vi "TLB Native Dynamic Events ver 0.21.vi"() -> ()   [LabVIEW 2018]
uses:
  Labview Training Phase 2/Enum Controls/States for Action Engine.ctl
  TLB Type Definitions/State Type Definitions, for 0.26d versions and later.ctl
  TLB Type Definitions/Intruction Type Definitions.ctl
  TLB Type Definitions/Encoder cluster.ctl
  TLB Type Definitions/PING CLUSTER.ctl
  <vilib>/Studica/Studica Toolkit/NavX/NavX.lvlib
  <vilib>/Studica/Studica Toolkit/Background/DIO Channel.ctl
  Underlying VI's/NavX VI/navX type def.ctl
  <vilib>/Studica/Studica Toolkit/Background/I2C Channel.ctl
  TLB Type Definitions/Vision cluster.ctl
  <vilib>/NI_Real-Time Target Support.lvlib
  TLB Type Definitions/Stepper cluster.ctl
  Experimental VI's/Archived VI's/MOTOR CONTROL NO PID Type Def.ctl
  Underlying VI's/I2C Master VI/I2C MASTER Type Def.ctl
  Underlying VI's/I2C Master VI/I2C_MASTER_WRITE_NEW Type Def.ctl
  <vilib>/userdefined/High Color/IMAQdx.ctl
  Underlying VI's/I2C Master VI/Arduino_Interfacing.ctl
  TLB Type Definitions/Yaw Cluster.ctl
  TLB Type Definitions/Time cluster.ctl
  TLB Type Definitions/Y Stepper cluster.ctl
  Underlying VI's/Modified webcam FGV/Webcam AE.ctl
  Underlying VI's/Elasped Timer/Elapsed timer control.ctl
  Underlying VI's/Motor Control VI with PID/MOTOR CONTROL WITH PID AE DATA MODE TYPE DEF.ctl
  Underlying VI's/Motor Control VI with PID/MOTOR CONTROL WITH PID AE DIRECTION TYPE DEF.ctl
  TLB Type Definitions/IR Sensor Type Def.ctl
  <vilib>/myRIO/Common/Instrument Driver Framework/myRIO v1.0/AI/typedefs/AI Channels Enum.ctl
  <vilib>/myRIO/Common/Instrument Driver Framework/myRIO v1.0/AI/typedefs/AI Channels List.ctl
  TLB Type Definitions/Motor Speed Cluster.ctl
  Underlying VI's/IMAQ Create Reference AE/IMAQ Reference AE.ctl
  TLB Type Definitions/Line Sensor Cluster.ctl
  Underlying VI's/Line Sensor AE/Line Sensor AE Type Def.ctl
  <vilib>/Utility/RT CPU Load.ctl
  <vilib>/Studica/Studica Toolkit/NavX/TypeDefs/Flags/Z900_navX_Flags_CalibrationStatusTypeDef.ctl
  <vilib>/Studica/Studica Toolkit/NavX/TypeDefs/Flags/Z900_navX_Flags_OpStatusTypeDef.ctl
panel:
  out "Selected Task":T1=enum."Start Task 9"
  out "Object recognition mode":enum16{"Ball", "Soap", "Gel", "Pipe", "None"}(ring)
  out "Distance reached?":bool
  out "Correcte stepper":u8
  out "Image Processing Error":errorcluster
  out "Object Detection":T2
  out "Status":T5 {"OP Status" items=["INITIALIZING", "SELFTEST_IN_PROGRESS", "ERROR", "IMU_AUTOCAL_IN_PROGRESS", "NORMAL"]; "Calibration Status" items=["IMU_CAL_STATE_MASK"=3, "IMU_CAL_STATE_INPROGRESS"=0, "IMU_CAL_STATE_ACCUMULATE"=1, "IMU_CAL_STATE_COMPLETE"=2]}
  out "General Errors":errorcluster
  in  "Red LED":bool
  out "Arm IR Sensor":dbl
  out "Table obstruct":bool
  out "x-y":dbl
  out "Left IR Sensor":dbl
  out "Obstacle detected":bool
  out "Speed & distance":T6
  out "Time up flag":bool
  out "Task selection":u8
  out "NavX Readings":T7
  out "Arduino Data":T8
  out "CPU loads":T9[](array[typedef]) {"ISR (%)" format="%#.2f"; "Idle (%)" format="%#.2f"; "Background (%)" format="%#.2f"; "Normal (%)" format="%#.2f"; "Above Normal (%)" format="%#.2f"; "High (%)" format="%#.2g"; "Timed Structures (%)" format="%#.2g"; "Time Critical (%)" format="%#.2g"; "Total (%)" format="%#.2g"}
  out "TASK ENABLE":bool
  out "Rising Edge":bool
  in  "Green LED":bool
  out "State Logic":T10=enum."Startup"
  out "elements":T1[](array[typedef])
  in  "STOP TASK":bool
  in  "OK Button":bool
  in  "STOP":bool
  out "Queue Errors":errorcluster
  out "Action Queue Items":i32
  out "State Logic Queue Items":i32
  out "Action Queues items":string[](array[string])=["Hardware reset", "Software reset", ""]
  out "Action State":string
  # "System Health Status Update"
  # "VISION"
  # "TLB FRAMEWORK STATUS"
  # "Test Programme written by Calvin Loke    Dated: 28 Aug 2019\nTest Programme revised by Dr Alex See   Dated 30 Aug 2019\n\nRevision date: 20/03/2020\nProgramme version:   TLB Native Dynamic Events ver 0.19a"
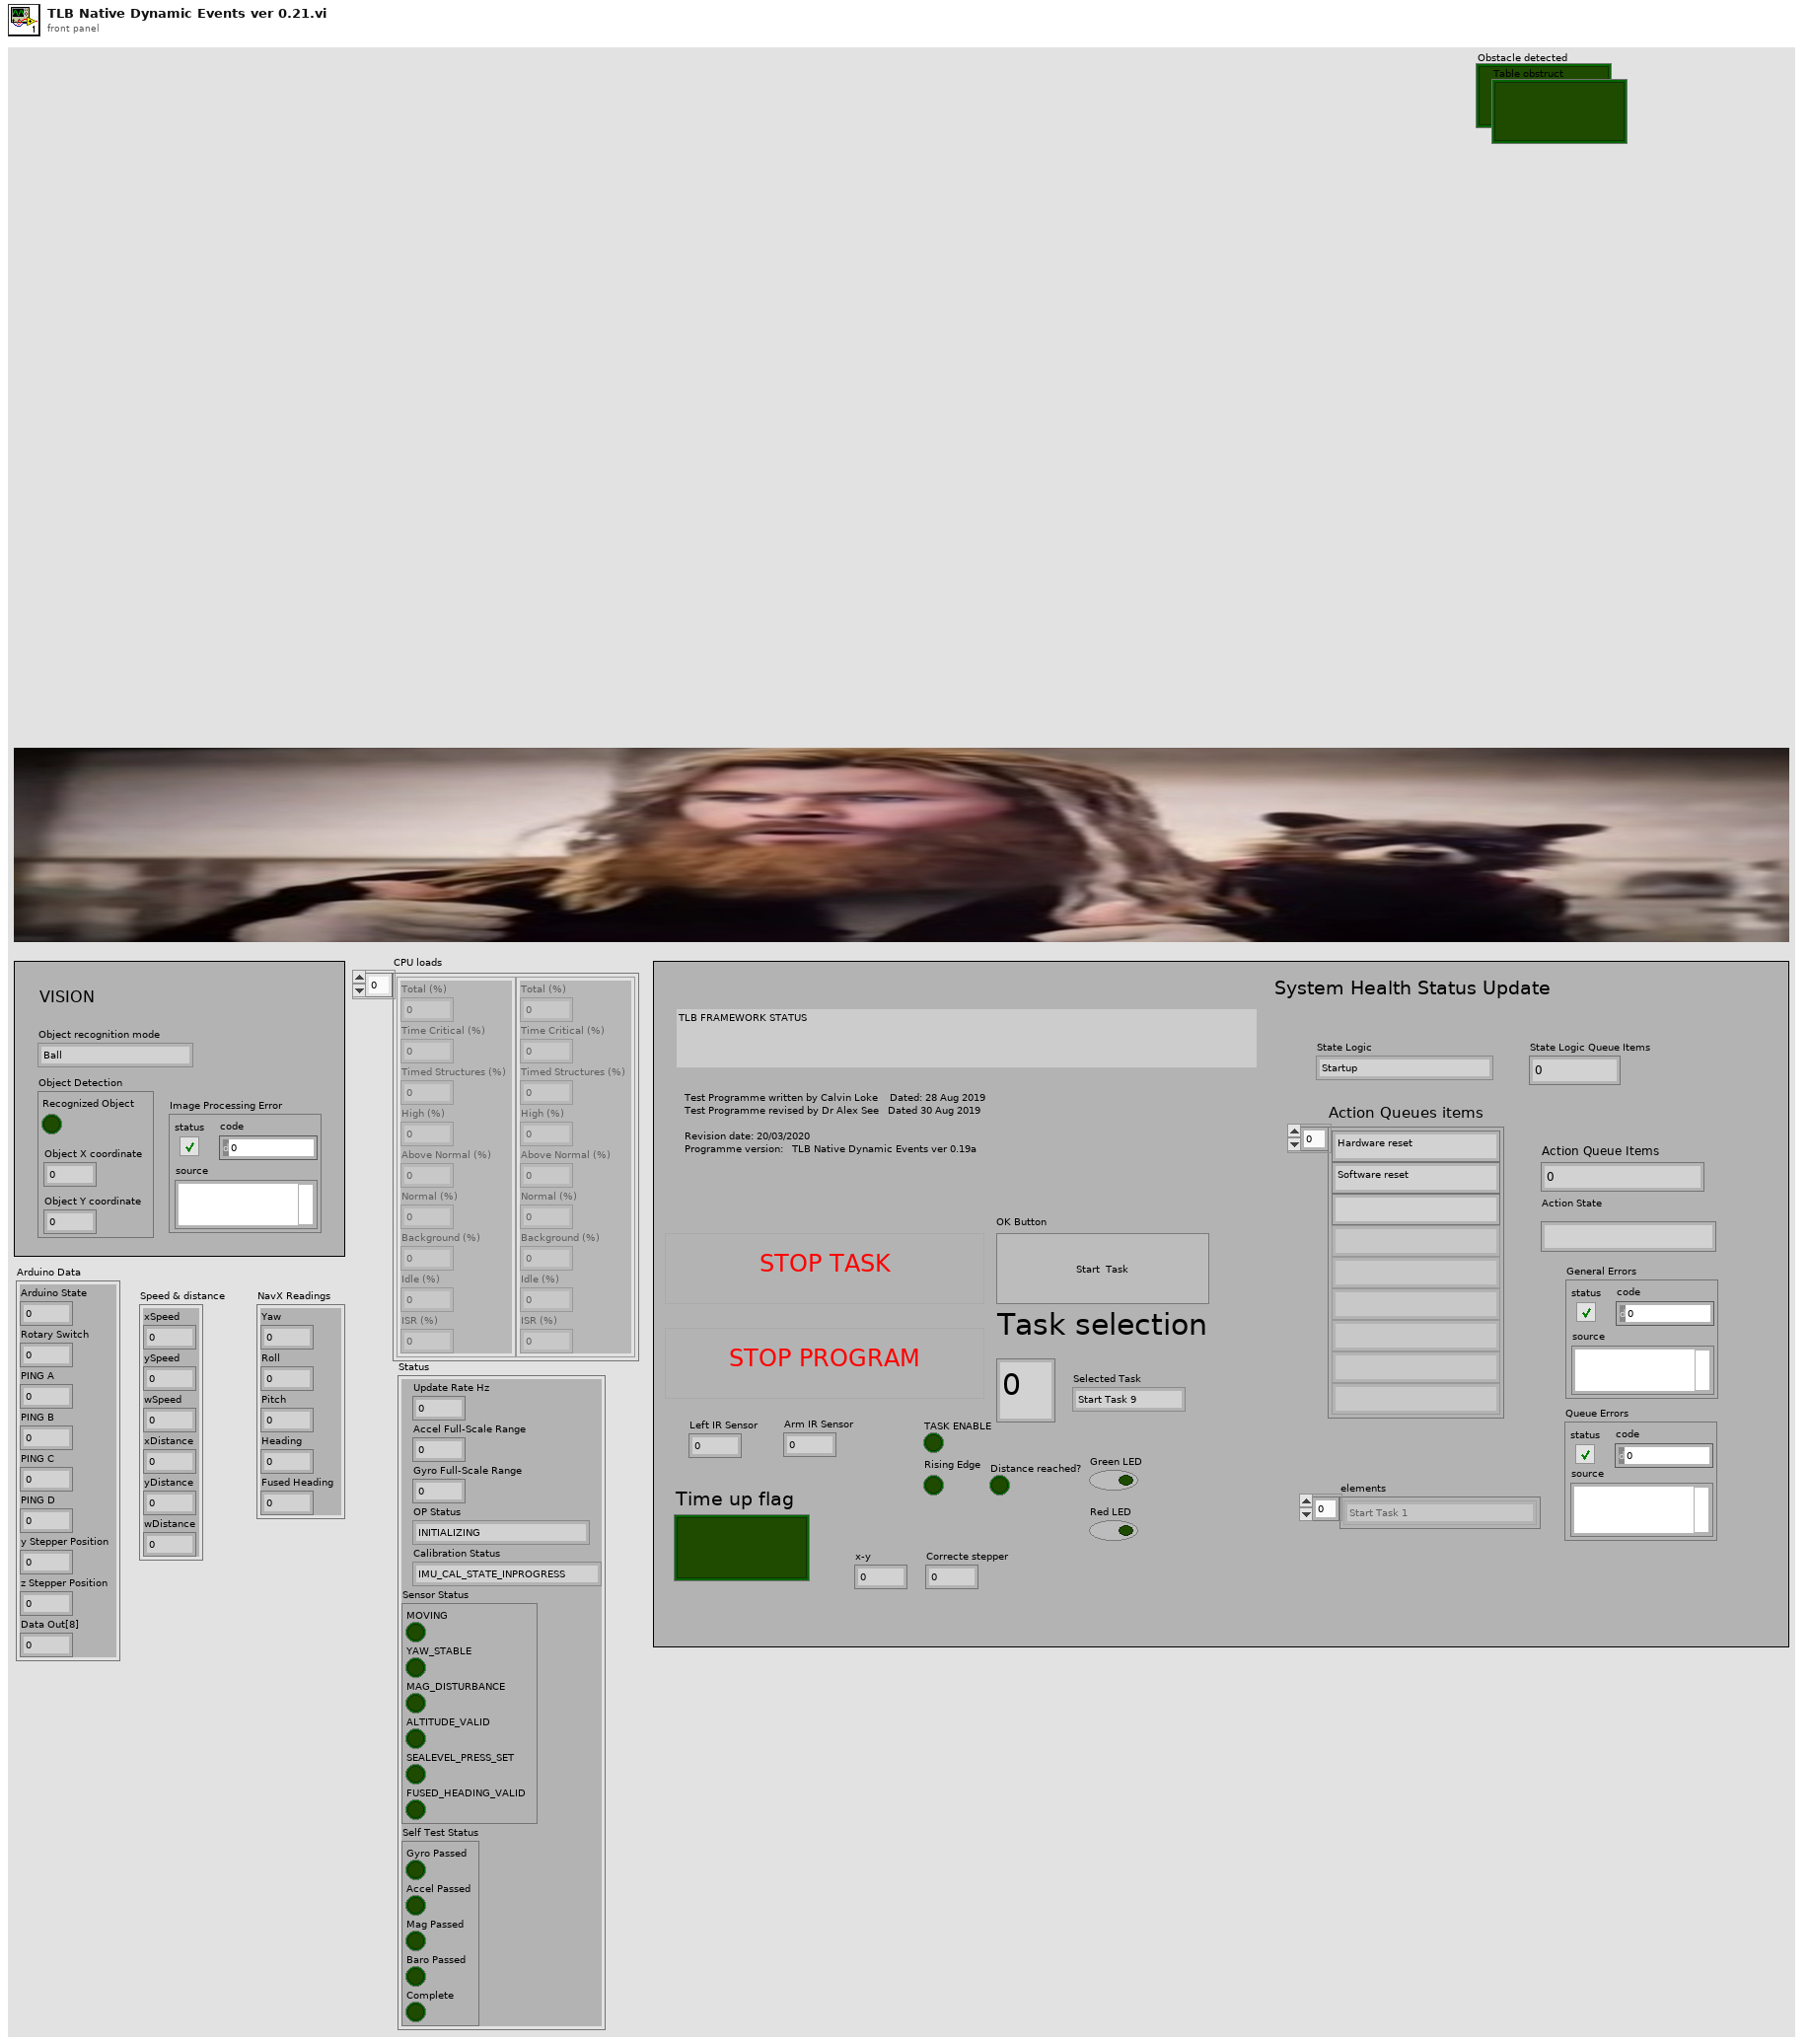
[diagram p1: front panel]
types:
  T1 = typedef "Intruction Type Definitions.ctl" = enum16{"None", "Start Task 1", "Start Task 2", "Start Task 3", "Start Task 4", "Start Task 5", "Start Task 6", "Start Task 7", "Start Task 8 - BALL", "Start Task 8 - Gel", "Start Task 8 - Pipe", "Start Task 8 - Soap", "Start Task 9", "Start Task A", "Start Task B", "Exit"}
  T2 = typedef "Vision cluster.ctl" = cluster{"Recognized Object":bool, "Object X coordinate":dbl, "Object Y coordinate":dbl}
  T3 = typedef "NavX.lvlib/Z900_navX_Flags_OpStatusTypeDef.ctl" = u8
  T4 = typedef "NavX.lvlib/Z900_navX_Flags_CalibrationStatusTypeDef.ctl" = u8
  T5 = cluster{"Update Rate Hz":u8, "Accel Full-Scale Range":u8, "Gyro Full-Scale Range":u16, "OP Status":T3, "Calibration Status":T4, "Sensor Status":cluster{"MOVING":bool, "YAW_STABLE":bool, "MAG_DISTURBANCE":bool, "ALTITUDE_VALID":bool, "SEALEVEL_PRESS_SET":bool, "FUSED_HEADING_VALID":bool}, "Self Test Status":cluster{"Gyro Passed":bool, "Accel Passed":bool, "Mag Passed":bool, "Baro Passed":bool, "Complete":bool}}
  T6 = cluster{"xSpeed":dbl, "ySpeed":dbl, "wSpeed":dbl, "xDistance":dbl, "yDistance":dbl, "wDistance":dbl}
  T7 = cluster{"Yaw":dbl, "Roll":dbl, "Pitch":dbl, "Heading":dbl, "Fused Heading":dbl}
  T8 = cluster{"Arduino State":u8, "Rotary Switch":u8, "PING A":u8, "PING B":u8, "PING C":u8, "PING D":u8, "y Stepper Position":u8, "z Stepper Position":u8, "Data Out[8]":u8}
  T9 = typedef "NI_Real-Time Target Support.lvlib/RT CPU Load.ctl" = cluster{"Total (%)":dbl, "Time Critical (%)":dbl, "Timed Structures (%)":dbl, "High (%)":dbl, "Above Normal (%)":dbl, "Normal (%)":dbl, "Background (%)":dbl, "Idle (%)":dbl, "ISR (%)":dbl}
  T10 = typedef "State Type Definitions.ctl" = enum16{"None", "Startup", "Move to Angle", "True Stop", "Idle", "Shutdown", "Task 1A", "Task 1B", "Task 2:Raise Arm", "Task 2:Sensor Mode", "Task 2:Reverse Mode", "Task 3", "Task 4_A", "Task 4_B", "Task 4_C", "Task 4_D", "Task 5A", "Task 5B", "Task 5C", "Task 5D", "Task 5E: POSITION ARM", "Task 5F: ARM GRAB HEIGHT", "Task 5G: CLOSE CLAW", "Task 5H: RAISE ARM", "Task 6_A", "Task 6_B", "Task 7", "Task 8A: RAISE ARM", "Task 8B: MOVE TO BOX", "Task 8C: CAM BURST", "Task 8D: PROCESS IMAGE", "Task 8E: ROBOT ADJUST", "Task 8F: CAM BURST 2", "Task 8G: PROCESS IMAGE 2", "Task 8H: ARM ADJUST", "Task 8I: ARM GRAB HEIGHT", "Task 8J: CLOSE CLAW", "Task 8K: RAISE MY SWORD", "Task 9A: Raise Arm", "Task 9B: Rotate to Angle", "Task 9C: Detect Box", "Task 9D: MOVE FORWARD", "Task 9E: MOVE LEFT", "Task 9F: SCAN IMAGE", "Task 9G: PROCESS COLOUR", "Task 9H: MOVE RIGHT", "Task 9I: SCAN IMAGE", "Task 9J: PROCESS COLOUR", "Task 9K: ROTATE 90 CW", "Task 9L: MOVE FORWARD", "Task 9M: MOVE RIGHT", "Task 9N: SCAN IMAGE", "Task 9O: PROCESS COLOUR", "Task 9P: MOVE RIGHT", "Task 9Q: SCAN IMAGE", "Task 9R: PROCESS COLOUR", "Task A1: Raise Arm", "Task A2: Rotate to Angle", "Task A3: Move Forward", "Task A4: Rotate CW 90"}
  T11 = typedef "Line Sensor Cluster.ctl" = cluster{"Line Detected?":bool, "S1":dbl, "S2":dbl, "S3":dbl, "S4":dbl}
  T12 = typedef "Motor Speed Cluster.ctl" = cluster{"ySpeed":dbl, "xSpeed":dbl, "wSpeed":dbl}
  T13 = typedef "IR Sensor Type Def.ctl" = cluster{"Left IR Sensor":dbl, "Arm IR Sensor":dbl, "Bottom IR Sensor":dbl}
  T14 = typedef "Y Stepper cluster.ctl" = cluster{"yStepper desired":u8}
  T15 = typedef "Time cluster.ctl" = cluster{"Time up flag":bool, "SET TIME TO CHECK":dbl}
  T16 = typedef "Yaw Cluster.ctl" = cluster{"Yaw":dbl, "Compass":dbl}
  T17 = typedef "Stepper cluster.ctl" = cluster{"y Stepper Position":u8, "z Stepper Position":u8}
  T18 = typedef "DIO Channel.ctl" = enum16{"Not Connected", "A/DIO1", "A/DIO2", "A/DIO3", "A/DIO4", "A/DIO5", "A/DIO6", "A/DIO7", "A/DIO13", "B/DIO1", "B/DIO2", "B/DIO3", "B/DIO4", "B/DIO5", "B/DIO6", "B/DIO7", "B/DIO13", "C/DIO0", "C/DIO1", "C/DIO2", "C/DIO3", "C/DIO4", "C/DIO5", "C/DIO6", "C/DIO7"}
  T19 = typedef "PING CLUSTER.ctl" = cluster{"PING_A":u8, "PING_B":u8, "PING_C":u8, "PING_D":u8}
  T20 = typedef "Encoder cluster.ctl" = cluster{"xDistance":dbl, "yDistance":dbl, "wDistance":dbl}
  T21 = cluster{"DIO Channel":T18, "FPGA VI Reference Out":refnum<k20>}
  T22 = typedef "navX type def.ctl" = enum16{"Get i2C reference", "Read Values", "Zero Yaw"}
  T23 = typedef "Arduino_Interfacing.ctl" = enum16{"Initialize", "Write to Arduino", "Read From Arduino"}
  T24 = typedef "I2C Channel.ctl" = enum16{"Not Connected", "A", "B"}
  T25 = typedef "States for Action Engine.ctl" = enum16{"Initialize", "Write", "Read"}
  T26 = cluster{"I2C Ref Out":cluster{"I2C Channel":T24, "FPGA VI Reference Out":refnum<k20>}, "Connected":bool, "Slave Address (7-bit)":u8, "Registry":u8[]}
  T27 = typedef "State Type Definitions.ctl" = enum16{"None", "Startup", "Move to Angle", "True Stop", "Idle", "Shutdown", "Task 1", "Task 2:Raise Arm", "Task 2:Sensor Mode", "Task 2:Reverse Mode", "Task 3", "Task 4_A", "Task 4_B", "Task 4_C", "Task 4_D", "Task 5A: ARM CAM HEIGHT", "Task 5B: MOVE TO BOX", "Task 5C: CAM BURST", "Task 5D: PROCESS IMAGE", "Task 5E: POSITION ARM", "Task 5F: ARM GRAB HEIGHT", "Task 5G: CLOSE CLAW", "Task 5H: RAISE ARM", "Task 6_A", "Task 6_B", "Task 7", "Task 8A: RAISE ARM", "Task 8B: MOVE TO BOX", "Task 8C: CAM BURST", "Task 8D: PROCESS IMAGE", "Task 8E: ROBOT ADJUST", "Task 8F: CAM BURST 2", "Task 8G: PROCESS IMAGE 2", "Task 8H: ARM ADJUST", "Task 8I: ARM GRAB HEIGHT", "Task 8J: CLOSE CLAW", "Task 8K: RAISE MY SWORD", "Task 9A: Raise Arm", "Task 9B: Rotate to Angle", "Task 9C: Rotation alignmnet", "Task 9D: Move Forward", "Task 9E: MOVE LEFT", "Task A: RAISE ARM TO HEIGHT", "Task A: MOVE FORWARD"}
  T28 = typedef "MOTOR CONTROL WITH PID AE DIRECTION TYPE DEF.ctl" = enum16{"y-axis movement", "x-axis movement", "rotation", "stop", "reset encoders"}
  T29 = typedef "MOTOR CONTROL WITH PID AE DATA MODE TYPE DEF.ctl" = enum16{"Init AE", "Write to AE", "Read from AE"}
  T30 = typedef "Line Sensor AE Type Def.ctl" = enum16{"INIT AE", "READ FROM LINE SENSORS"}
  T31 = typedef "IMAQ Reference AE.ctl" = enum16{"Initialize AE", "Get IMAQ Reference", "Dispose Processing Buffer"}
  T32 = typedef "Elapsed timer control.ctl" = enum16{"Start", "Pause", "Initialize"}
  T33 = typedef "I2C_MASTER_WRITE_NEW Type Def.ctl" = enum16{"Ultrasonic sensors", "Stepper origin", "zStepper 13.3k", "zStepper 13k", "zStepper 12k", "zStepper 11k", "zStepper 10k", "zStepper 9k", "zStepper 8k", "zStepper 7k", "zStepper 6k", "zStepper 5k", "zStepper 4k", "zStepper 3k", "zStepper 2k", "zStepper 1k", "zStepper 900", "zStepper 800", "zStepper 700", "zStepper 600", "zStepper 500", "zStepper 400", "zStepper 300", "zStepper 200", "zStepper 100", "zStepper 0", "yStepper control", "Open Claw", "Close Claw", "Soft Reset"}
  T34 = typedef "Webcam AE.ctl" = enum16{"Initialize Camera", "Open Camera", "Continuous Acquisition", "Close Camera", "Retrieve Image", "Dispose Camera Image Buffer"}
  T35 = typedef "IMAQdx.ctl" = refnum<k21>
  T36 = typedef "MOTOR CONTROL NO PID Type Def.ctl" = enum16{"Init", "Front Back", "Left Right", "Rotate", "Stop", "Latch"}
  T37 = typedef "AI Channels List.ctl" = T38[]
  T38 = typedef "AI Channels Enum.ctl" = enum16{"Not Connected", "AudioIn/Left", "AudioIn/Right", "C/AI0", "C/AI1", "A/AI0", "A/AI1", "A/AI2", "A/AI3", "A/AI4", "A/AI5", "A/AI6", "A/AI7", "B/AI0", "B/AI1", "B/AI2", "B/AI3", "B/AI4", "B/AI5", "B/AI6", "B/AI7", "AI/AI0", "AI/AI1", "AI/AI2", "AI/AI3", "A/AI0 (DIFF)", "A/AI1 (DIFF)", "A/AI2 (DIFF)", "A/AI3 (DIFF)", "B/AI0 (DIFF)", "B/AI1 (DIFF)", "B/AI2 (DIFF)", "B/AI3 (DIFF)"}
  T39 = cluster{"S1":dbl, "S2":dbl, "S3":dbl, "S4":dbl, "Array[4]":dbl, "Array[5]":dbl, "Array[6]":dbl, "Array[7]":dbl, "Array[8]":dbl}
  T40 = typedef "I2C MASTER Type Def.ctl" = enum16{"Last State", "Mode 0", "Mode 1", "Mode 2", "Mode 3", "Mode 4", "Mode 5", "Mode 6", "Mode 7", "Mode 8", "Mode 9", "Mode 10"}
  T41 = typedef "IMAQ Image.ctl" = refnum<image>
  T42 = cluster{"Number of Matches":i32, "Object detected?":bool}
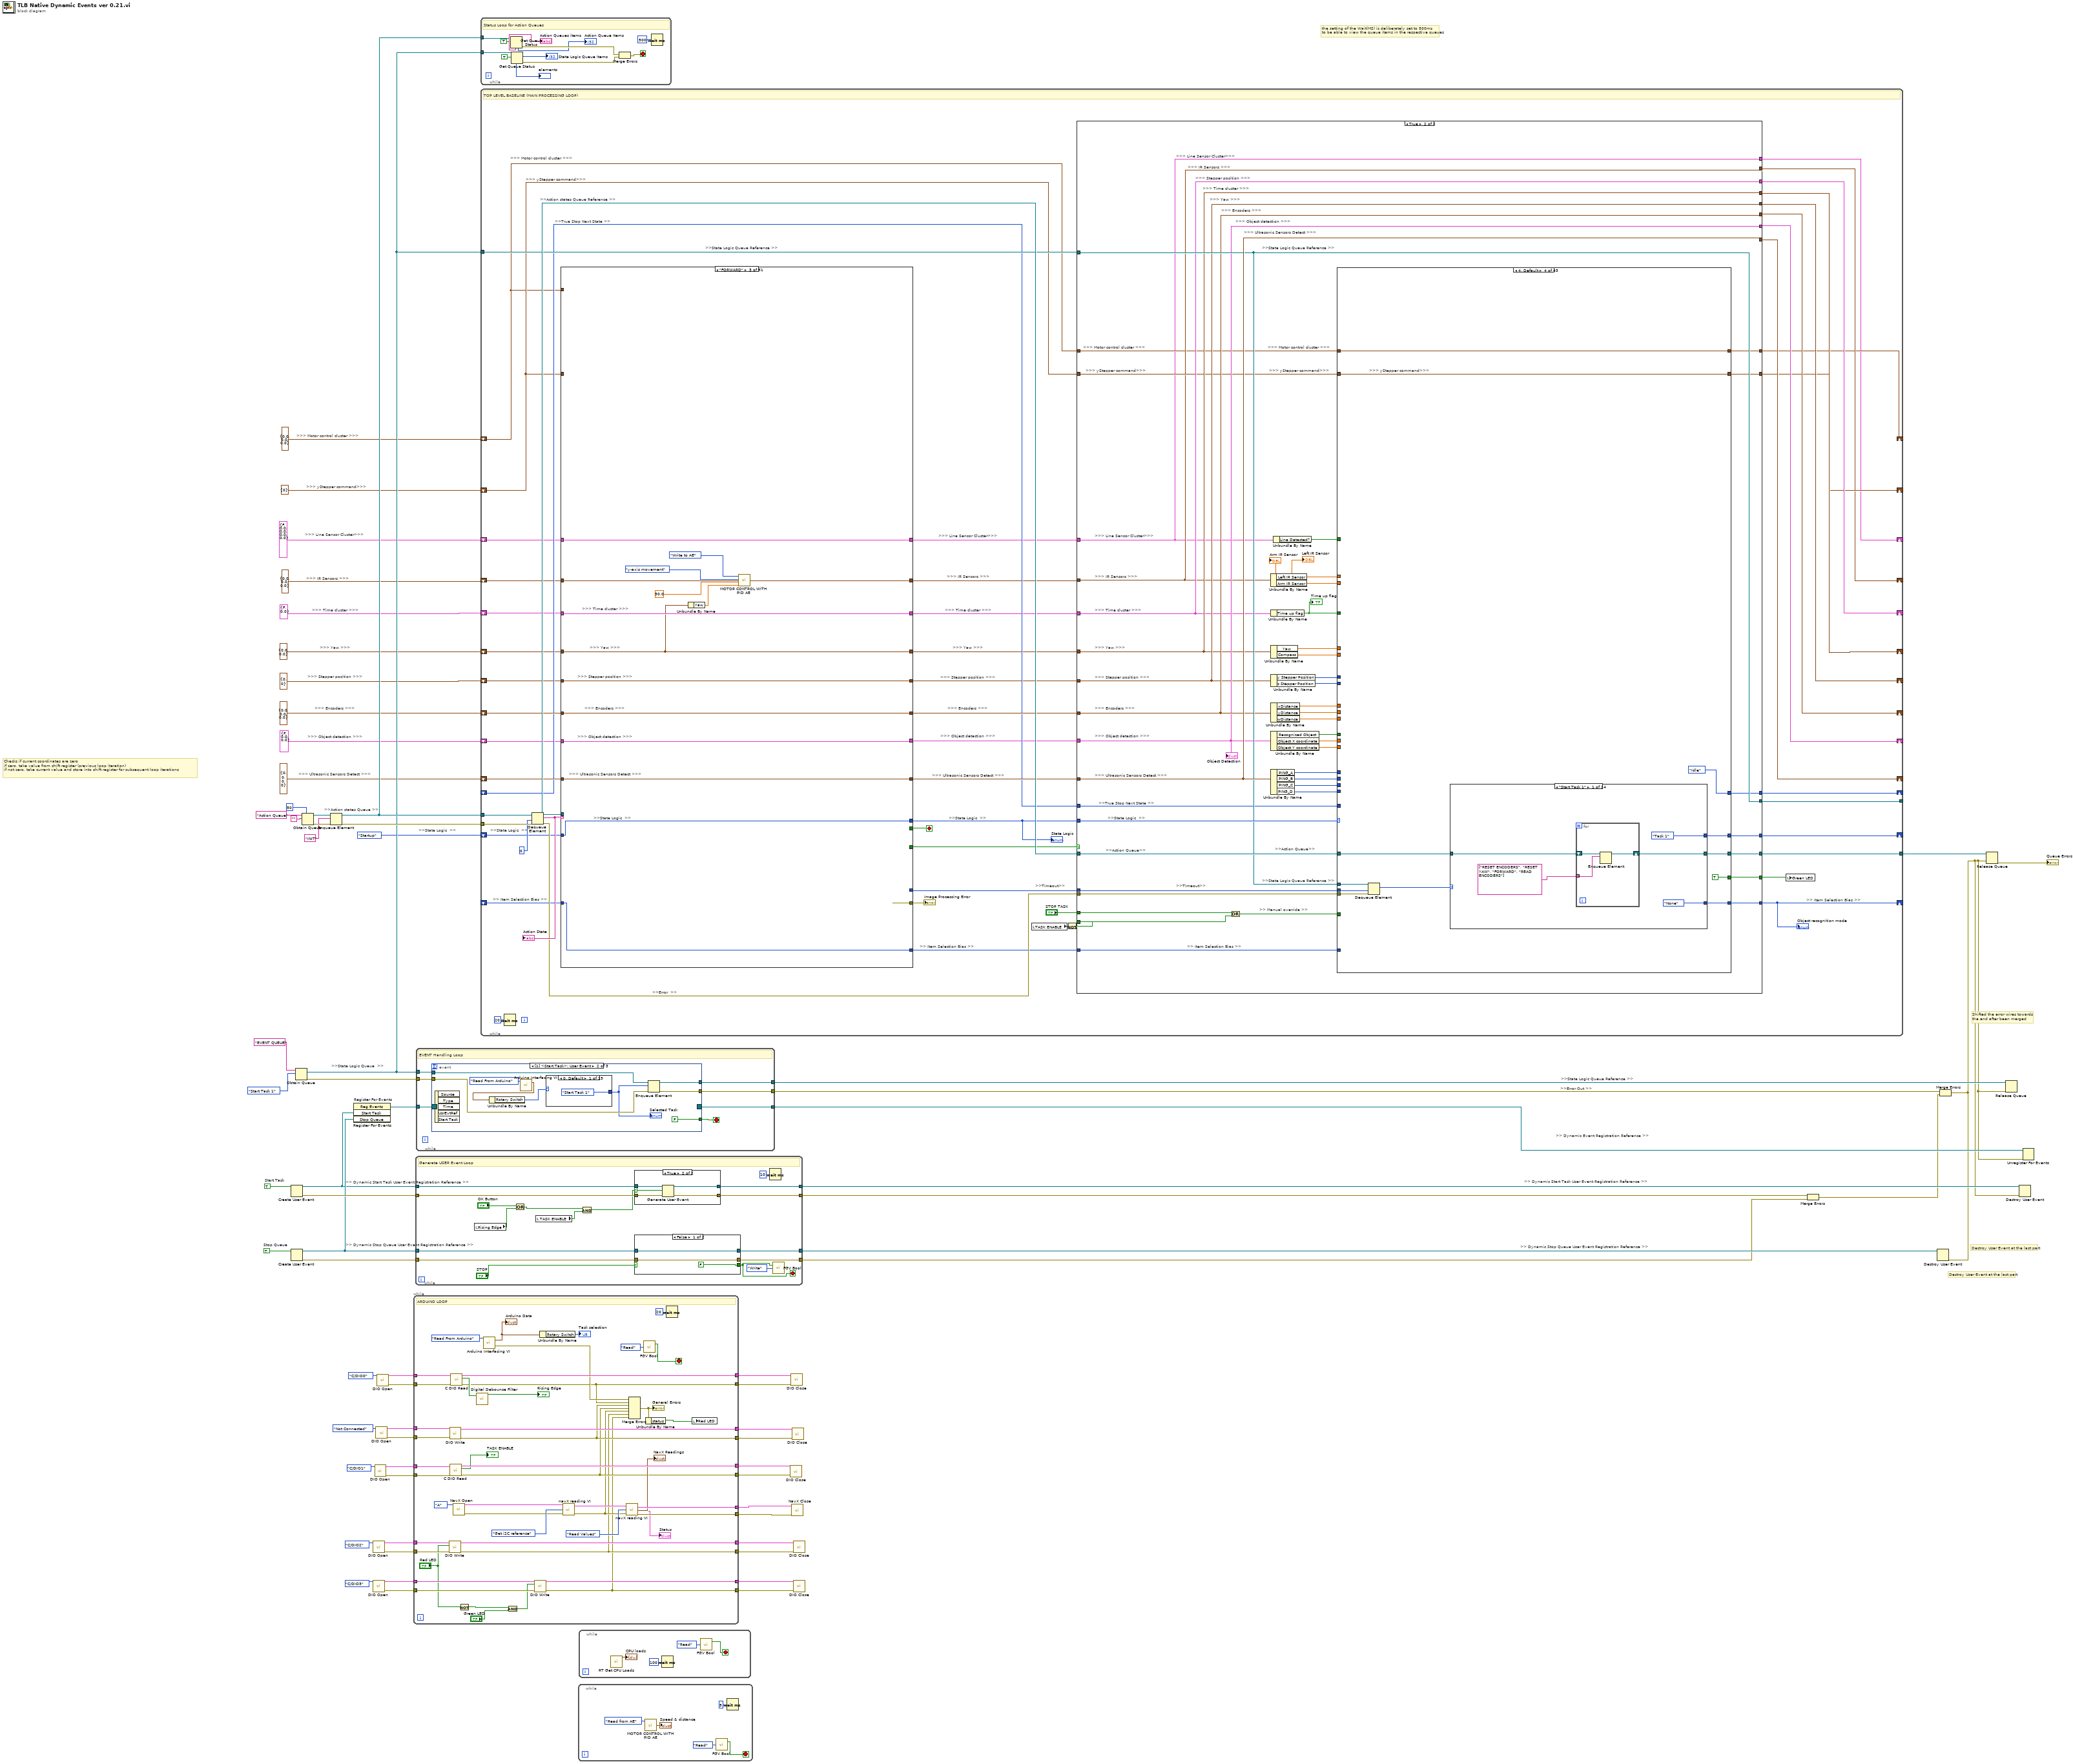
[diagram p0: block diagram]
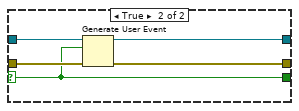
[diagram p2: hidden frame]
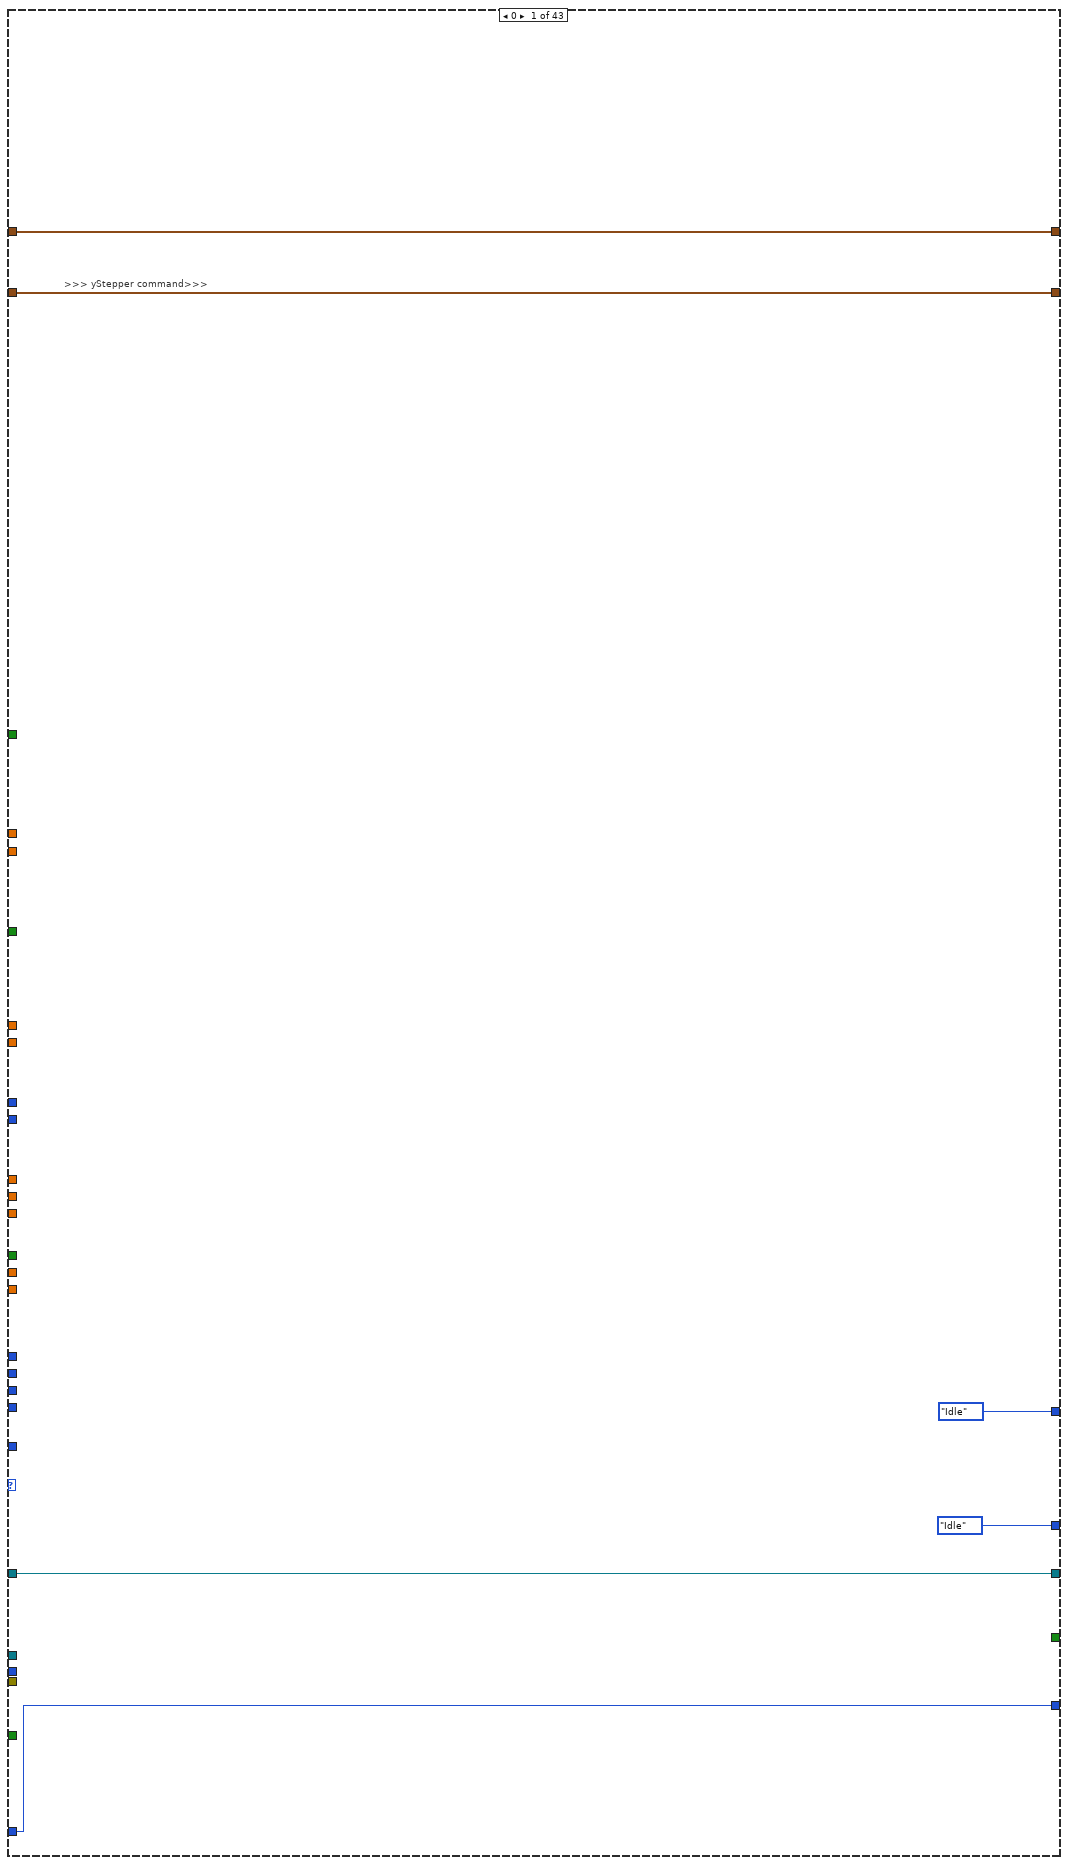
[diagram p5: hidden frame]
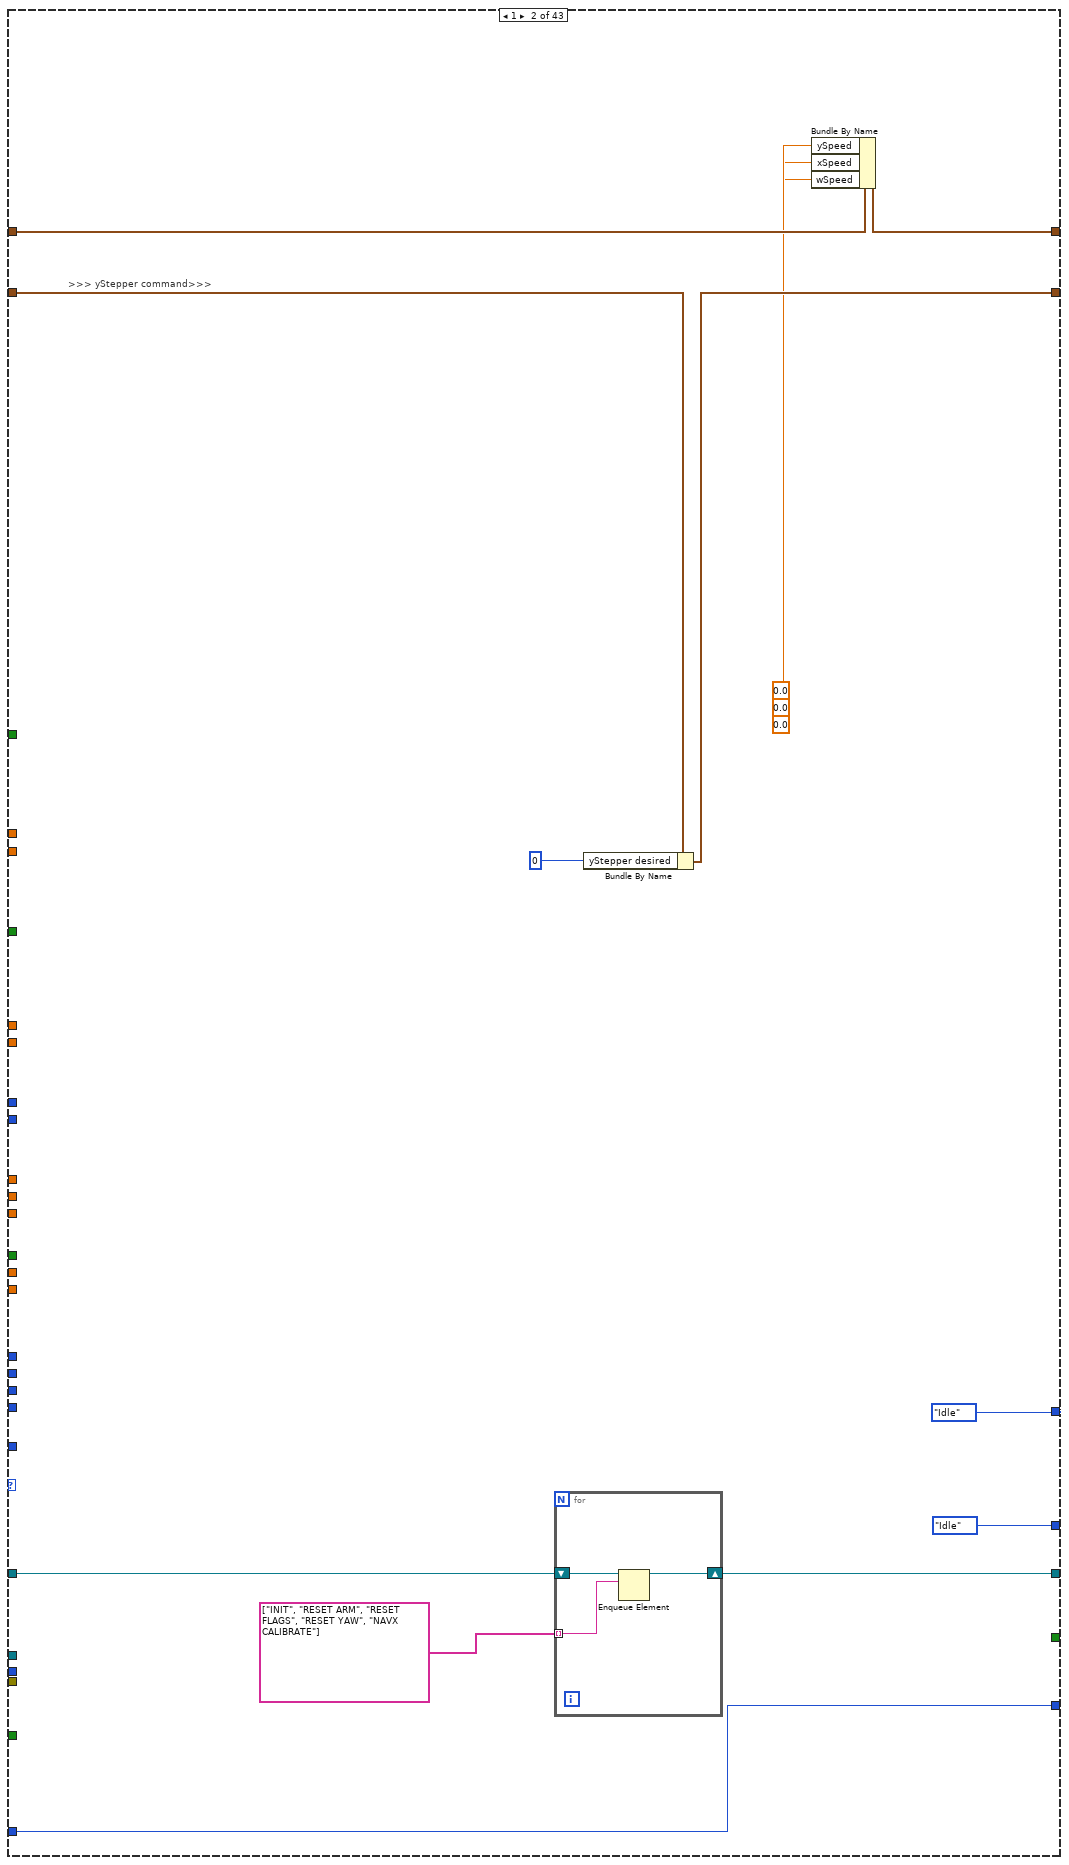
[diagram p6: hidden frame]
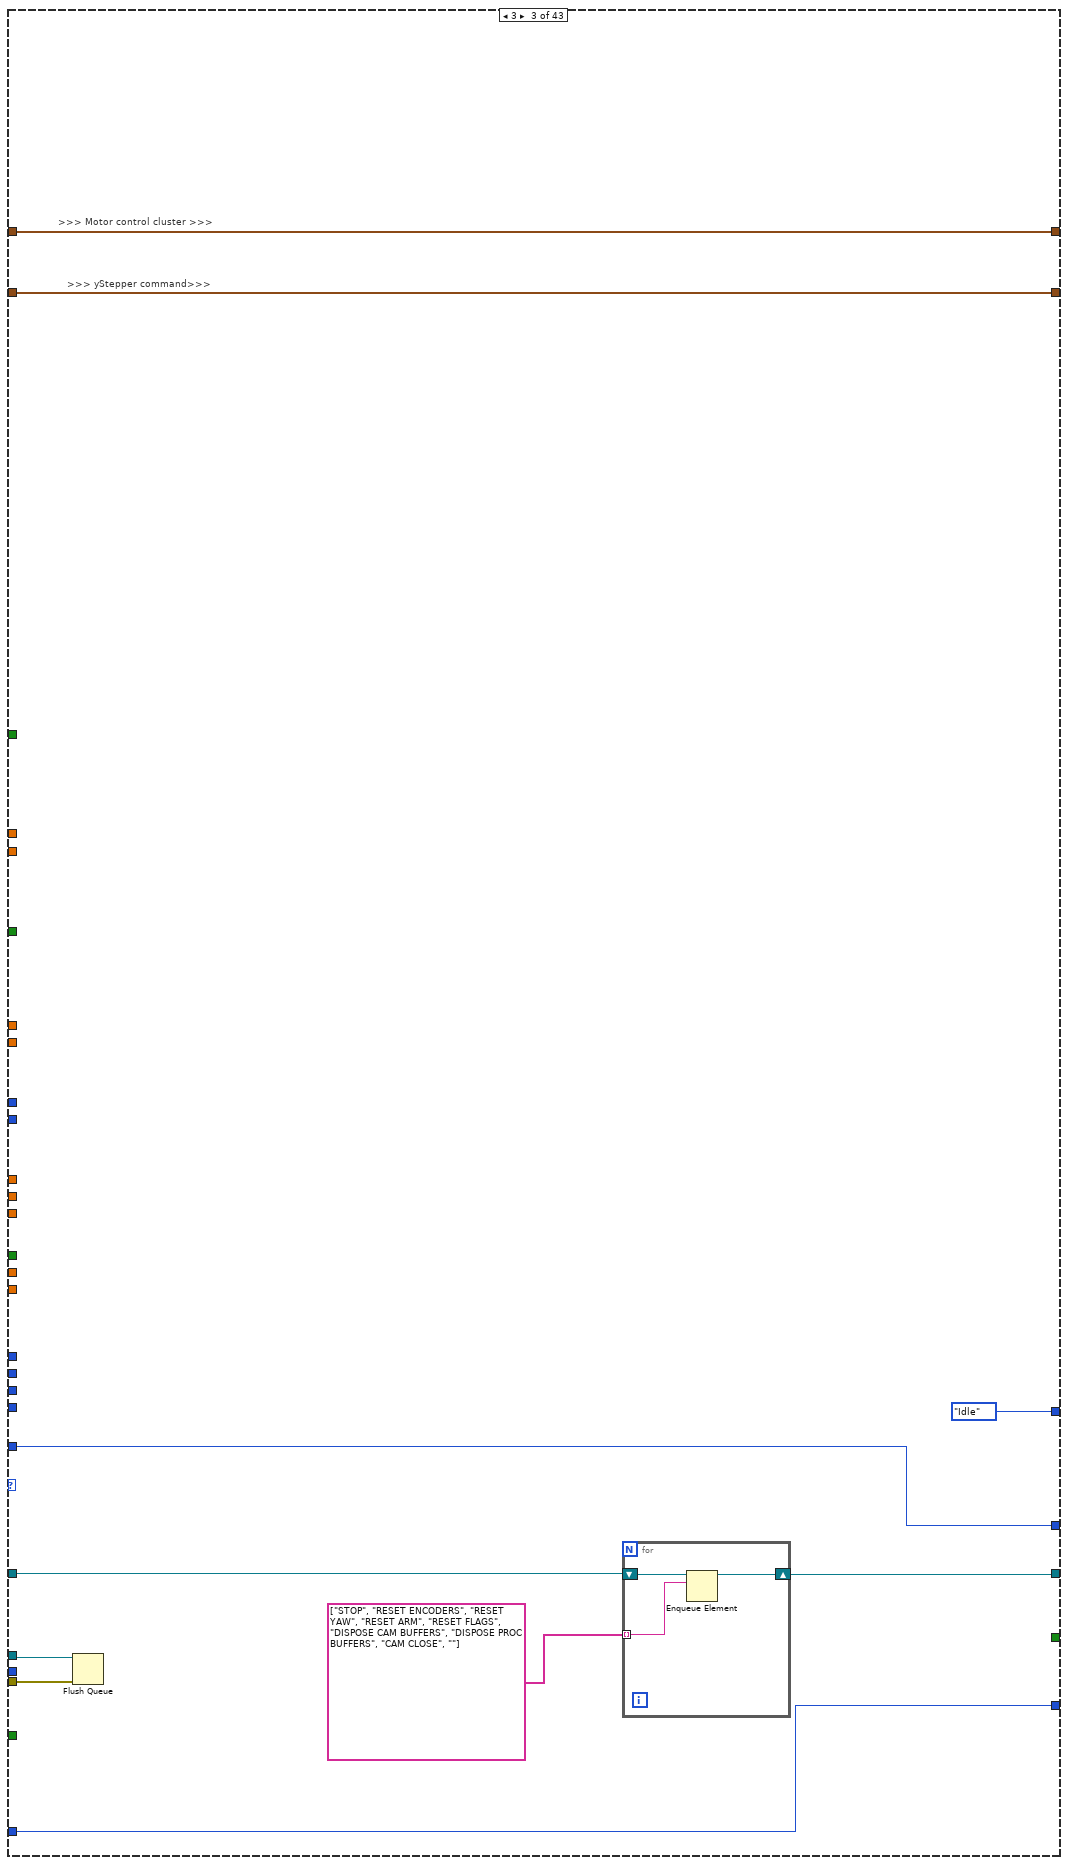
[diagram p7: hidden frame]
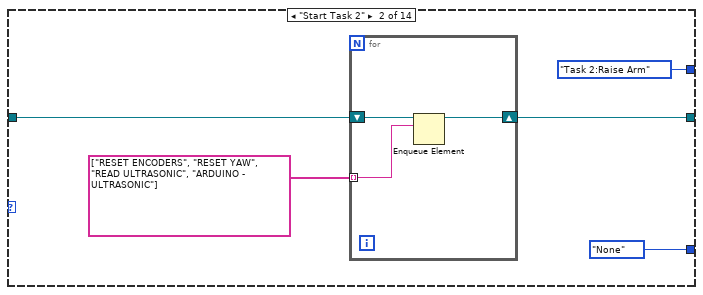
[diagram p8: hidden frame]
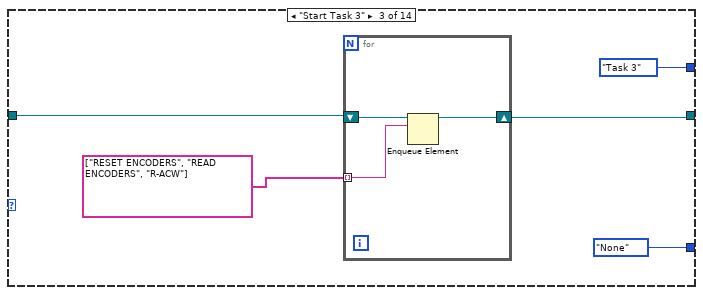
[diagram p9: hidden frame]
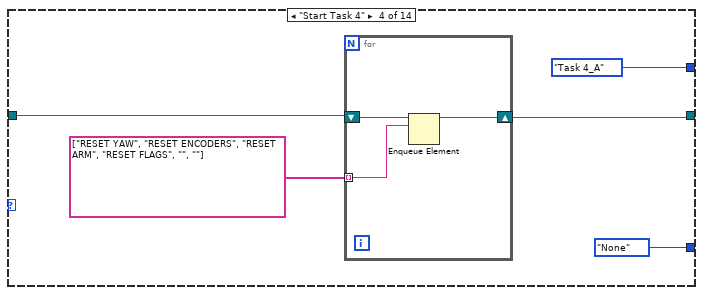
[diagram p10: hidden frame]
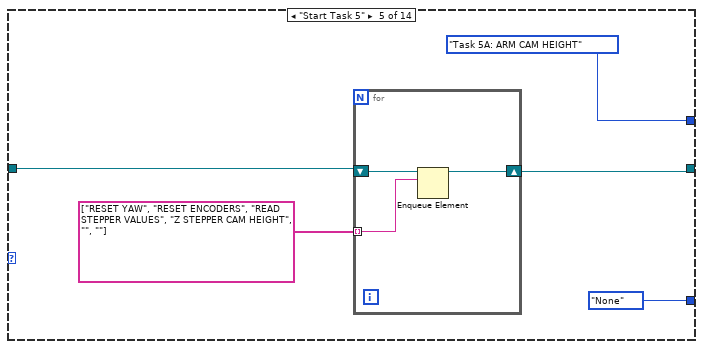
[diagram p11: hidden frame]
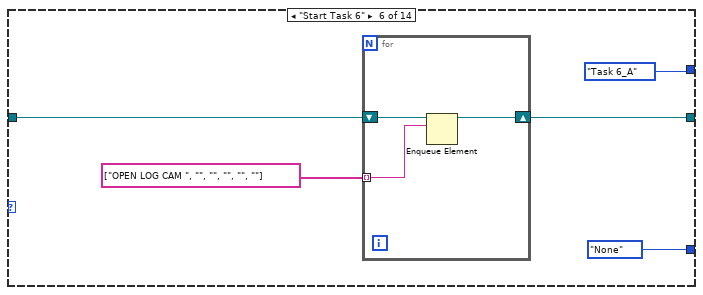
[diagram p12: hidden frame]
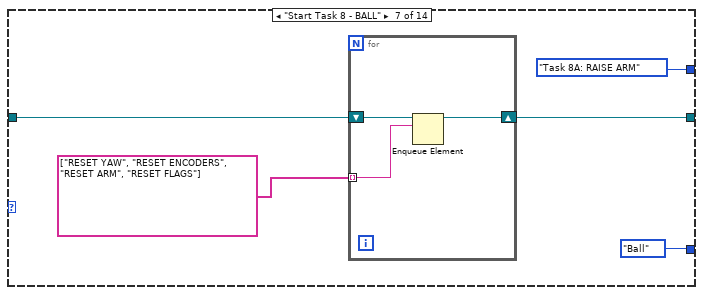
[diagram p13: hidden frame]
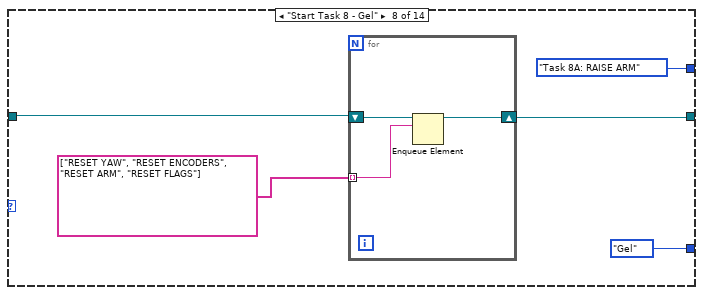
[diagram p14: hidden frame]
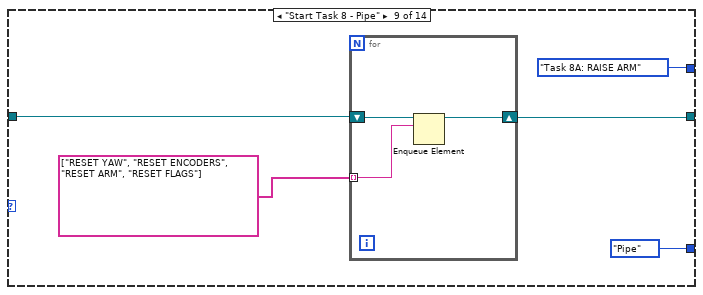
[diagram p15: hidden frame]
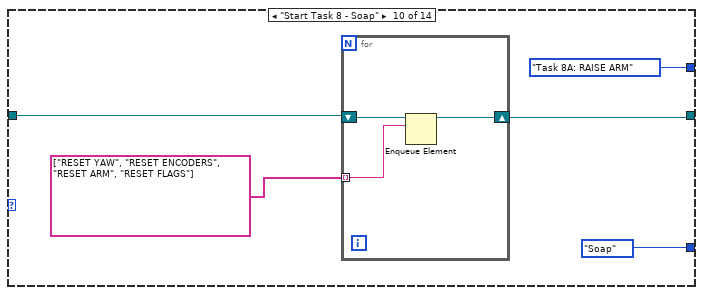
[diagram p16: hidden frame]
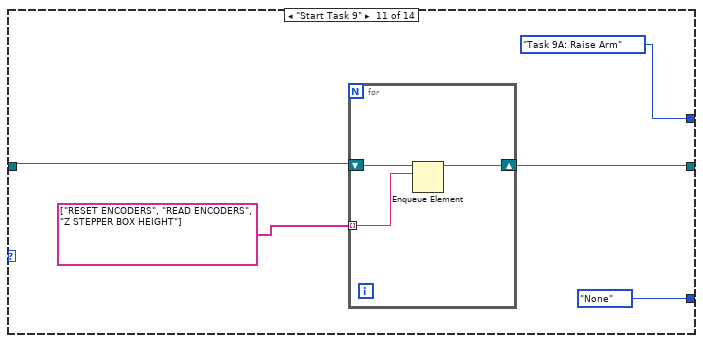
[diagram p17: hidden frame]
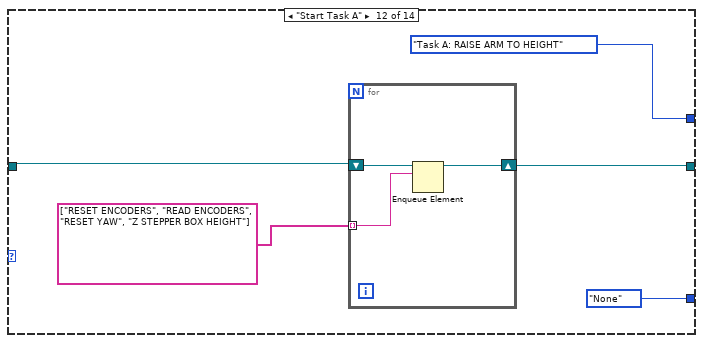
[diagram p18: hidden frame]
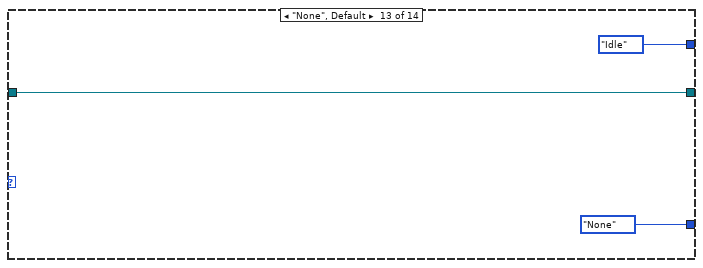
[diagram p19: hidden frame]
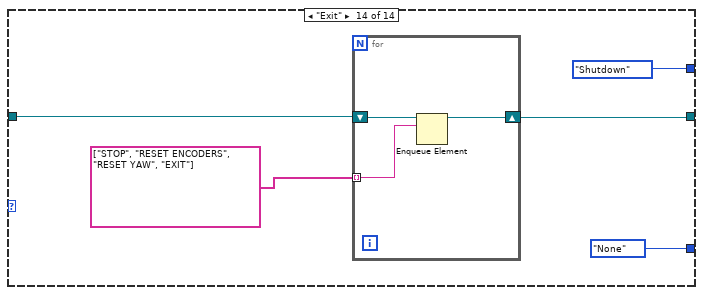
[diagram p20: hidden frame]
diagram:
  w68 = TRUE  # Stop Queue
  w67 = TRUE  # Start Task
  # ">>State Logic  >>"
  # ">>> Line Sensor Cluster>>>"
  # ">>> Motor control cluster >>>"
  # ">>> IR Sensors >>>"
  # "Checks if current coordinates are zero\nif zero, take value from shift register (previous loop iteration)\nif not zero, take current value and store into shift register for subsequent loop iterations"
  # ">>> yStepper command>>>"
  # ">>> Time cluster >>>"
  # ">>> Yaw >>>"
  # ">>> Stepper position >>>"
  # ">>> Encoders >>>"
  # ">>> Object detection >>>"
  # ">>> Ultrasonic Sensors Detect >>>"
  # "the setting of the Wait(MS) is deliberately set to 500ms\nto be able to view the queue items in the respective queues"
  # ">>Error Out >>"
  # ">> Dynamic Stop Queue User Event Registration Reference >>"
  # ">> Dynamic Start Task User Event Registration Reference >>"
  # ">> Dynamic Stop Queue User Event Registration Reference >>"
  # ">> Dynamic Start Task User Event Registration Reference >>"
  # ">> Dynamic Event Registration Reference >>"
  # ">>Action states Queue >>"
  # ">>State Logic Queue  >>"
  # ">>State Logic Queue Reference >>"
  # "Destroy User Event at the last part"
  # "Destroy User Event at the last part"
  # "Shifted the error wires towards\nthe end after been merged"
  n1 = Create User Event(user event datatype=w67) -> (user event=w59:refnum<user-event>, error out=w64:errorcluster)  [unwired: 1 in]
  n2 = Create User Event(user event datatype=w68) -> (user event=w60:refnum<user-event>, error out=w63:errorcluster)  [unwired: 1 in]
  n3 = Obtain Queue(name (unnamed)="EVENT QUEUE", element data type=Intruction_Type_Definitions."Start Task 1" ("Enum")) -> (queue out=w45:refnum<queue>, error out=w51:errorcluster)  [unwired: 3 in, 1 out]
  n4 = Obtain Queue(max queue size (-1, unlimited)=50, name (unnamed)="Action Queue", element data type="") -> (queue out=w54:refnum<queue>, error out=w50:errorcluster)  [unwired: 2 in, 1 out]
  n5 = Enqueue Element(queue=w54, element="INIT", error in (no error)=w50) -> (queue out=w46:refnum<queue>, error out=w49:errorcluster)  [unwired: 1 in, 1 out]
  n6 = register-events "Register For Events"(w59, w60) -> (reference out=w58:refnum<event-registration>)  [unwired: 2 in, 1 out]
  n7 = call <vilib>:"DIO Open.vi"("DIO Channel"=DIO_Channel."C/DIO2") -> ("error out"=w18:errorcluster, "DIO Info Out"=w19:T21)  [unwired: 9 in]
  n8 = call <vilib>:"DIO Open.vi"("DIO Channel"=DIO_Channel."C/DIO3") -> ("error out"=w13:errorcluster, "DIO Info Out"=w14:T21)  [unwired: 9 in]
  n9 = call <vilib>:"DIO Open.vi"("DIO Channel"=DIO_Channel."C/DIO1") -> ("error out"=w23:errorcluster, "DIO Info Out"=w24:T21)  [unwired: 9 in]
  n10 = call <vilib>:"DIO Open.vi"("DIO Channel"=DIO_Channel."Not Connected") -> ("error out"=w28:errorcluster, "DIO Info Out"=w30:T21)  [unwired: 9 in]
  n11 = call <vilib>:"DIO Open.vi"("DIO Channel"=DIO_Channel."C/DIO0") -> ("error out"=w33:errorcluster, "DIO Info Out"=w36:T21)  [unwired: 9 in]
  n12 = while {
    tunnel: w36 -> [w112]
    tunnel: [w111] -> w34
    tunnel: w33 -> [w110]
    tunnel: [w81] -> w32
    tunnel: w30 -> [w107]
    tunnel: [w106] -> w29
    tunnel: w28 -> [w105]
    tunnel: [w80] -> w27
    tunnel: [w104] -> w25
    tunnel: w24 -> [w103]
    tunnel: w23 -> [w102]
    tunnel: [w79] -> w22
    tunnel: w19 -> [w96]
    tunnel: w18 -> [w95]
    tunnel: [w94] -> w17
    tunnel: [w77] -> w16
    tunnel: w14 -> [w93]
    tunnel: w13 -> [w92]
    tunnel: [w91] -> w12
    tunnel: [w76] -> w11
    tunnel: [w88] -> w8
    tunnel: [w87] -> w9
    stop <- w114 stop-if-true
    # "ARDUINO LOOP"
    n13 = call <vilib>:"DIO Write.vi"("error in (no error)"=w95, "Input"="Red LED", "DIO Info In"=w96) -> ("error out"=w77:errorcluster, "DIO Info Out"=w94:T21)  [unwired: 7 in]
    n14 = call <vilib>:"DIO Write.vi"("error in (no error)"=w105, "DIO Info In"=w107) -> ("error out"=w80:errorcluster, "DIO Info Out"=w106:T21)  [unwired: 8 in]
    n15 = call <vilib>:"C DIO Read.vi"("error in (no error)"=w102, "DIO Info In in"=w103) -> ("error out"=w79:errorcluster, "IN"=→"TASK ENABLE":bool, "DIO Info In out"=w104:T21)  [unwired: 7 in]
    n16 = call <vilib>:"C DIO Read.vi"("error in (no error)"=w110, "DIO Info In in"=w112) -> ("error out"=w81:errorcluster, "IN"=w109:bool, "DIO Info In out"=w111:T21)  [unwired: 7 in]
    n17 = call <vilib>:"NavX Open.vi"("I2C Channel"=I2C_Channel."A") -> ("error out"=w98:errorcluster, "NavX Info"=w100:T26)  [unwired: 9 in]
    n18 = Not(x="Red LED") -> (.not. x?=w70:bool)
    n19 = call "Digital Debounce Filter.vi"("Boolean input"=w109) -> ("Rising Edge"=→"Rising Edge":bool)  [unwired: 1 in, 2 out]
    n20 = call "Arduino Interfacing VI.vi"("AE Mode"=Arduino_Interfacing."Read From Arduino") -> ("error out"=w82:errorcluster, "Arduino Data"=w84:T8)  [unwired: 3 in]
    "Arduino Data" <- w84
    n21 = And(x=w70, y="Green LED") -> (x .and. y?=w73:bool)
    n22 = call <vilib>:"DIO Write.vi"("error in (no error)"=w92, "Input"=w73, "DIO Info In"=w93) -> ("error out"=w76:errorcluster, "DIO Info Out"=w91:T21)  [unwired: 7 in]
    n23 = Unbundle By Name(w84) -> ("Rotary Switch"=→"Task selection":u8)
    n24 = call "navX reading VI.vi"("NavX Info In"=w100, "Mode"=navX_type_def."Get i2C reference", "error in (no error)"=w98) -> ("NavX Info Out"=w89:T26, "Error Out"=w78:errorcluster)  [unwired: 2 out]
    n25 = call "navX reading VI.vi"("NavX Info In"=w89, "Mode"=navX_type_def."Read Values", "error in (no error)"=w78) -> ("NavX Info Out"=w88:T26, "NavX Readings"=→"NavX Readings":T7, "Status"=→"Status":T5, "Error Out"=w87:errorcluster)
    n26 = Merge Errors(w82, w81, w80, w79, w78, w77, w76) -> (w74:errorcluster)
    "General Errors" <- w74
    n27 = call "FGV Bool.vi"("Init/Read/Write State"=States_for_Action_Engine."Read") -> ("Output node"=w114:bool)  [unwired: 2 in, 1 out]
    n28 = Unbundle By Name(w74) -> ("status"=w71:bool)
    n29 = Wait (ms)(milliseconds to wait=u32 20) -> ()  [unwired: 1 out]
    n30 = local write "Red LED"(w71) -> ()
  }
  n31 = while {
    tunnel: w59 -> [w132]
    tunnel: w60 -> [w131]
    tunnel: [w130] -> w66
    tunnel: [w129] -> w65
    tunnel: w64 -> [w128]
    tunnel: [w127] -> w62
    tunnel: w63 -> [w126]
    tunnel: [w125] -> w61
    stop <- w123 stop-if-true
    # "Generate USER Event Loop"
    n32 = local read "Rising Edge"() -> (w120:bool)
    n33 = Or(x="OK Button", y=w120) -> (x .or. y?=w119:bool)
    n34 = local read "TASK ENABLE"() -> (w118:bool)
    n35 = And(x=w119, y=w118) -> (x .and. y?=w117:bool)
    n36 = case shown="True" w117 {
      selector: w117 -> [_ w143]
      tunnel: w132 -> [w142 w147]
      tunnel: [w142 w146] -> w129
      tunnel: w128 -> [w141 w145]
      tunnel: [w141 w144] -> w127
      frame False {
      }
      frame True {
        n37 = Generate User Event(user event=w147, event data cluster=w143, error in=w145) -> (user event out=w146:refnum<user-event>, error out=w144:errorcluster)  [unwired: 1 in]
      }
    }
    n38 = case shown="False" "STOP" {
      selector: "STOP" -> [_ w136]
      tunnel: w131 -> [w135 w140]
      tunnel: [w135 w139] -> w130
      tunnel: w126 -> [w134 w138]
      tunnel: [w134 w137] -> w125
      tunnel: [FALSE w136] -> w123
      frame False {
      }
      frame True {
        n39 = Generate User Event(user event=w140, event data cluster=w136, error in=w138) -> (user event out=w139:refnum<user-event>, error out=w137:errorcluster)  [unwired: 1 in]
      }
    }
    n40 = Wait (ms)(milliseconds to wait=u32 10) -> ()  [unwired: 1 out]
    n41 = call "FGV Bool.vi"("Init/Read/Write State"=States_for_Action_Engine."Write", "Input Node"=w123) -> ()  [unwired: 1 in, 2 out]
  }
  n42 = while {
    tunnel: w58 -> [w154]
    tunnel: [w153] -> w57
    tunnel: w45 -> [w151]
    tunnel: [w150] -> w56
    tunnel: w51 -> [w149]
    tunnel: [w148] -> w48
    stop <- w152 stop-if-true
    # "EVENT Handling Loop"
    n43 = event shown="[1] <Start Task>: User Event" {
      selector: w154 -> [_ _ _]
      dyn-events: [_ _ _] -> w153
      timeout: _ -> [_ _ _]
      tunnel: [FALSE FALSE w188] -> w152
      tunnel: w151 -> [w159 w168 w186]
      tunnel: [w158 w167 w187] -> w150
      tunnel: w149 -> [w157 w166 w185]
      tunnel: [w156 w165 w184] -> w148
      event Timeout {
        n44 = event-data() -> ()  [unwired: 1 in, 3 out]
        n45 = Enqueue Element(queue=w159, element=Intruction_Type_Definitions."Start Task 1" ("Enum"), error in (no error)=w157) -> (queue out=w158:refnum<queue>, error out=w156:errorcluster)  [unwired: 1 in, 1 out]
      }
      event User Event {
        n46 = event-data() -> ()  [unwired: 1 in, 5 out]
        n47 = call "Arduino Interfacing VI.vi"("AE Mode"=Arduino_Interfacing."Read From Arduino") -> ("Arduino Data"=w162:T8)  [unwired: 3 in, 1 out]
        n48 = Unbundle By Name(w162) -> ("Rotary Switch"=w161:u8)
        n49 = case shown="0, Default" w161 {
          tunnel: [Intruction_Type_Definitions."Start Task 1" ("Enum") Intruction_Type_Definitions."Start Task 2" ("Enum") Intruction_Type_Definitions."Start Task 3" ("Enum") Intruction_Type_Definitions."Start Task 4" ("Enum") Intruction_Type_Definitions."Start Task 5" ("Enum") Intruction_Type_Definitions."Start Task 6" ("Enum") Intruction_Type_Definitions."Start Task 7" ("Enum") Intruction_Type_Definitions."Start Task 8 - BALL" ("Enum") Intruction_Type_Definitions."Start Task 8 - Gel" ("Enum") Intruction_Type_Definitions."Start Task 8 - Pipe" ("Enum") Intruction_Type_Definitions."Start Task 8 - Soap" ("Enum") Intruction_Type_Definitions."Start Task 9" ("Enum") Intruction_Type_Definitions."None" ("Enum")] -> w164
          frame 0, Default {
          }
          frame 1 {
          }
          frame 2 {
          }
          frame 3 {
          }
          frame 4 {
          }
          frame 5 {
          }
          frame 6 {
          }
          frame 7 {
          }
          frame 8 {
          }
          frame 9 {
          }
          frame 10 {
          }
          frame 11 {
          }
          frame 12 {
          }
        }
        "Selected Task" <- w164
        n50 = Enqueue Element(queue=w168, element=w164, error in (no error)=w166) -> (queue out=w167:refnum<queue>, error out=w165:errorcluster)  [unwired: 1 in, 1 out]
      }
      event User Event {
        n51 = event-data() -> ("Stop Queue"=w188:bool)  [unwired: 1 in, 4 out]
        n52 = Enqueue Element At Opposite End(queue=w186, element=Intruction_Type_Definitions."Exit" ("Enum"), error in (no error)=w185) -> (queue out=w187:refnum<queue>, error out=w184:errorcluster)  [unwired: 1 in, 1 out]
      }
    }
  }
  n53 = while {
    tunnel: w46 -> [w198]
    tunnel: w45 -> [w195]
    stop <- w192 stop-if-true
    # "Status Loop for Action Queues"
    n54 = Get Queue Status(queue=w198, return elements? (F)=TRUE) -> (error out=w194:errorcluster, # elements in queue=→"Action Queue Items":i32, elements=→"Action Queues items":string[])  [unwired: 1 in, 5 out]
    n55 = Get Queue Status(queue=w195, return elements? (F)=TRUE) -> (# pending remove=→"State Logic Queue Items":i32, error out=w193:errorcluster, elements=→"elements":T1[])  [unwired: 1 in, 5 out]
    n56 = Merge Errors(w194, w193) -> (w192:errorcluster)
    n57 = Wait (ms)(milliseconds to wait=u32 500) -> ()  [unwired: 1 out]
  }
  n58 = while {
    tunnel: w45 -> [w242]
    tunnel: w46 -> [w254]
    tunnel: w49 -> [w252]
    tunnel: [w251] -> _
    tunnel: [w250] -> w39
    shift-right: [w243] -> _
    shift-left: T19 {"PING_A"=0, "PING_B"=0, "PING_C"=0, "PING_D"=0} -> [w245]
    shift-right: [w236] -> _
    shift-left: State_Type_Definitions."Startup" ("Enum") -> [w239]
    shift-right: [w232] -> _
    shift-left: T20 {"xDistance"=0.0, "yDistance"=0.0, "wDistance"=0.0} -> [w234]
    shift-right: [w229] -> _
    shift-left: _ -> [w228]
    shift-right: [w225] -> _
    shift-left: T2 {"Recognized Object"=FALSE, "Object X coordinate"=0.0, "Object Y coordinate"=0.0} -> [w227]
    shift-right: [w222] -> _
    shift-left: T17 {"y Stepper Position"=0, "z Stepper Position"=0} -> [w224]
    shift-right: [w219] -> _
    shift-left: T16 {"Yaw"=0.0, "Compass"=0.0} -> [w221]
    shift-right: [w216] -> _
    shift-left: T15 {"Time up flag"=FALSE, "SET TIME TO CHECK"=0.0} -> [w218]
    shift-right: [w214] -> _
    shift-left: T14 {"yStepper desired"=0} -> [w215]
    shift-right: [w210] -> _
    shift-left: T13 {"Left IR Sensor"=0.0, "Arm IR Sensor"=0.0, "Bottom IR Sensor"=0.0} -> [w212]
    shift-right: [w208] -> _
    shift-left: T12 {"ySpeed"=0.0, "xSpeed"=0.0, "wSpeed"=0.0} -> [w209]
    shift-right: [w205] -> _
    shift-left: T11 {"Line Detected?"=FALSE, "S1"=0.0, "S2"=0.0, "S3"=0.0, "S4"=0.0} -> [w207]
    shift-right: [w203] -> _
    shift-left: _ -> [w202]
    stop <- w241 stop-if-true
    # ">>> Line Sensor Cluster>>>"
    # ">>> IR Sensors >>>"
    # ">>> Time cluster >>>"
    # ">>> Object detection >>>"
    # ">>> Yaw >>>"
    # ">>> Ultrasonic Sensors Detect >>>"
    # ">>> Encoders >>>"
    # ">>> Stepper position >>>"
    # ">>State Logic  >>"
    # ">> Item Selection Bias >>"
    # ">> Item Selection Bias >>"
    # ">> Item Selection Bias >>"
    # ">>State Logic  >>"
    # ">>> Motor control cluster >>>"
    # ">>> yStepper command>>>"
    # ">>True Stop Next State >>"
    # ">>Error  >>"
    # ">>Timeout>>"
    # ">>Action states Queue Reference >>"
    # ">>State Logic Queue Reference >>"
    # "TOP LEVEL BASELINE (MAIN PROCESSING LOOP)"
    n59 = Wait (ms)(milliseconds to wait=u32 20) -> ()  [unwired: 1 out]
    n60 = Dequeue Element(queue=w254, timeout in ms (-1)=0, error in (no error)=w252) -> (queue out=w246:refnum<queue>, element=w253:string, error out=w247:errorcluster)  [unwired: 1 out]
    "Action State" <- w253
    n61 = case shown="\"FORWARD\"" w253 {
      tunnel: [_ _ _ _ _ _ _ _ _ _ _ _ _ _ _ _ _ _ _ _ 0 w2509 _ _ _ _ _ _ _ _ _ _ _ _ _ _ _ _ _ _ _ _ _ _ _ _ _ _ _ _ _] -> w249
      tunnel: w246 -> [_ _ _ _ _ _ _ _ _ _ _ _ _ _ _ _ _ _ _ _ _ _ _ _ _ _ _ _ _ _ _ _ _ _ _ _ _ _ _ _ _ _ _ _ _ _ _ _ _ _ _]
      tunnel: w245 -> [w2205 w2216 w2230 w2243 w2262 w2275 w2288 w2302 w2317 w2331 w2344 w2353 w2370 w2386 w2400 w2412 w2435 w2444 w2473 w2485 w2498 w2510 w2521 w2533 w2565 w2578 w2588 w2599 w2611 w2625 w2640 w2651 w2662 w2681 w2691 w2706 w2715 w2727 w2739 w2751 w2760 w2777 w2786 w2804 w2812 w2826 w2840 w2854 w2868 w2882 w2895]
      tunnel: [w2205 w2216 w2230 w2243 w2262 w2275 w2288 w2302 w2317 w2331 w2344 w2353 w2370 w2387 w2400 w2412 w2435 w2444 w2474 w2485 w2498 w2510 w2521 w2533 w2564 w2578 w2588 w2599 w2611 w2625 w2640 w2651 w2662 w2681 w2691 w2706 w2715 w2727 w2739 w2751 w2760 w2777 w2786 w2804 w2812 w2826 w2840 w2854 w2868 w2882 w2895] -> w244
      tunnel: [TRUE TRUE _ _ _ _ _ _ _ _ _ _ _ _ _ _ _ _ _ _ _ _ _ _ _ _ _ _ _ _ _ _ _ _ _ _ _ _ _ _ _ _ _ _ _ _ _ _ _ _ _] -> w241
      tunnel: w239 -> [w2203 w2214 w2229 w2242 w2261 w2274 w2287 w2301 w2316 w2330 w2343 w2352 w2369 w2385 w2399 w2410 w2428 w2443 w2472 w2484 w2495 w2507 w2520 w2532 w2563 w2577 w2587 w2598 w2603 w2624 w2639 w2650 w2661 w2680 w2690 w2700 w2714 w2726 w2738 w2750 w2759 w2768 w2785 w2803 w2811 w2825 w2839 w2853 w2867 w2881 w2894]
      tunnel: [_ _ _ _ _ _ _ _ _ _ _ _ _ _ _ _ _ _ _ _ _ TRUE _ _ _ _ _ _ _ _ _ _ _ _ _ _ _ _ _ _ _ _ _ _ _ _ _ _ _ _ _] -> w238
      tunnel: [w2203 w2214 w2229 w2242 w2261 w2274 w2287 w2301 w2316 w2330 w2343 w2352 w2369 w2385 w2399 w2410 w2428 w2443 w2472 w2484 w2495 w2507 w2520 w2532 w2563 w2577 w2587 w2598 w2603 w2624 w2639 w2650 w2661 w2680 w2690 w2700 w2714 w2726 w2738 w2750 w2759 w2768 w2785 w2803 w2811 w2825 w2839 w2853 w2867 w2881 w2894] -> w237
      tunnel: w234 -> [w2202 w2213 w2228 w2245 w2260 w2273 w2286 w2300 w2315 w2329 w2342 w2354 w2368 w2384 w2401 w2414 w2430 w2445 w2471 w2486 w2494 w2506 w2522 w2534 w2553 w2576 w2590 w2600 w2608 w2626 w2641 w2652 w2663 w2682 w2693 w2704 w2717 w2729 w2741 w2753 w2762 w2772 w2788 w2806 w2814 w2828 w2842 w2856 w2870 w2884 w2897]
      tunnel: [w2202 w2213 w2228 w2245 w2260 w2273 w2286 w2300 w2315 w2329 w2342 w2354 w2367 w2384 w2401 w2414 w2430 w2445 w2470 w2486 w2494 w2506 w2522 w2534 w2552 w2576 w2590 w2600 w2608 w2626 w2641 w2652 w2663 w2682 w2693 w2704 w2717 w2729 w2741 w2753 w2762 w2772 w2788 w2806 w2814 w2828 w2842 w2856 w2870 w2884 w2897] -> w233
      tunnel: w227 -> [w2201 w2212 w2227 w2244 w2259 w2272 w2285 w2299 w2314 w2328 w2340 w2351 w2366 w2383 w2394 w2413 w2429 w2442 w2462 w2483 w2493 w2505 w2519 w2531 w2558 w2574 w2589 w2597 w2609 w2623 w2638 w2646 w2660 w2676 w2692 w2705 w2716 w2728 w2740 w2752 w2761 w2771 w2787 w2805 w2813 w2827 w2841 w2855 w2869 w2883 w2896]
      tunnel: [w2201 w2212 w2227 w2244 w2259 w2272 w2285 w2299 w2314 w2328 w2340 w2351 w2366 w2383 w2394 w2413 w2429 w2442 w2461 w2483 w2493 w2505 w2519 w2531 w2557 w2574 w2589 w2597 w2609 w2623 w2638 w2646 w2660 w2675 w2692 w2705 w2716 w2728 w2740 w2752 w2761 w2771 w2787 w2805 w2813 w2827 w2841 w2855 w2869 w2883 w2896] -> w226
      tunnel: w224 -> [w2200 w2211 w2226 w2246 w2258 w2271 w2284 w2298 w2313 w2327 w2339 w2350 w2365 w2382 w2402 w2415 w2431 w2441 w2467 w2482 w2492 w2504 w2518 w2530 w2548 w2573 w2586 w2596 w2607 w2622 w2637 w2649 w2659 w2683 w2694 w2703 w2713 w2725 w2737 w2749 w2763 w2773 w2789 w2802 w2815 w2829 w2843 w2857 w2871 w2885 w2898]
      tunnel: [w2200 w2211 w2226 w2246 w2258 w2271 w2284 w2298 w2313 w2327 w2339 w2350 w2365 w2382 w2402 w2415 w2431 w2441 w2466 w2482 w2492 w2504 w2518 w2530 w2547 w2573 w2586 w2596 w2607 w2622 w2637 w2649 w2659 w2683 w2694 w2703 w2713 w2725 w2737 w2749 w2763 w2773 w2789 w2801 w2815 w2829 w2843 w2857 w2871 w2885 w2898] -> w223
      tunnel: w221 -> [w2199 w2210 w2224 w2247 w2256 w2269 w2283 w2296 w2311 w2325 w2338 w2349 w2364 w2375 w2397 w2416 w2432 w2440 w2457 w2481 w2491 w2503 w2517 w2529 w2544 w2572 w2583 w2595 w2606 w2621 w2636 w2648 w2658 w2684 w2695 w2702 w2712 w2722 w2734 w2746 w2764 w2774 w2790 w2796 w2816 w2830 w2844 w2858 w2872 w2886 w2899]
      tunnel: [w2199 w2210 w2224 w2247 w2256 w2269 w2283 w2296 w2311 w2325 w2338 w2349 w2364 w2375 w2396 w2416 w2432 w2440 w2456 w2481 w2491 w2503 w2517 w2529 w2543 w2572 w2583 w2595 w2606 w2621 w2636 w2648 w2658 w2684 w2695 w2702 w2712 w2722 w2734 w2746 w2764 w2774 w2790 w2796 w2816 w2830 w2844 w2858 w2872 w2886 w2899] -> w220
      tunnel: w218 -> [w2197 w2209 w2225 w2248 w2257 w2270 w2282 w2297 w2312 w2326 w2337 w2348 w2363 w2374 w2393 w2417 w2433 w2439 w2453 w2478 w2490 w2502 w2516 w2528 w2541 w2570 w2582 w2594 w2605 w2620 w2635 w2647 w2657 w2685 w2696 w2701 w2711 w2721 w2733 w2745 w2765 w2775 w2791 w2795 w2810 w2824 w2838 w2852 w2866 w2880 w2893]
      tunnel: [w2197 w2209 w2225 w2248 w2257 w2270 w2282 w2297 w2312 w2326 w2337 w2348 w2363 w2374 w2393 w2417 w2433 w2439 w2453 w2478 w2490 w2502 w2516 w2528 w2540 w2570 w2582 w2594 w2605 w2620 w2635 w2647 w2657 w2685 w2696 w2701 w2711 w2721 w2733 w2745 w2765 w2775 w2791 w2795 w2810 w2822 w2836 w2850 w2864 w2878 w2892] -> w217
      tunnel: w215 -> [_ _ _ _ _ _ _ _ _ _ _ _ _ _ _ _ _ _ _ _ _ _ _ _ _ _ _ _ _ _ _ _ _ _ _ _ _ _ _ _ _ _ w2782 _ _ _ _ _ _ _ _]
      tunnel: [w2196 w2208 w2219 w2238 w2251 w2265 w2278 w2291 w2307 w2320 w2334 w2347 w2357 w2373 w2390 w2408 w2434 w2438 w2450 w2477 w2489 w2501 w2515 w2525 w2537 w2569 w2581 w2593 w2610 w2614 w2629 w2644 w2655 w2669 w2688 w2707 w2710 w2720 w2732 w2744 w2756 w2776 w2780 w2794 w2809 w2819 w2833 w2847 w2861 w2875 w2889] -> w211
      tunnel: w212 -> [w2196 w2208 w2219 w2238 w2251 w2265 w2278 w2291 w2307 w2320 w2334 w2347 w2357 w2373 w2390 w2409 w2434 w2438 w2450 w2477 w2489 w2501 w2515 w2525 w2537 w2569 w2581 w2593 w2610 w2614 w2629 w2644 w2655 w2669 w2688 w2707 w2710 w2720 w2732 w2744 w2756 w2776 w2780 w2794 w2809 w2819 w2833 w2847 w2861 w2875 w2889]
      tunnel: w209 -> [_ _ _ _ _ _ _ _ w2306 _ _ _ _ _ _ _ _ _ _ _ _ _ _ _ _ _ _ _ _ _ _ _ _ _ _ _ _ _ _ _ _ _ _ _ _ _ _ _ _ _ _]
      tunnel: w207 -> [w2195 w2207 w2218 w2232 w2250 w2264 w2277 w2290 w2304 w2319 w2333 w2346 w2356 w2372 w2389 w2404 w2427 w2437 w2448 w2476 w2488 w2500 w2514 w2524 w2536 w2568 w2580 w2592 w2602 w2613 w2628 w2643 w2654 w2666 w2687 w2698 w2709 w2719 w2731 w2743 w2755 w2767 w2779 w2793 w2808 w2818 w2832 w2846 w2860 w2874 w2888]
      tunnel: [w2195 w2207 w2218 w2232 w2250 w2264 w2277 w2290 w2304 w2319 w2333 w2346 w2356 w2372 w2389 w2404 w2426 w2437 w2448 w2476 w2488 w2500 w2514 w2524 w2536 w2568 w2580 w2592 w2602 w2613 w2628 w2643 w2654 w2666 w2687 w2698 w2709 w2719 w2731 w2743 w2755 w2767 w2779 w2793 w2808 w2818 w2832 w2846 w2860 w2874 w2888] -> w206
      tunnel: [_ _ _ _ _ _ _ _ _ _ _ _ _ _ _ _ _ _ _ _ _ _ _ _ _ _ _ _ _ _ _ _ _ w2665 _ _ _ _ _ _ _ _ _ _ _ _ _ _ _ _ _] -> w204
      tunnel: w202 -> [w2194 w2206 w2217 w2231 w2249 w2263 w2276 w2289 w2303 w2318 w2332 w2345 w2355 w2371 w2388 w2403 w2418 w2436 w2446 w2475 w2487 w2499 w2513 w2523 w2535 w2567 w2579 w2591 w2601 w2612 w2627 w2642 w2653 w2664 w2686 w2697 w2708 w2718 w2730 w2742 w2754 w2766 w2778 w2792 w2807 w2817 w2831 w2845 w2859 w2873 w2887]
      tunnel: [w2194 w2206 w2217 w2231 w2249 w2263 w2276 w2289 w2303 w2318 w2332 w2345 w2355 w2371 w2388 w2403 w2418 w2436 w2446 w2475 w2487 w2499 w2513 w2523 w2535 w2567 w2579 w2591 w2601 w2612 w2627 w2642 w2653 w2664 w2686 w2697 w2708 w2718 w2730 w2742 w2754 w2766 w2778 w2792 w2807 w2817 w2831 w2845 w2859 w2873 w2887] -> w201
      frame "Exit" {
        # ">>State Logic  >>"
        # ">>> Time cluster >>>"
        # ">>> Yaw >>>"
        # ">>> Stepper position >>>"
        # ">>> Encoders >>>"
        # ">>> Object detection >>>"
        # ">>> Ultrasonic Sensors Detect >>>"
        n62 = call "Imaq Dispose"("All Images? (No)"=TRUE) -> ()  [unwired: 5 in, 1 out]
      }
      frame "----Movement States----" {
        # ">>State Logic  >>"
        # ">>> Time cluster >>>"
        # ">>> Yaw >>>"
        # ">>> Stepper position >>>"
        # ">>> Encoders >>>"
        # ">>> Object detection >>>"
        # ">>> Ultrasonic Sensors Detect >>>"
      }
      frame "FORWARD" {
        # ">>State Logic  >>"
        # ">>> Time cluster >>>"
        # ">>> Yaw >>>"
        # ">>> Stepper position >>>"
        # ">>> Encoders >>>"
        # ">>> Object detection >>>"
        # ">>> Ultrasonic Sensors Detect >>>"
        n63 = Unbundle By Name(w2224) -> ("Yaw"=w2220:dbl)
        n64 = call "MOTOR CONTROL WITH PID AE.vi"("Yaw"=w2220, "Speed"=30.0, "Direction"=MOTOR_CONTROL_WITH_PID_AE_DIRECTION_TYPE_DEF."y-axis movement", "AE Mode"=MOTOR_CONTROL_WITH_PID_AE_DATA_MODE_TYPE_DEF."Write to AE") -> ()  [unwired: 1 out]
      }
      frame "FORWARD - IR ASSIST" {
        # ">>State Logic  >>"
        # ">>> Time cluster >>>"
        # ">>> Yaw >>>"
        # ">>> Stepper position >>>"
        # ">>> Encoders >>>"
        # ">>> Object detection >>>"
        # ">>> Ultrasonic Sensors Detect >>>"
        n65 = Unbundle By Name(w2238) -> ("Left IR Sensor"=w2237:dbl)
        n66 = Subtract(x=w2237, y=20.0) -> (x-y=w2235:dbl)
        n67 = Multiply(x=w2235, y=0.25) -> (x*y=w2233:dbl)
        n68 = call "MOTOR CONTROL WITH PID AE.vi"("Yaw"=w2233, "Speed"=30.0, "Direction"=MOTOR_CONTROL_WITH_PID_AE_DIRECTION_TYPE_DEF."y-axis movement", "AE Mode"=MOTOR_CONTROL_WITH_PID_AE_DATA_MODE_TYPE_DEF."Write to AE") -> ()  [unwired: 1 out]
      }
      frame "LEFT" {
        # ">>State Logic  >>"
        # ">>> Time cluster >>>"
        # ">>> Yaw >>>"
        # ">>> Stepper position >>>"
        # ">>> Encoders >>>"
        # ">>> Object detection >>>"
        # ">>> Ultrasonic Sensors Detect >>>"
        n69 = Unbundle By Name(w2256) -> ("Yaw"=w2253:dbl)
        n70 = call "MOTOR CONTROL WITH PID AE.vi"("Yaw"=w2253, "Speed"=-30.0, "Direction"=MOTOR_CONTROL_WITH_PID_AE_DIRECTION_TYPE_DEF."x-axis movement", "AE Mode"=MOTOR_CONTROL_WITH_PID_AE_DATA_MODE_TYPE_DEF."Write to AE") -> ()  [unwired: 1 out]
      }
      frame "R-ACW" {
        # ">>> IR Sensors >>>"
        # ">>> Time cluster >>>"
        # ">>> Yaw >>>"
        # ">>> Stepper position >>>"
        # ">>> Encoders >>>"
        # ">>> Object detection >>>"
        # ">>> Ultrasonic Sensors Detect >>>"
        n71 = call "MOTOR CONTROL WITH PID AE.vi"("Speed"=-10.0, "Direction"=MOTOR_CONTROL_WITH_PID_AE_DIRECTION_TYPE_DEF."rotation", "AE Mode"=MOTOR_CONTROL_WITH_PID_AE_DATA_MODE_TYPE_DEF."Write to AE") -> ()  [unwired: 1 in, 1 out]
      }
      frame "R-CW" {
        (unwired) -0.2 ("Speed")
        # ">>> Time cluster >>>"
        # ">>> Yaw >>>"
        # ">>> Stepper position >>>"
        # ">>> Encoders >>>"
        # ">>> Object detection >>>"
        # ">>> Ultrasonic Sensors Detect >>>"
        n72 = call "MOTOR CONTROL WITH PID AE.vi"("Speed"=10.0, "Direction"=MOTOR_CONTROL_WITH_PID_AE_DIRECTION_TYPE_DEF."rotation", "AE Mode"=MOTOR_CONTROL_WITH_PID_AE_DATA_MODE_TYPE_DEF."Write to AE") -> ()  [unwired: 1 in, 1 out]
      }
      frame "RIGHT" {
        # ">>> Time cluster >>>"
        # ">>> Yaw >>>"
        # ">>> Stepper position >>>"
        # ">>> Encoders >>>"
        # ">>> Object detection >>>"
        # ">>> Ultrasonic Sensors Detect >>>"
        n73 = Unbundle By Name(w2296) -> ("Yaw"=w2292:dbl)
        n74 = call "MOTOR CONTROL WITH PID AE.vi"("Yaw"=w2292, "Speed"=50.0, "Direction"=MOTOR_CONTROL_WITH_PID_AE_DIRECTION_TYPE_DEF."x-axis movement", "AE Mode"=MOTOR_CONTROL_WITH_PID_AE_DATA_MODE_TYPE_DEF."Write to AE") -> ()  [unwired: 1 out]
      }
      frame "X AXIS - SLOW" {
        # ">>> IR Sensors >>>"
        # ">>> Time cluster >>>"
        # ">>> Yaw >>>"
        # ">>> Stepper position >>>"
        # ">>> Encoders >>>"
        # ">>> Object detection >>>"
        # ">>> Ultrasonic Sensors Detect >>>"
        n75 = Unbundle By Name(w2306) -> ("xSpeed"=w2305:dbl)
        n76 = Unbundle By Name(w2311) -> ("Yaw"=w2308:dbl)
        n77 = call "MOTOR CONTROL WITH PID AE.vi"("Yaw"=w2308, "Speed"=w2305, "Direction"=MOTOR_CONTROL_WITH_PID_AE_DIRECTION_TYPE_DEF."x-axis movement", "AE Mode"=MOTOR_CONTROL_WITH_PID_AE_DATA_MODE_TYPE_DEF."Write to AE") -> ()  [unwired: 1 out]
      }
      frame "REVERSE" {
        # ">>> Time cluster >>>"
        # ">>> Yaw >>>"
        # ">>> Stepper position >>>"
        # ">>> Encoders >>>"
        # ">>> Object detection >>>"
        # ">>> Ultrasonic Sensors Detect >>>"
        n78 = Unbundle By Name(w2325) -> ("Yaw"=w2321:dbl)
        n79 = call "MOTOR CONTROL WITH PID AE.vi"("Yaw"=w2321, "Speed"=-50.0, "Direction"=MOTOR_CONTROL_WITH_PID_AE_DIRECTION_TYPE_DEF."y-axis movement", "AE Mode"=MOTOR_CONTROL_WITH_PID_AE_DATA_MODE_TYPE_DEF."Write to AE") -> ()  [unwired: 1 out]
      }
      frame "STOP" {
        n80 = Wait (ms)(milliseconds to wait=u32 100) -> ()  [unwired: 1 out]
        n81 = call "MOTOR CONTROL WITH PID AE.vi"("Direction"=MOTOR_CONTROL_WITH_PID_AE_DIRECTION_TYPE_DEF."stop", "AE Mode"=MOTOR_CONTROL_WITH_PID_AE_DATA_MODE_TYPE_DEF."Write to AE") -> ()  [unwired: 2 in, 1 out]
      }
      frame "----SENSOR READING---- " {
      }
      frame "READ ENCODERS" {
        # ">>> Time cluster >>>"
        # ">>> Yaw >>>"
        # ">>> Stepper position >>>"
        # ">>> Object detection >>>"
        # ">>> Current encoder distance >>>"
        # ">>> Ultrasonic Sensors Detect >>>"
        n82 = call "MOTOR CONTROL WITH PID AE.vi"("AE Mode"=MOTOR_CONTROL_WITH_PID_AE_DATA_MODE_TYPE_DEF."Read from AE") -> ("Speed & distance"=w2361:T6)  [unwired: 3 in]
        n83 = Unbundle By Name(w2361) -> ("xDistance"=w2360:dbl, "yDistance"=w2359:dbl, "wDistance"=w2358:dbl)
        n84 = Bundle By Name(cluster=w2368, "xDistance"=w2360, "yDistance"=w2359, "wDistance"=w2358) -> (w2367:T20)
      }
      frame "READ ULTRASONIC" {
        (unwired) navX_type_def."Read Values" ("Mode")
        (unwired) MOTOR_CONTROL_NO_PID_Type_Def."Latch" ("Direction")
        # ">>State Logic  >>"
        # ">>> Time cluster >>>"
        # ">>> Ultrasonic Sensors Detect >>>"
        # ">>> Object detection >>>"
        # ">>> Encoders >>>"
        # ">>> Stepper position >>>"
        # ">>> Yaw >>>"
        n85 = call "Arduino Interfacing VI.vi"("AE Mode"=Arduino_Interfacing."Read From Arduino") -> ("Arduino Data"=w2380:T8)  [unwired: 3 in, 1 out]
        n86 = Unbundle By Name(w2380) -> ("PING A"=w2379:u8, "PING B"=w2378:u8, "PING C"=w2377:u8, "PING D"=w2376:u8)
        n87 = Bundle By Name(cluster=w2386, "PING_A"=w2379, "PING_B"=w2378, "PING_C"=w2377, "PING_D"=w2376) -> (w2387:T19)
      }
      frame "READ NAVX" {
        # ">>> Time cluster >>>"
        # ">>> Yaw >>>"
        # ">>> Ultrasonic Sensors Detect >>>"
        # ">>> Object detection >>>"
        # ">>> Encoders >>>"
        # ">>> Stepper position >>>"
        n88 = call "navX reading VI.vi"("Mode"=navX_type_def."Read Values") -> ("NavX Readings"=w2392:T7)  [unwired: 2 in, 3 out]
        n89 = Unbundle By Name(w2392) -> ("Heading"=w2391:dbl)
        n90 = Unbundle By Name(w2392) -> ("Yaw"=w2395:dbl)
        n91 = Bundle By Name(cluster=w2397, "Yaw"=w2395, "Compass"=w2391) -> (w2396:T16)
      }
      frame "READ IR" {
        w2406 = T37 [enum."B/AI1"] items=["Not Connected", "AudioIn/Left", "AudioIn/Right", "C/AI0", "C/AI1", "A/AI0", "A/AI1", "A/AI2", "A/AI3", "A/AI4", "A/AI5", "A/AI6", "A/AI7", "B/AI0", "B/AI1", "B/AI2", "B/AI3", "B/AI4", "B/AI5", "B/AI6", "B/AI7", "AI/AI0", "AI/AI1", "AI/AI2", "AI/AI3", "A/AI0 (DIFF)", "A/AI1 (DIFF)", "A/AI2 (DIFF)", "A/AI3 (DIFF)", "B/AI0 (DIFF)", "B/AI1 (DIFF)", "B/AI2 (DIFF)", "B/AI3 (DIFF)"] ("AI Channel")
        w2411 = T37 [enum."B/AI0"] items=["Not Connected", "AudioIn/Left", "AudioIn/Right", "C/AI0", "C/AI1", "A/AI0", "A/AI1", "A/AI2", "A/AI3", "A/AI4", "A/AI5", "A/AI6", "A/AI7", "B/AI0", "B/AI1", "B/AI2", "B/AI3", "B/AI4", "B/AI5", "B/AI6", "B/AI7", "AI/AI0", "AI/AI1", "AI/AI2", "AI/AI3", "A/AI0 (DIFF)", "A/AI1 (DIFF)", "A/AI2 (DIFF)", "A/AI3 (DIFF)", "B/AI0 (DIFF)", "B/AI1 (DIFF)", "B/AI2 (DIFF)", "B/AI3 (DIFF)"] ("AI Channel")
        # ">>State Logic  >>"
        # ">>> Time cluster >>>"
        # ">>> Ultrasonic Sensors Detect >>>"
        # ">>> Object detection >>>"
        # ">>> Encoders >>>"
        # ">>> Stepper position >>>"
        # ">>> Yaw >>>"
        n92 = call <vilib>:"Sharp IR.vi"("AI Channel"=w2411) -> ("Sharp IR Distance"=w2407:dbl)  [unwired: 8 in, 2 out]
        n93 = call <vilib>:"Sharp IR.vi"("AI Channel"=w2406) -> ("Sharp IR Distance"=w2405:dbl)  [unwired: 8 in, 2 out]
        n94 = Bundle By Name(cluster=w2409, "Left IR Sensor"=w2407, "Arm IR Sensor"=w2405) -> (w2408:T13)
      }
      frame "READ LINE SENSOR" {
        # ">>> IR Sensors >>>"
        # ">>> Line Sensor Cluster>>>"
        # ">>State Logic  >>"
        # ">>> Time cluster >>>"
        # ">>> Object detection >>>"
        # ">>> Yaw >>>"
        # ">>> Ultrasonic Sensors Detect >>>"
        # ">>> Encoders >>>"
        # ">>> Stepper position >>>"
        n95 = call "Line Sensor AE.vi"("AE State"=Line_Sensor_AE_Type_Def."READ FROM LINE SENSORS") -> ("Line Detected?"=w2424:bool, "Line Sensor Raw Values"=w2423:T39)
        n96 = Unbundle By Name(w2423) -> ("S1"=w2422:dbl, "S2"=w2421:dbl, "S3"=w2420:dbl, "S4"=w2419:dbl)
        n97 = Bundle By Name(cluster=w2427, "Line Detected?"=w2424, "S1"=w2422, "S2"=w2421, "S3"=w2420, "S4"=w2419) -> (w2426:T11)
      }
      frame "----SYSTEM MODES----" {
        (unwired) I2C_MASTER_Type_Def."Last State" ("Arduino Mode")
        # ">>> Object detection >>>"
        # ">>> Yaw >>>"
        # ">>> Ultrasonic Sensors Detect >>>"
        # ">>> Encoders >>>"
        # ">>> Stepper position >>>"
      }
      frame "INIT" {
        w2468 = u8 0
        w2469 = 0.0
        # ">>> IR Sensors >>>"
        # ">>> IR Sensors >>>"
        # ">>> Line Sensor Cluster>>>"
        # ">>> Time cluster >>>"
        # ">>> Object detection >>>"
        # ">>> Yaw >>>"
        # ">>> Ultrasonic Sensors Detect >>>"
        # ">>> Encoders >>>"
        # ">>> Stepper position >>>"
        # ">>State Logic  >>"
        n98 = call "Arduino Interfacing VI.vi"("AE Mode"=Arduino_Interfacing."Initialize") -> ()  [unwired: 3 in, 2 out]
        n99 = call "FGV Bool.vi"("Init/Read/Write State"=States_for_Action_Engine."Initialize") -> ()  [unwired: 2 in, 2 out]
        n100 = call "Elasped Timer.vi"("Action"=Elapsed_timer_control."Initialize") -> ()  [unwired: 7 in, 4 out]
        n101 = call "MOTOR CONTROL WITH PID AE.vi"("AE Mode"=MOTOR_CONTROL_WITH_PID_AE_DATA_MODE_TYPE_DEF."Init AE") -> ()  [unwired: 3 in, 1 out]
        n102 = call "IMAQ Reference AE.vi"("IMAQ AE States"=IMAQ_Reference_AE."Initialize AE") -> ()  [unwired: 1 in, 2 out]
        n103 = call "Line Sensor AE.vi"("AE State"=Line_Sensor_AE_Type_Def."INIT AE") -> ()  [unwired: 2 out]
        n104 = Bundle By Name(cluster=w2462, "Recognized Object"=FALSE, "Object X coordinate"=0.0, "Object Y coordinate"=0.0) -> (w2461:T2)
        n105 = Bundle By Name(cluster=w2467, "y Stepper Position"=u8 0, "z Stepper Position"=u8 0) -> (w2466:T17)
        n106 = Bundle By Name(cluster=w2471, "xDistance"=w2469, "yDistance"=w2469, "wDistance"=w2469) -> (w2470:T20)
        n107 = Bundle By Name(cluster=w2473, "PING_A"=w2468, "PING_B"=w2468, "PING_C"=w2468, "PING_D"=w2468) -> (w2474:T19)
        n108 = Bundle By Name(cluster=w2457, "Yaw"=0.0) -> (w2456:T16)
      }
      frame "ARDUINO - ULTRASONIC" {
        # ">>> Time cluster >>>"
        # ">>> Line Sensor Cluster>>>"
        # ">>> Object detection >>>"
        # ">>> Yaw >>>"
        # ">>> Ultrasonic Sensors Detect >>>"
        # ">>> Encoders >>>"
        # ">>> Stepper position >>>"
        # ">>State Logic  >>"
        n109 = call "Arduino Interfacing VI.vi"("Data to Write"=I2C_MASTER_WRITE_NEW_Type_Def."Ultrasonic sensors", "AE Mode"=Arduino_Interfacing."Write to Arduino") -> ()  [unwired: 2 in, 2 out]
      }
      frame "NAVX CALIBRATE" {
        # ">>> Object detection >>>"
        # ">>> Yaw >>>"
        # ">>> Ultrasonic Sensors Detect >>>"
        # ">>> Encoders >>>"
        # ">>> Stepper position >>>"
        # ">>State Logic  >>"
        # "Adds a 15 second delay to the startup process \nfor the NavX to calibrate"
        n110 = Wait (ms)(milliseconds to wait=u32 1000) -> ()  [unwired: 1 out]
      }
      frame "NO ACTION", Default {
        (unwired) u8 0 ("y Stepper value")
        (unwired) TRUE ("Latch")
        (unwired) navX_type_def."Read Values" ("Mode")
        (unwired) MOTOR_CONTROL_NO_PID_Type_Def."Latch" ("Direction")
        # ">>> Object detection >>>"
        # ">>> Yaw >>>"
        # ">>> Ultrasonic Sensors Detect >>>"
        # ">>> Encoders >>>"
        # ">>> Stepper position >>>"
        # ">>State Logic  >>"
        n111 = case shown="4" w2507 {
          tunnel: [0 100] -> w2509
          frame 1, Default {
          }
          frame 4 {
          }
        }
      }
      frame "----RESET CASES----" {
        (unwired) I2C_MASTER_Type_Def."Last State" ("Arduino Mode")
        # ">>> Object detection >>>"
        # ">>> Yaw >>>"
        # ">>> Ultrasonic Sensors Detect >>>"
        # ">>> Encoders >>>"
        # ">>> Stepper position >>>"
        # ">>State Logic  >>"
      }
      frame "RESET ENCODERS" {
        # ">>> Object detection >>>"
        # ">>> Yaw >>>"
        # ">>> Ultrasonic Sensors Detect >>>"
        # ">>> Encoders >>>"
        # ">>> Stepper position >>>"
        # ">>State Logic  >>"
        n112 = call "MOTOR CONTROL WITH PID AE.vi"("Direction"=MOTOR_CONTROL_WITH_PID_AE_DIRECTION_TYPE_DEF."reset encoders", "AE Mode"=MOTOR_CONTROL_WITH_PID_AE_DATA_MODE_TYPE_DEF."Write to AE") -> ()  [unwired: 2 in, 1 out]
      }
      frame "RESET FLAGS" {
        (unwired) I2C_MASTER_Type_Def."Last State" ("Arduino Mode")
        # "Resets any software variables\nand/or non-critical states"
        n113 = Wait (ms)(milliseconds to wait=u32 20) -> ()  [unwired: 1 out]
        n114 = Bundle By Name(cluster=w2541, "Time up flag"=FALSE, "SET TIME TO CHECK"=0.0) -> (w2540:T15)
        n115 = Bundle By Name(cluster=w2558, "Recognized Object"=FALSE, "Object X coordinate"=0.0, "Object Y coordinate"=0.0) -> (w2557:T2)
        n116 = Bundle By Name(cluster=w2548, "y Stepper Position"=u8 0, "z Stepper Position"=u8 0) -> (w2547:T17)
        n117 = Bundle By Name(cluster=w2553, "xDistance"=0.0, "yDistance"=0.0, "wDistance"=0.0) -> (w2552:T20)
        n118 = Bundle By Name(cluster=w2565, "PING_A"=u8 0, "PING_B"=u8 0, "PING_C"=u8 0, "PING_D"=u8 0) -> (w2564:T19)
        n119 = Bundle By Name(cluster=w2544, "Yaw"=0.0) -> (w2543:T16)
      }
      frame "RESET YAW" {
        n120 = Wait (ms)(milliseconds to wait=u32 100) -> ()  [unwired: 1 out]
        n121 = call "navX reading VI.vi"("Mode"=navX_type_def."Zero Yaw") -> ()  [unwired: 2 in, 4 out]
      }
      frame "RESET ARM" {
        n122 = call "Arduino Interfacing VI.vi"("Data to Write"=I2C_MASTER_WRITE_NEW_Type_Def."Soft Reset", "AE Mode"=Arduino_Interfacing."Write to Arduino") -> ()  [unwired: 2 in, 2 out]
      }
      frame "--------CAM STATES-------" {
      }
      frame "OPEN IMAQ REF" {
        # ">>> Line Sensor Cluster>>>"
        # ">>State Logic  >>"
        # ">>> Time cluster >>>"
        # ">>> Object detection >>>"
        # ">>> Yaw >>>"
        # ">>> Ultrasonic Sensors Detect >>>"
        # ">>> Encoders >>>"
        # ">>> Stepper position >>>"
        # ">>> IR Sensors >>>"
        n123 = call "IMAQ Reference AE.vi"("IMAQ AE States"=IMAQ_Reference_AE."Initialize AE") -> ()  [unwired: 1 in, 2 out]
      }
      frame "OPEN LOG CAM" {
        n124 = call "Webcam AE.vi"("Session In"=T35 "cam0", "Camera states"=Webcam_AE."Initialize Camera") -> ("error out"=w2617:errorcluster, "Session Out"=w2616:T35)  [unwired: 1 in, 1 out]
        n125 = call "Webcam AE.vi"("error in (no error)"=w2617, "Session In"=w2616, "Camera states"=Webcam_AE."Open Camera") -> ()  [unwired: 3 out]
      }
      frame "OPEN LIFE CAM" {
        n126 = call "Webcam AE.vi"("Session In"=T35 "cam1", "Camera states"=Webcam_AE."Initialize Camera") -> ("error out"=w2632:errorcluster, "Session Out"=w2631:T35)  [unwired: 1 in, 1 out]
        n127 = call "Webcam AE.vi"("error in (no error)"=w2632, "Session In"=w2631, "Camera states"=Webcam_AE."Open Camera") -> ()  [unwired: 3 out]
      }
      frame "CAM ACQ" {
        # ">>State Logic  >>"
        # ">>> Time cluster >>>"
        # ">>> Yaw >>>"
        # ">>> Stepper position >>>"
        # ">>> Encoders >>>"
        # ">>> Object detection >>>"
        # ">>> Ultrasonic Sensors Detect >>>"
        n128 = call "Webcam AE.vi"("Camera states"=Webcam_AE."Continuous Acquisition") -> ()  [unwired: 2 in, 3 out]
      }
      frame "CAM CLOSE" {
        # ">>State Logic  >>"
        # ">>> Time cluster >>>"
        # ">>> Yaw >>>"
        # ">>> Stepper position >>>"
        # ">>> Encoders >>>"
        # ">>> Object detection >>>"
        # ">>> Ultrasonic Sensors Detect >>>"
        n129 = call "Webcam AE.vi"("Camera states"=Webcam_AE."Close Camera") -> ()  [unwired: 2 in, 3 out]
      }
      frame "PROCESS IMAGE" {
        # ">> Item Selection Bias >>"
        # ">> Item Selection Bias >>"
        # ">>State Logic  >>"
        # ">>> Time cluster >>>"
        # ">>> Yaw >>>"
        # ">>> Stepper position >>>"
        # ">>> Encoders >>>"
        # ">>> Object detection >>>"
        # ">>> Ultrasonic Sensors Detect >>>"
        n130 = call "Webcam AE.vi"("Camera states"=Webcam_AE."Retrieve Image") -> ("error out"=w2677:errorcluster, "Image Out"=w2678:T41)  [unwired: 2 in, 1 out]
        n131 = call "IMAQ Reference AE.vi"("IMAQ AE States"=IMAQ_Reference_AE."Get IMAQ Reference") -> ("Image Out"=w2667:T41)  [unwired: 1 in, 1 out]
        n132 = call "Object Detection SubVI.vi"("Error In"=w2677, "Mode"=w2664, "Image Dest"=w2667, "Image in"=w2678) -> ("Error out"=w2665:errorcluster, "Object Center Coordinates"=w2674:cluster{"x":sgl, "y":sgl}, "Object detection cluster"=w2670:T42)  [unwired: 1 out]
        n133 = Unbundle By Name(w2670) -> ("Object detected?"=w2671:bool)
        n134 = Unbundle By Name(w2674) -> ("x"=w2673:sgl, "y"=w2672:sgl)
        n135 = Bundle By Name(cluster=w2676, "Recognized Object"=w2671, "Object X coordinate"=w2673, "Object Y coordinate"=w2672) -> (w2675:T2)
      }
      frame "DISPOSE CAM BUFFERS" {
        # ">> Item Selection Bias >>"
        # ">>> Line Sensor Cluster>>>"
        # ">>> IR Sensors >>>"
        # ">>State Logic  >>"
        # ">>> Time cluster >>>"
        # ">>> Yaw >>>"
        # ">>> Stepper position >>>"
        # ">>> Encoders >>>"
        # ">>> Object detection >>>"
        # ">>> Ultrasonic Sensors Detect >>>"
        n136 = call "Webcam AE.vi"("Camera states"=Webcam_AE."Dispose Camera Image Buffer") -> ()  [unwired: 2 in, 3 out]
      }
      frame "DISPOSE PROC BUFFERS" {
        # ">>> Line Sensor Cluster>>>"
        # ">>State Logic  >>"
        # ">>> IR Sensors >>>"
        # ">>> Time cluster >>>"
        # ">>> Object detection >>>"
        # ">>> Yaw >>>"
        # ">>> Ultrasonic Sensors Detect >>>"
        # ">>> Encoders >>>"
        # ">>> Stepper position >>>"
        n137 = call "IMAQ Reference AE.vi"("IMAQ AE States"=IMAQ_Reference_AE."Dispose Processing Buffer") -> ()  [unwired: 1 in, 2 out]
      }
      frame "-----ARM ACTIONS-----" {
      }
      frame "CLOSE CLAW" {
        n138 = call "Arduino Interfacing VI.vi"("Data to Write"=I2C_MASTER_WRITE_NEW_Type_Def."Close Claw", "AE Mode"=Arduino_Interfacing."Write to Arduino") -> ()  [unwired: 2 in, 2 out]
      }
      frame "OPEN CLAW" {
        n139 = call "Arduino Interfacing VI.vi"("Data to Write"=I2C_MASTER_WRITE_NEW_Type_Def."Open Claw", "AE Mode"=Arduino_Interfacing."Write to Arduino") -> ()  [unwired: 2 in, 2 out]
      }
      frame "Z STEPPER CAM HEIGHT" {
        n140 = call "Arduino Interfacing VI.vi"("Data to Write"=I2C_MASTER_WRITE_NEW_Type_Def."zStepper 6k", "AE Mode"=Arduino_Interfacing."Write to Arduino") -> ()  [unwired: 2 in, 2 out]
      }
      frame "Z STEPPER GRAB HEIGHT" {
        # ">>State Logic  >>"
        # ">>> Time cluster >>>"
        # ">>> Yaw >>>"
        # ">>> Stepper position >>>"
        # ">>> Encoders >>>"
        # ">>> Object detection >>>"
        # ">>> Ultrasonic Sensors Detect >>>"
        n141 = call "Arduino Interfacing VI.vi"("Data to Write"=I2C_MASTER_WRITE_NEW_Type_Def."zStepper 100", "AE Mode"=Arduino_Interfacing."Write to Arduino") -> ()  [unwired: 2 in, 2 out]
      }
      frame "Z STEPPER BOX HEIGHT" {
        # ">>> IR Sensors >>>"
        # ">>> Time cluster >>>"
        # ">>> Yaw >>>"
        # ">>> Stepper position >>>"
        # ">>> Encoders >>>"
        # ">>> Object detection >>>"
        # ">>> Ultrasonic Sensors Detect >>>"
        n142 = call "Arduino Interfacing VI.vi"("Data to Write"=I2C_MASTER_WRITE_NEW_Type_Def."zStepper 4k", "AE Mode"=Arduino_Interfacing."Write to Arduino") -> ()  [unwired: 2 in, 2 out]
      }
      frame "Y STEPPER CONTROL" {
        # ">>State Logic  >>"
        # ">>> yStepper command>>>"
        # ">>> Time cluster >>>"
        # ">>> Yaw >>>"
        # ">>> Stepper position >>>"
        # ">>> Encoders >>>"
        # ">>> Object detection >>>"
        # ">>> Ultrasonic Sensors Detect >>>"
        n143 = Unbundle By Name(w2782) -> ("yStepper desired"=w2781:u8)
        n144 = call "Arduino Interfacing VI.vi"("y Stepper value"=w2781, "Data to Write"=I2C_MASTER_WRITE_NEW_Type_Def."yStepper control", "AE Mode"=Arduino_Interfacing."Write to Arduino") -> ()  [unwired: 1 in, 2 out]
      }
      frame "READ STEPPER VALUES" {
        # ">>State Logic  >>"
        # ">>> Time cluster >>>"
        # ">>> Yaw >>>"
        # ">>> Stepper position >>>"
        # ">>> Encoders >>>"
        # ">>> Object detection >>>"
        # ">>> Ultrasonic Sensors Detect >>>"
        n145 = call "Arduino Interfacing VI.vi"("AE Mode"=Arduino_Interfacing."Read From Arduino") -> ("Arduino Data"=w2799:T8)  [unwired: 3 in, 1 out]
        n146 = Unbundle By Name(w2799) -> ("y Stepper Position"=w2798:u8, "z Stepper Position"=w2797:u8)
        n147 = Bundle By Name(cluster=w2802, "y Stepper Position"=w2798, "z Stepper Position"=w2797) -> (w2801:T17)
      }
      frame " -----TIMING-----" {
        # ">>State Logic  >>"
        # ">>> Time cluster >>>"
        # ">>> Yaw >>>"
        # ">>> Stepper position >>>"
        # ">>> Encoders >>>"
        # ">>> Object detection >>>"
        # ">>> Ultrasonic Sensors Detect >>>"
      }
      frame "SET TIMER 1" {
        # ">>State Logic  >>"
        # ">>> Time cluster >>>"
        # ">>> Yaw >>>"
        # ">>> Stepper position >>>"
        # ">>> Encoders >>>"
        # ">>> Object detection >>>"
        # ">>> Ultrasonic Sensors Detect >>>"
        n148 = call "Elasped Timer.vi"("Time Setting"=1.0, "Action"=Elapsed_timer_control."Initialize") -> ()  [unwired: 6 in, 4 out]
        n149 = Bundle By Name(cluster=w2824, "Time up flag"=FALSE) -> (w2822:T15)
      }
      frame "SET TIMER 2" {
        # ">>State Logic  >>"
        # ">>> Time cluster >>>"
        # ">>> Yaw >>>"
        # ">>> Stepper position >>>"
        # ">>> Encoders >>>"
        # ">>> Object detection >>>"
        # ">>> Ultrasonic Sensors Detect >>>"
        n150 = call "Elasped Timer.vi"("Time Setting"=2.0, "Action"=Elapsed_timer_control."Initialize") -> ()  [unwired: 6 in, 4 out]
        n151 = Bundle By Name(cluster=w2838, "Time up flag"=FALSE) -> (w2836:T15)
      }
      frame "SET TIMER 3" {
        # ">>State Logic  >>"
        # ">>> Time cluster >>>"
        # ">>> Yaw >>>"
        # ">>> Stepper position >>>"
        # ">>> Encoders >>>"
        # ">>> Object detection >>>"
        # ">>> Ultrasonic Sensors Detect >>>"
        n152 = call "Elasped Timer.vi"("Time Setting"=3.0, "Action"=Elapsed_timer_control."Initialize") -> ()  [unwired: 6 in, 4 out]
        n153 = Bundle By Name(cluster=w2852, "Time up flag"=FALSE) -> (w2850:T15)
      }
      frame "SET TIMER 4" {
        # ">>State Logic  >>"
        # ">>> Time cluster >>>"
        # ">>> Yaw >>>"
        # ">>> Stepper position >>>"
        # ">>> Encoders >>>"
        # ">>> Object detection >>>"
        # ">>> Ultrasonic Sensors Detect >>>"
        n154 = call "Elasped Timer.vi"("Time Setting"=4.0, "Action"=Elapsed_timer_control."Initialize") -> ()  [unwired: 6 in, 4 out]
        n155 = Bundle By Name(cluster=w2866, "Time up flag"=FALSE) -> (w2864:T15)
      }
      frame "SET TIMER 5" {
        # ">>State Logic  >>"
        # ">>> Time cluster >>>"
        # ">>> Yaw >>>"
        # ">>> Stepper position >>>"
        # ">>> Encoders >>>"
        # ">>> Object detection >>>"
        # ">>> Ultrasonic Sensors Detect >>>"
        n156 = call "Elasped Timer.vi"("Time Setting"=5.0, "Action"=Elapsed_timer_control."Initialize") -> ()  [unwired: 6 in, 4 out]
        n157 = Bundle By Name(cluster=w2880, "Time up flag"=FALSE) -> (w2878:T15)
      }
      frame "START TIMER" {
        # ">>State Logic  >>"
        # ">>> Time cluster >>>"
        # ">>> Yaw >>>"
        # ">>> Stepper position >>>"
        # ">>> Encoders >>>"
        # ">>> Object detection >>>"
        # ">>> Ultrasonic Sensors Detect >>>"
        n158 = call "Elasped Timer.vi"("Action"=Elapsed_timer_control."Start") -> ("Time Out?!"=w2890:bool)  [unwired: 7 in, 3 out]
        n159 = Bundle By Name(cluster=w2893, "Time up flag"=w2890) -> (w2892:T15)
      }
    }
    "State Logic" <- w237
    "Image Processing Error" <- w204
    n160 = local read "TASK ENABLE"() -> (w231:bool)
    n161 = Not(x=w231) -> (.not. x?=w230:bool)
    n162 = case shown="True" w238 {
      tunnel: w242 -> [w269 w309]
      tunnel: w246 -> [w265 w311]
      tunnel: [w269 w309] -> w251
      tunnel: [w265 w312] -> w250
      tunnel: w247 -> [_ w307]
      tunnel: w249 -> [_ w308]
      tunnel: w244 -> [w268 w314]
      tunnel: [w268 w314] -> w243
      tunnel: "STOP TASK" -> [_ w297]
      tunnel: w237 -> [w267 w313]
      tunnel: [w267 w310] -> w236
      tunnel: w233 -> [w266 w303]
      tunnel: [w266 w303] -> w232
      tunnel: w230 -> [_ w298]
      tunnel: [w264 w295] -> w229
      tunnel: w228 -> [w264 w294]
      tunnel: w226 -> [w263 w291]
      tunnel: [w263 w291] -> w225
      tunnel: w223 -> [w262 w287]
      tunnel: [w262 w287] -> w222
      tunnel: w220 -> [w261 w285]
      tunnel: [w261 w285] -> w219
      tunnel: w217 -> [w260 w283]
      tunnel: [w260 w283] -> w216
      tunnel: w215 -> [w259 w282]
      tunnel: [w259 w281] -> w214
      tunnel: [_ w279] -> w213
      tunnel: w211 -> [w258 w277]
      tunnel: [w258 w277] -> w210
      tunnel: w209 -> [w257 w276]
      tunnel: [w257 w275] -> w208
      tunnel: w206 -> [w256 w272]
      tunnel: [w256 w272] -> w205
      tunnel: [w255 w271] -> w203
      tunnel: w201 -> [w255 w270]
      frame False {
        # ">> Item Selection Bias >>"
        # ">>State Logic Queue Reference >>"
        # ">>Action states Queue Reference >>"
        # ">>True Stop Next State >>"
        # ">>State Logic  >>"
        # ">>> IR Sensors >>>"
        # ">>> Line Sensor Cluster>>>"
        # ">>> Line Sensor Cluster>>>"
        # ">>> Motor control cluster >>>"
        # ">>> yStepper command>>>"
        # ">>> Motor control cluster >>>"
        # ">>> yStepper command>>>"
        # ">>> Motor control cluster >>>"
        # ">>> IR Sensors >>>"
        # ">>> IR Sensors >>>"
        # ">>> yStepper command>>>"
        # ">>> Time cluster >>>"
        # ">>> Yaw >>>"
        # ">>> Stepper position >>>"
        # ">>> Encoders >>>"
        # ">>> Object detection >>>"
        # ">>> Ultrasonic Sensors Detect >>>"
        # ">>> Time cluster >>>"
        # ">>> Yaw >>>"
        # ">>> Stepper position >>>"
        # ">>> Encoders >>>"
        # ">>> Object detection >>>"
        # ">>> Ultrasonic Sensors Detect >>>"
      }
      frame True {
        # ">> Item Selection Bias >>"
        # ">>> IR Sensors >>>"
        # ">>> Line Sensor Cluster>>>"
        # ">>> Line Sensor Cluster>>>"
        # ">>> Motor control cluster >>>"
        # ">>> yStepper command>>>"
        # ">>> IR Sensors >>>"
        # ">>> Motor control cluster >>>"
        # ">>State Logic Queue Reference >>"
        # ">>Timeout>>"
        # ">>> yStepper command>>>"
        # ">>> Time cluster >>>"
        # ">>> Object detection >>>"
        # ">>> Yaw >>>"
        # ">>> Ultrasonic Sensors Detect >>>"
        # ">>> Encoders >>>"
        # ">>> Stepper position >>>"
        # ">>State Logic  >>"
        # ">>True Stop Next State >>"
        # ">>Action Queue>>"
        # ">> Manual override >>"
        # ">>> Time cluster >>>"
        # ">>> Yaw >>>"
        # ">>> Stepper position >>>"
        # ">>> Encoders >>>"
        # ">>> Object detection >>>"
        # ">>> Ultrasonic Sensors Detect >>>"
        # ">>Action Queue>>"
        # ">>State Logic Queue Reference >>"
        n163 = Or(x=w297, y=w298) -> (x .or. y?=w296:bool)
        n164 = Unbundle By Name(w277) -> ("Left IR Sensor"=w278:dbl, "Arm IR Sensor"=w274:dbl)
        "Left IR Sensor" <- w278
        "Arm IR Sensor" <- w274
        n165 = Unbundle By Name(w283) -> ("Time up flag"=w284:bool)
        "Time up flag" <- w284
        n166 = Unbundle By Name(w285) -> ("Yaw"=w286:dbl, "Compass"=w280:dbl)
        n167 = Unbundle By Name(w287) -> ("y Stepper Position"=w289:u8, "z Stepper Position"=w288:u8)
        n168 = Unbundle By Name(w303) -> ("xDistance"=w300:dbl, "yDistance"=w301:dbl, "wDistance"=w302:dbl)
        n169 = Unbundle By Name(w291) -> ("Recognized Object"=w290:bool, "Object X coordinate"=w293:dbl, "Object Y coordinate"=w292:dbl)
        n170 = Unbundle By Name(w314) -> ("PING_A"=w306:u8, "PING_B"=w305:u8, "PING_C"=w304:u8, "PING_D"=w299:u8)
        n171 = Unbundle By Name(w272) -> ("Line Detected?"=w273:bool)
        n172 = case shown="4, Default" w313 {
          tunnel: [w319 w331 w345 w356 w474 w489 w526 w580 w623 w671 w715 w770 w818 w859 w920 w966 w1007 w1056 w1099 w1152 w1190 w1242 w1286 w1330 w1360 w1378 w1424 w1465 w1514 w1567 w1606 w1655 w1698 w1751 w1789 w1841 w1877 w1926 w1969 w2015 w2061 w2105 w2160] -> w312
          tunnel: w311 -> [w319 w334 w346 w359 w476 w490 w535 w578 w627 w672 w721 w763 w821 w866 w910 w969 w1013 w1055 w1102 w1142 w1196 w1232 w1281 w1321 w1360 w1368 w1427 w1471 w1513 w1566 w1612 w1654 w1701 w1741 w1795 w1831 w1881 w1933 w1974 w2020 w2066 w2109 w2158]
          tunnel: [State_Type_Definitions."Idle" ("Enum") State_Type_Definitions."Idle" ("Enum") w341 w358 State_Type_Definitions."Shutdown" ("Enum") w491 w533 w581 w624 w670 w716 w769 w819 w861 w919 w967 w1014 w1057 w1101 w1151 w1197 w1241 w1287 w1322 State_Type_Definitions."Idle" ("Enum") w1377 w1425 w1472 w1515 w1568 w1613 w1656 w1700 w1750 w1796 w1840 w1878 w1927 w1970 w2016 w2062 w2106 w2161] -> w310
          tunnel: w309 -> [_ _ w344 w362 _ w496 w529 w577 w628 w679 w720 w767 w822 w865 w917 w964 w1012 w1053 w1103 w1149 w1195 w1239 w1284 w1329 _ w1375 w1422 w1470 w1511 w1564 w1611 w1652 w1702 w1748 w1794 w1838 w1885 w1932 w1977 w2023 w2069 w2113 w2157]
          tunnel: w308 -> [_ _ _ w361 _ w495 w528 w576 w629 w678 w719 w766 w815 w864 w916 w963 w1011 w1052 w1104 w1148 w1194 w1238 w1283 w1327 _ w1374 w1421 w1469 w1510 w1563 w1610 w1651 w1703 w1747 w1793 w1837 w1880 w1931 w1976 w2022 w2068 w2108 w2156]
          tunnel: w307 -> [_ _ w343 w357 _ w494 w527 w575 w630 w677 w718 w765 w814 w863 w918 w965 w1010 w1051 w1105 w1150 w1193 w1240 w1282 w1328 _ w1376 w1423 w1468 w1509 w1562 w1609 w1650 w1704 w1749 w1792 w1839 w1884 w1930 w1975 w2021 w2067 w2112 w2155]
          tunnel: w296 -> [_ _ _ _ _ w488 w534 w574 w631 w674 w714 w768 w820 w867 w911 w970 w1008 w1054 w1106 w1143 w1191 w1233 w1285 w1325 _ w1369 w1428 w1466 w1512 w1565 w1607 w1653 w1705 w1742 w1790 w1832 w1883 w1925 w1973 w2019 w2065 w2111 w2154]
          tunnel: w306 -> [_ _ _ _ _ _ _ _ _ _ _ _ _ _ _ _ _ _ _ _ _ _ _ _ _ _ _ _ _ _ _ _ _ _ _ _ _ _ _ _ _ _ _]
          tunnel: w305 -> [_ _ _ _ _ _ _ w573 _ _ _ w759 w803 w857 _ w956 _ _ _ _ _ _ _ _ _ _ w1414 _ _ _ _ _ _ _ _ _ _ _ _ _ _ _ _]
          tunnel: w304 -> [_ _ _ _ _ _ _ w572 _ _ _ w760 w804 w858 _ w957 _ _ _ _ _ _ _ _ _ _ w1415 _ _ _ _ _ _ _ _ _ _ _ _ _ _ _ _]
          tunnel: w302 -> [_ _ _ _ _ _ _ _ _ w676 _ _ _ _ _ _ _ _ _ _ _ _ _ _ _ _ _ _ _ _ _ _ _ _ _ _ _ _ _ _ _ _ _]
          tunnel: w301 -> [_ _ _ _ _ w487 _ _ w622 _ _ _ _ w862 _ _ _ _ _ _ _ _ _ _ _ _ _ _ _ _ _ _ _ _ _ _ _ _ _ _ _ _ _]
          tunnel: w300 -> [_ _ _ _ _ _ _ _ _ _ _ _ w809 _ _ _ _ _ _ _ _ _ _ _ _ _ _ _ _ w1553 _ _ _ _ _ _ _ _ _ _ w2059 _ _]
          tunnel: w299 -> [_ _ _ _ _ _ _ _ _ _ _ _ _ _ _ _ _ _ _ _ _ _ _ _ _ _ _ _ _ _ _ _ _ _ _ _ _ _ _ _ _ _ _]
          tunnel: [State_Type_Definitions."Idle" ("Enum") State_Type_Definitions."Idle" ("Enum") State_Type_Definitions."Idle" ("Enum") State_Type_Definitions."Idle" ("Enum") State_Type_Definitions."Shutdown" ("Enum") w484 w532 w579 w625 w667 w713 w762 w817 w860 w921 w968 w1006 w1058 w1100 w1153 w1189 w1243 w1288 w1323 w1362 w1379 w1426 w1464 w1516 w1569 w1605 w1657 w1699 w1752 w1788 w1842 w1879 w1928 w1972 w2018 w2064 w2107 w2159] -> w295
          tunnel: w294 -> [_ _ w341 _ _ _ _ _ _ _ _ _ _ _ _ _ _ _ _ _ _ _ _ _ w1362 _ _ _ _ _ _ _ _ _ _ _ _ _ _ _ _ _ _]
          tunnel: w290 -> [_ _ _ _ _ _ _ _ _ _ _ _ _ _ _ _ _ _ _ _ _ _ _ w1324 _ _ _ _ _ _ _ _ _ _ _ _ _ _ _ _ _ _ _]
          tunnel: w293 -> [_ _ _ _ _ _ _ _ _ _ _ _ _ _ _ _ _ _ _ _ _ _ _ _ _ _ _ _ _ w1559 _ _ _ _ _ _ _ _ _ _ _ _ _]
          tunnel: w292 -> [_ _ _ _ _ _ _ _ _ _ _ _ _ _ _ _ _ _ w1095 _ _ _ _ _ _ _ _ _ _ _ _ _ w1694 _ _ _ _ _ _ _ _ _ _]
          tunnel: w289 -> [_ _ _ _ _ _ _ _ _ _ _ _ _ _ _ _ _ _ w1094 _ _ _ _ _ _ _ _ _ _ _ _ _ w1693 _ _ _ _ _ _ _ _ _ _]
          tunnel: w288 -> [_ _ _ _ _ _ w531 _ _ _ w711 _ _ _ w914 _ _ _ _ w1146 _ w1236 w1280 _ _ w1372 _ _ _ _ _ _ _ w1745 _ w1835 w1882 _ _ _ _ w2110 _]
          tunnel: w286 -> [_ _ _ _ _ _ _ _ _ _ _ _ _ _ _ _ _ _ _ _ _ _ _ _ _ _ _ _ _ _ _ _ _ _ _ _ _ _ _ _ _ _ _]
          tunnel: w284 -> [_ _ _ _ _ _ _ _ _ _ _ _ _ _ _ _ w1004 w1048 _ _ w1187 _ _ _ _ _ _ w1462 w1506 _ w1603 w1647 _ _ w1786 _ _ _ _ _ _ _ _]
          tunnel: w282 -> [w317 w329 w340 w354 w472 w483 w530 w571 w626 w666 w712 w761 w813 w856 w909 w961 w1005 w1049 w1097 w1141 w1188 w1231 w1277 w1320 w1363 w1367 w1419 w1463 w1507 w1560 w1604 w1648 w1696 w1740 w1787 w1830 w1876 w1929 w1971 w2017 w2063 w2104 w2153]
          tunnel: [w317 w328 w340 w354 w472 w483 w530 w571 w626 w666 w712 w761 w813 w856 w909 w961 w1005 w1049 w1096 w1141 w1188 w1231 w1277 w1320 w1363 w1367 w1419 w1463 w1507 w1560 w1604 w1648 w1695 w1740 w1787 w1830 w1876 w1929 w1971 w2017 w2063 w2104 w2153] -> w281
          tunnel: w280 -> [_ _ _ _ _ _ _ _ _ _ _ _ _ _ _ _ _ _ _ _ _ _ _ _ _ _ _ _ _ _ _ _ _ _ _ _ _ w1924 _ _ _ _ _]
          tunnel: [_ _ _ TRUE _ _ _ _ _ _ _ _ _ _ _ _ _ _ _ _ _ _ _ _ _ _ _ _ _ _ _ _ _ _ _ _ _ _ _ _ _ _ _] -> w279
          tunnel: w278 -> [_ _ _ _ _ _ _ _ _ _ _ _ _ _ _ _ _ _ _ _ _ _ _ _ _ _ _ _ _ _ _ _ _ _ _ _ _ _ _ _ _ _ _]
          tunnel: w276 -> [w316 w326 w339 w352 w471 w482 w525 w570 w619 w665 w708 w754 w802 w855 w908 w954 w1003 w1047 w1091 w1140 w1186 w1230 w1276 w1319 w1364 w1366 w1412 w1461 w1505 w1556 w1602 w1646 w1690 w1739 w1785 w1829 w1875 w1920 w1968 w2014 w2060 w2103 w2152]
          tunnel: [w316 w325 w339 w352 w471 w482 w525 w570 w619 w665 w708 w754 w802 w855 w908 w954 w1003 w1047 w1091 w1140 w1186 w1230 w1276 w1319 w1364 w1366 w1412 w1461 w1505 w1555 w1602 w1646 w1690 w1739 w1785 w1829 w1875 w1920 w1968 w2014 w2060 w2103 w2152] -> w275
          tunnel: w274 -> [_ _ _ _ _ _ _ _ _ _ _ _ _ _ _ _ _ _ _ _ _ _ _ _ _ _ _ _ _ _ _ _ _ _ _ _ _ _ _ w2012 _ _ w2151]
          tunnel: w273 -> [_ _ _ _ _ _ _ _ _ _ _ _ _ _ _ _ _ _ _ _ _ _ _ _ _ _ _ _ _ _ _ _ _ _ _ _ _ _ w1967 _ _ _ _]
          tunnel: [w315 w321 w338 w351 w470 w481 w524 w569 w618 w664 w707 w753 w801 w854 w907 w953 w1002 w1046 w1090 w1139 w1185 w1229 w1275 w1318 w1359 w1365 w1411 w1460 w1504 w1548 w1601 w1645 w1689 w1738 w1784 w1828 w1874 w1919 w1966 w2010 w2056 w2102 w2148] -> w271
          tunnel: w270 -> [w315 w321 w338 _ w470 w481 w524 w569 w618 w664 w707 w753 w801 w854 w907 w953 w1002 w1046 w1090 w1139 w1185 w1229 w1275 w1318 w1359 w1365 w1411 w1460 w1504 w1548 w1601 w1645 w1689 w1738 w1784 w1828 w1874 w1919 w1966 w2010 w2056 w2102 w2148]
          frame 0 {
            # ">>> yStepper command>>>"
          }
          frame 1 {
            # ">>> yStepper command>>>"
            n173 = for {
              shift-right: [w337] -> w331
              shift-left: w334 -> [w336]
              tunnel: string[] ["INIT", "RESET ARM", "RESET FLAGS", "RESET YAW", "NAVX CALIBRATE"] -> [w335] mode=indexing
              n174 = Enqueue Element(queue=w336, element=w335) -> (queue out=w337:refnum<queue>)  [unwired: 2 in, 2 out]
            }
            n175 = Bundle By Name(cluster=w329, "yStepper desired"=u8 0) -> (w328:T14)
            n176 = Bundle By Name(cluster=w326, "ySpeed"=0.0, "xSpeed"=0.0, "wSpeed"=0.0) -> (w325:T12)
          }
          frame 3 {
            # ">>> Motor control cluster >>>"
            # ">>> yStepper command>>>"
            n177 = Flush Queue(queue=w344, error in (no error)=w343) -> ()  [unwired: 3 out]
            n178 = for {
              shift-right: [w350] -> w345
              shift-left: w346 -> [w349]
              tunnel: string[] ["STOP", "RESET ENCODERS", "RESET YAW", "RESET ARM", "RESET FLAGS", "DISPOSE CAM BUFFERS", "DISPOSE PROC BUFFERS", "CAM CLOSE", ""] -> [w348] mode=indexing
              n179 = Enqueue Element(queue=w349, element=w348) -> (queue out=w350:refnum<queue>)  [unwired: 2 in, 2 out]
            }
          }
          frame 4, Default {
            # ">>> yStepper command>>>"
            n180 = Dequeue Element(queue=w362, timeout in ms (-1)=w361, error in (no error)=w357) -> (element=w360:T1)  [unwired: 3 out]
            n181 = case shown="\"Start Task 1\"" w360 {
              tunnel: [w365 w373 w381 w389 w397 w405 w413 w421 w429 w436 w446 w454 w461 w464] -> w356
              tunnel: w359 -> [w366 w374 w382 w390 w398 w406 w414 w422 w430 w437 w445 w453 w461 w465]
              tunnel: [State_Type_Definitions."Task 1" ("Enum") State_Type_Definitions."Task 2:Raise Arm" ("Enum") State_Type_Definitions."Task 3" ("Enum") State_Type_Definitions."Task 4_A" ("Enum") State_Type_Definitions."Task 5A: ARM CAM HEIGHT" ("Enum") State_Type_Definitions."Task 6_A" ("Enum") State_Type_Definitions."Task 8A: RAISE ARM" ("Enum") State_Type_Definitions."Task 8A: RAISE ARM" ("Enum") State_Type_Definitions."Task 8A: RAISE ARM" ("Enum") State_Type_Definitions."Task 8A: RAISE ARM" ("Enum") State_Type_Definitions."Task 9A: Raise Arm" ("Enum") State_Type_Definitions."Task A: RAISE ARM TO HEIGHT" ("Enum") State_Type_Definitions."Idle" ("Enum") State_Type_Definitions."Shutdown" ("Enum")] -> w358
              tunnel: [enum16{"Ball", "Soap", "Gel", "Pipe", "None"}."None" ("Object recognition mode") enum16{"Ball", "Soap", "Gel", "Pipe", "None"}."None" ("Object recognition mode") enum16{"Ball", "Soap", "Gel", "Pipe", "None"}."None" ("Object recognition mode") enum16{"Ball", "Soap", "Gel", "Pipe", "None"}."None" ("Object recognition mode") enum16{"Ball", "Soap", "Gel", "Pipe", "None"}."None" ("Object recognition mode") enum16{"Ball", "Soap", "Gel", "Pipe", "None"}."None" ("Object recognition mode") enum16{"Ball", "Soap", "Gel", "Pipe", "None"}."Ball" ("Object recognition mode") enum16{"Ball", "Soap", "Gel", "Pipe", "None"}."Gel" ("Object recognition mode") enum16{"Ball", "Soap", "Gel", "Pipe", "None"}."Pipe" ("Object recognition mode") enum16{"Ball", "Soap", "Gel", "Pipe", "None"}."Soap" ("Object recognition mode") enum16{"Ball", "Soap", "Gel", "Pipe", "None"}."None" ("Object recognition mode") enum16{"Ball", "Soap", "Gel", "Pipe", "None"}."None" ("Object recognition mode") enum16{"Ball", "Soap", "Gel", "Pipe", "None"}."None" ("Object recognition mode") enum16{"Ball", "Soap", "Gel", "Pipe", "None"}."None" ("Object recognition mode")] -> w351
              frame "Start Task 1" {
                n182 = for {
                  shift-right: [w370] -> w365
                  shift-left: w366 -> [w369]
                  tunnel: string[] ["RESET ENCODERS", "RESET YAW", "FORWARD", "READ ENCODERS"] -> [w368] mode=indexing
                  n183 = Enqueue Element(queue=w369, element=w368) -> (queue out=w370:refnum<queue>)  [unwired: 2 in, 2 out]
                }
              }
              frame "Start Task 2" {
                n184 = for {
                  shift-right: [w378] -> w373
                  shift-left: w374 -> [w377]
                  tunnel: string[] ["RESET ENCODERS", "RESET YAW", "READ ULTRASONIC", "ARDUINO - ULTRASONIC"] -> [w376] mode=indexing
                  n185 = Enqueue Element(queue=w377, element=w376) -> (queue out=w378:refnum<queue>)  [unwired: 2 in, 2 out]
                }
              }
              frame "Start Task 3" {
                n186 = for {
                  shift-right: [w386] -> w381
                  shift-left: w382 -> [w385]
                  tunnel: string[] ["RESET ENCODERS", "READ ENCODERS", "R-ACW"] -> [w384] mode=indexing
                  n187 = Enqueue Element(queue=w385, element=w384) -> (queue out=w386:refnum<queue>)  [unwired: 2 in, 2 out]
                }
              }
              frame "Start Task 4" {
                n188 = for {
                  shift-right: [w394] -> w389
                  shift-left: w390 -> [w393]
                  tunnel: string[] ["RESET YAW", "RESET ENCODERS", "RESET ARM", "RESET FLAGS", "", ""] -> [w392] mode=indexing
                  n189 = Enqueue Element(queue=w393, element=w392) -> (queue out=w394:refnum<queue>)  [unwired: 2 in, 2 out]
                }
              }
              frame "Start Task 5" {
                n190 = for {
                  shift-right: [w402] -> w397
                  shift-left: w398 -> [w401]
                  tunnel: string[] ["RESET YAW", "RESET ENCODERS", "READ STEPPER VALUES", "Z STEPPER CAM HEIGHT", "", ""] -> [w400] mode=indexing
                  n191 = Enqueue Element(queue=w401, element=w400) -> (queue out=w402:refnum<queue>)  [unwired: 2 in, 2 out]
                }
              }
              frame "Start Task 6" {
                n192 = for {
                  shift-right: [w410] -> w405
                  shift-left: w406 -> [w409]
                  tunnel: string[] ["OPEN LOG CAM ", "", "", "", "", ""] -> [w408] mode=indexing
                  n193 = Enqueue Element(queue=w409, element=w408) -> (queue out=w410:refnum<queue>)  [unwired: 2 in, 2 out]
                }
              }
              frame "Start Task 8 - BALL" {
                n194 = for {
                  shift-right: [w418] -> w413
                  shift-left: w414 -> [w417]
                  tunnel: string[] ["RESET YAW", "RESET ENCODERS", "RESET ARM", "RESET FLAGS"] -> [w416] mode=indexing
                  n195 = Enqueue Element(queue=w417, element=w416) -> (queue out=w418:refnum<queue>)  [unwired: 2 in, 2 out]
                }
              }
              frame "Start Task 8 - Gel" {
                n196 = for {
                  shift-right: [w426] -> w421
                  shift-left: w422 -> [w425]
                  tunnel: string[] ["RESET YAW", "RESET ENCODERS", "RESET ARM", "RESET FLAGS"] -> [w424] mode=indexing
                  n197 = Enqueue Element(queue=w425, element=w424) -> (queue out=w426:refnum<queue>)  [unwired: 2 in, 2 out]
                }
              }
              frame "Start Task 8 - Pipe" {
                n198 = for {
                  shift-right: [w434] -> w429
                  shift-left: w430 -> [w433]
                  tunnel: string[] ["RESET YAW", "RESET ENCODERS", "RESET ARM", "RESET FLAGS"] -> [w432] mode=indexing
                  n199 = Enqueue Element(queue=w433, element=w432) -> (queue out=w434:refnum<queue>)  [unwired: 2 in, 2 out]
                }
              }
              frame "Start Task 8 - Soap" {
                n200 = for {
                  shift-right: [w442] -> w436
                  shift-left: w437 -> [w441]
                  tunnel: string[] ["RESET YAW", "RESET ENCODERS", "RESET ARM", "RESET FLAGS"] -> [w440] mode=indexing
                  n201 = Enqueue Element(queue=w441, element=w440) -> (queue out=w442:refnum<queue>)  [unwired: 2 in, 2 out]
                }
              }
              frame "Start Task 9" {
                n202 = for {
                  shift-right: [w450] -> w446
                  shift-left: w445 -> [w449]
                  tunnel: string[] ["RESET ENCODERS", "READ ENCODERS", "Z STEPPER BOX HEIGHT"] -> [w448] mode=indexing
                  n203 = Enqueue Element(queue=w449, element=w448) -> (queue out=w450:refnum<queue>)  [unwired: 2 in, 2 out]
                }
              }
              frame "Start Task A" {
                n204 = for {
                  shift-right: [w458] -> w454
                  shift-left: w453 -> [w457]
                  tunnel: string[] ["RESET ENCODERS", "READ ENCODERS", "RESET YAW", "Z STEPPER BOX HEIGHT"] -> [w456] mode=indexing
                  n205 = Enqueue Element(queue=w457, element=w456) -> (queue out=w458:refnum<queue>)  [unwired: 2 in, 2 out]
                }
              }
              frame "None", Default {
              }
              frame "Exit" {
                n206 = for {
                  shift-right: [w469] -> w464
                  shift-left: w465 -> [w468]
                  tunnel: string[] ["STOP", "RESET ENCODERS", "RESET YAW", "EXIT"] -> [w467] mode=indexing
                  n207 = Enqueue Element(queue=w468, element=w467) -> (queue out=w469:refnum<queue>)  [unwired: 2 in, 2 out]
                }
              }
            }
          }
          frame 5 {
            # ">> Item Selection Bias >>"
            # ">>> yStepper command>>>"
            n208 = for {
              shift-right: [w480] -> w474
              shift-left: w476 -> [w479]
              tunnel: string[] ["INIT", "RESET ENCODERS", "RESET FLAGS", "CAM CLOSE", "DISPOSE BUFFERS", "EXIT", ""] -> [w478] mode=indexing
              n209 = Enqueue Element(queue=w479, element=w478) -> (queue out=w480:refnum<queue>)  [unwired: 2 in, 2 out]
            }
          }
          frame 6 {
            # ">>> yStepper command>>>"
            # "Use 250"
            n210 = Dequeue Element(queue=w496, timeout in ms (-1)=w495, error in (no error)=w494) -> (element=w493:T1)  [unwired: 3 out]
            n211 = Greater?(x=w487, y=265.0) -> (0:w485:bool)
            n212 = Or(x=w485, y=w488) -> (x .or. y?=w492:bool)
            n213 = case shown="\"Start Task 1\", Default" w493 {
              tunnel: w492 -> [w499 _]
              tunnel: [w503 State_Type_Definitions."True Stop" ("Enum")] -> w491
              tunnel: w490 -> [w500 w518]
              tunnel: [w498 w517] -> w489
              tunnel: [State_Type_Definitions."Idle" ("Enum") State_Type_Definitions."Shutdown" ("Enum")] -> w484
              frame "Start Task 1", Default {
                n214 = case shown="True" w499 {
                  tunnel: w500 -> [w506 w512]
                  tunnel: [w505 w510] -> w498
                  frame False {
                    n215 = for {
                      shift-right: [w508] -> w505
                      shift-left: w506 -> [w509]
                      tunnel: string[] ["READ ENCODERS", "READ NAVX", "FORWARD"] ("element") -> [w507] mode=indexing
                      n216 = Enqueue Element(queue=w509, element=w507) -> (queue out=w508:refnum<queue>)  [unwired: 2 in, 2 out]
                    }
                  }
                  frame True {
                    n217 = for {
                      shift-right: [w514] -> w510
                      shift-left: w512 -> [w515]
                      tunnel: string[] ["RESET YAW", "RESET ENCODERS", "STOP", ""] -> [w513] mode=indexing
                      n218 = Enqueue Element(queue=w515, element=w513) -> (queue out=w514:refnum<queue>)  [unwired: 2 in, 2 out]
                    }
                  }
                }
                n219 = Select(t=State_Type_Definitions."True Stop" ("Enum"), s=w499, f=State_Type_Definitions."Task 1" ("Enum")) -> (s? t:f=w503:u16)
              }
              frame "Exit" {
                n220 = for {
                  shift-right: [w522] -> w517
                  shift-left: w518 -> [w523]
                  tunnel: string[] ["STOP", "RESET ENCODERS", "RESET YAW", ""] -> [w521] mode=indexing
                  n221 = Enqueue Element(queue=w523, element=w521) -> (queue out=w522:refnum<queue>)  [unwired: 2 in, 2 out]
                }
              }
            }
          }
          frame 8 {
            # ">> Stepper height reeached >>"
            # ">>> yStepper command>>>"
            # ">> Manual override >>"
            n222 = Dequeue Element(queue=w529, timeout in ms (-1)=w528, error in (no error)=w527) -> (element=w538:T1)  [unwired: 3 out]
            n223 = Equal?(x=w531, y=u8 60) -> (x = y?=w536:bool)
            n224 = case shown="\"Start Task 1\", Default" w538 {
              tunnel: [w549 State_Type_Definitions."True Stop" ("Enum")] -> w533
              tunnel: [w547 w564] -> w526
              tunnel: w535 -> [w546 _]
              tunnel: w534 -> [w540 _]
              tunnel: [State_Type_Definitions."Idle" ("Enum") State_Type_Definitions."Shutdown" ("Enum")] -> w532
              tunnel: w536 -> [w539 _]
              frame "Start Task 1", Default {
                # ">> WIill proceed to part ii if not manual override >>"
                # ">>If ENABLE or Trigger is set to true>>"
                n225 = Or(x=w539, y=w540) -> (x .or. y?=w541:bool)
                n226 = case shown="True" w539 {
                  tunnel: [w552 w558] -> w547
                  tunnel: w546 -> [w551 w557]
                  frame False {
                    n227 = for {
                      shift-right: [w554] -> w552
                      shift-left: w551 -> [w555]
                      tunnel: string[] ["Z STEPPER CAM HEIGHT", "READ STEPPER VALUES"] ("element") -> [w553] mode=indexing
                      n228 = Enqueue Element(queue=w555, element=w553) -> (queue out=w554:refnum<queue>)  [unwired: 2 in, 2 out]
                    }
                  }
                  frame True {
                    n229 = for {
                      shift-right: [w560] -> w558
                      shift-left: w557 -> [w561]
                      tunnel: string[] ["ARDUINO - ULTRASONIC", "READ ULTRASONIC", "", "", "", ""] -> [w559] mode=indexing
                      n230 = Enqueue Element(queue=w561, element=w559) -> (queue out=w560:refnum<queue>)  [unwired: 2 in, 2 out]
                    }
                  }
                }
                n231 = Select(t=State_Type_Definitions."True Stop" ("Enum"), s=w540, f=State_Type_Definitions."Task 2:Sensor Mode" ("Enum")) -> (s? t:f=w543:T10)
                n232 = Select(t=w543, s=w541, f=State_Type_Definitions."Task 2:Raise Arm" ("Enum")) -> (s? t:f=w549:T10)
              }
              frame "Exit" {
                n233 = for {
                  shift-right: [w567] -> w564
                  shift-left: _ -> [w568]
                  tunnel: string[] ["STOP", "RESET ENCODERS", "RESET YAW", ""] -> [w566] mode=indexing
                  n234 = Enqueue Element(queue=w568, element=w566) -> (queue out=w567:refnum<queue>)  [unwired: 2 in, 2 out]
                }
              }
            }
          }
          frame 9 {
            w585 = u8 20 ("y")
            # ">>> yStepper command>>>"
            # ">>Object detected>>"
            n235 = Dequeue Element(queue=w577, timeout in ms (-1)=w576, error in (no error)=w575) -> (element=w586:T1)  [unwired: 3 out]
            n236 = Less?(x=w573, y=w585) -> (x < y?=w584:bool)
            n237 = Less?(x=w572, y=w585) -> (x < y?=w583:bool)
            n238 = Or(x=w584, y=w583) -> (x .or. y?=w582:bool)
            "Obstacle detected" <- w582
            n239 = case shown="\"Start Task 1\", Default" w586 {
              tunnel: w582 -> [w589 _]
              tunnel: [w596 State_Type_Definitions."True Stop" ("Enum")] -> w581
              tunnel: w574 -> [w588 _]
              tunnel: w578 -> [w595 w612]
              tunnel: [w594 w613] -> w580
              tunnel: [State_Type_Definitions."Idle" ("Enum") State_Type_Definitions."Shutdown" ("Enum")] -> w579
              frame "Start Task 1", Default {
                n240 = case shown="True" w589 {
                  tunnel: w595 -> [w599 w606]
                  tunnel: [w600 w605] -> w594
                  frame False {
                    n241 = for {
                      tunnel: string[] ["READ ULTRASONIC", "STOP"] ("element") -> [w601] mode=indexing
                      shift-right: [w603] -> w600
                      shift-left: w599 -> [w602]
                      n242 = Enqueue Element(queue=w602, element=w601) -> (queue out=w603:refnum<queue>)  [unwired: 2 in, 2 out]
                    }
                  }
                  frame True {
                    n243 = for {
                      shift-right: [w608] -> w605
                      shift-left: w606 -> [w609]
                      tunnel: string[] ["RESET ENCODERS", "READ NAVX", "READ ENCODERS"] -> [w607] mode=indexing
                      n244 = Enqueue Element(queue=w609, element=w607) -> (queue out=w608:refnum<queue>)  [unwired: 2 in, 2 out]
                    }
                  }
                }
                n245 = Or(x=w589, y=w588) -> (x .or. y?=w587:bool)
                n246 = Select(t=State_Type_Definitions."True Stop" ("Enum"), s=w588, f=State_Type_Definitions."Task 2:Reverse Mode" ("Enum")) -> (s? t:f=w590:T10)
                n247 = Select(t=w590, s=w587, f=State_Type_Definitions."Task 2:Sensor Mode" ("Enum")) -> (s? t:f=w596:T10)
              }
              frame "Exit" {
                n248 = for {
                  shift-right: [w616] -> w613
                  shift-left: w612 -> [w617]
                  tunnel: string[] ["STOP", "RESET ENCODERS", "RESET YAW", "ARDUINO MODE 0"] -> [w615] mode=indexing
                  n249 = Enqueue Element(queue=w617, element=w615) -> (queue out=w616:refnum<queue>)  [unwired: 2 in, 2 out]
                }
              }
            }
          }
          frame 10 {
            # ">>> yStepper command>>>"
            n250 = Dequeue Element(queue=w628, timeout in ms (-1)=w629, error in (no error)=w630) -> (element=w632:T1)  [unwired: 3 out]
            n251 = Less?(x=w622, y=-50.0) -> (x < y?=w620:bool)
            n252 = case shown="\"Start Task 1\", Default" w632 {
              tunnel: [w642 State_Type_Definitions."True Stop" ("Enum")] -> w624
              tunnel: w631 -> [w635 _]
              tunnel: w627 -> [w641 w658]
              tunnel: [w640 w659] -> w623
              tunnel: [State_Type_Definitions."Idle" ("Enum") State_Type_Definitions."Shutdown" ("Enum")] -> w625
              tunnel: w620 -> [w633 _]
              frame "Start Task 1", Default {
                n253 = case shown="False" w633 {
                  tunnel: w641 -> [w645 w652]
                  tunnel: [w646 w651] -> w640
                  frame False {
                    n254 = for {
                      tunnel: string[] ["READ ENCODERS", "REVERSE", "READ NAVX"] ("element") -> [w647] mode=indexing
                      shift-right: [w649] -> w646
                      shift-left: w645 -> [w648]
                      n255 = Enqueue Element(queue=w648, element=w647) -> (queue out=w649:refnum<queue>)  [unwired: 2 in, 2 out]
                    }
                  }
                  frame True {
                    n256 = for {
                      shift-right: [w654] -> w651
                      shift-left: w652 -> [w655]
                      tunnel: string[] ["STOP", "ARDUINO - ULTRASONIC", "READ ULTRASONIC", "RESET ENCODERS"] -> [w653] mode=indexing
                      n257 = Enqueue Element(queue=w655, element=w653) -> (queue out=w654:refnum<queue>)  [unwired: 2 in, 2 out]
                    }
                  }
                }
                n258 = Or(x=w633, y=w635) -> (x .or. y?=w634:bool)
                n259 = Select(t=State_Type_Definitions."True Stop" ("Enum"), s=w635, f=State_Type_Definitions."Task 2:Sensor Mode" ("Enum")) -> (s? t:f=w636:T10)
                n260 = Select(t=w636, s=w634, f=State_Type_Definitions."Task 2:Reverse Mode" ("Enum")) -> (s? t:f=w642:T10)
              }
              frame "Exit" {
                n261 = for {
                  shift-right: [w662] -> w659
                  shift-left: w658 -> [w663]
                  tunnel: string[] ["STOP", "RESET ENCODERS", "RESET YAW", "ARDUINO MODE 0"] -> [w661] mode=indexing
                  n262 = Enqueue Element(queue=w663, element=w661) -> (queue out=w662:refnum<queue>)  [unwired: 2 in, 2 out]
                }
              }
            }
          }
          frame 11 {
            # ">>> yStepper command>>>"
            n263 = Dequeue Element(queue=w679, timeout in ms (-1)=w678, error in (no error)=w677) -> (element=w668:T1)  [unwired: 3 out]
            n264 = Greater?(x=w676, y=160.0) -> (0:w673:bool)
            n265 = Or(x=w673, y=w674) -> (x .or. y?=w669:bool)
            n266 = case shown="\"Start Task 1\", Default" w668 {
              tunnel: w669 -> [w682 _]
              tunnel: [w686 State_Type_Definitions."True Stop" ("Enum")] -> w670
              tunnel: w672 -> [w683 w702]
              tunnel: [w681 w701] -> w671
              tunnel: [State_Type_Definitions."Idle" ("Enum") State_Type_Definitions."Shutdown" ("Enum")] -> w667
              frame "Start Task 1", Default {
                n267 = case shown="False" w682 {
                  tunnel: w683 -> [w689 w695]
                  tunnel: [w688 w693] -> w681
                  frame False {
                    n268 = for {
                      shift-right: [w691] -> w688
                      shift-left: w689 -> [w692]
                      tunnel: string[] ["READ ENCODERS", "R-CW"] ("element") -> [w690] mode=indexing
                      n269 = Enqueue Element(queue=w692, element=w690) -> (queue out=w691:refnum<queue>)  [unwired: 2 in, 2 out]
                    }
                  }
                  frame True {
                    n270 = for {
                      shift-right: [w697] -> w693
                      shift-left: w695 -> [w698]
                      tunnel: string[] ["RESET YAW", "RESET ENCODERS", "STOP", "ARDUINO MODE 0"] -> [w696] mode=indexing
                      n271 = Enqueue Element(queue=w698, element=w696) -> (queue out=w697:refnum<queue>)  [unwired: 2 in, 2 out]
                    }
                  }
                }
                n272 = Select(t=State_Type_Definitions."True Stop" ("Enum"), s=w682, f=State_Type_Definitions."Task 3" ("Enum")) -> (s? t:f=w686:T10)
              }
              frame "Exit" {
                n273 = for {
                  shift-right: [w705] -> w701
                  shift-left: w702 -> [w706]
                  tunnel: string[] ["STOP", "RESET ENCODERS", "RESET YAW", ""] -> [w704] mode=indexing
                  n274 = Enqueue Element(queue=w706, element=w704) -> (queue out=w705:refnum<queue>)  [unwired: 2 in, 2 out]
                }
              }
            }
          }
          frame 12 {
            # ">> Stepper height reeached >>"
            # ">>> yStepper command>>>"
            # ">> Manual override >>"
            n275 = Dequeue Element(queue=w720, timeout in ms (-1)=w719, error in (no error)=w718) -> (element=w717:T1)  [unwired: 3 out]
            n276 = Equal?(x=w711, y=u8 60) -> (x = y?=w709:bool)
            n277 = case shown="\"Exit\"" w717 {
              tunnel: [w732 State_Type_Definitions."True Stop" ("Enum")] -> w716
              tunnel: [w730 w748] -> w715
              tunnel: w721 -> [w729 w745]
              tunnel: w714 -> [w723 _]
              tunnel: [State_Type_Definitions."Idle" ("Enum") State_Type_Definitions."Shutdown" ("Enum")] -> w713
              tunnel: w709 -> [w722 _]
              frame "Start Task 1", Default {
                # ">> WIill proceed to part ii if not manual override >>"
                # ">>If ENABLE or Trigger is set to true>>"
                n278 = Or(x=w722, y=w723) -> (x .or. y?=w724:bool)
                n279 = case shown="False" w722 {
                  tunnel: [w735 w741] -> w730
                  tunnel: w729 -> [w734 w740]
                  frame False {
                    n280 = for {
                      shift-right: [w737] -> w735
                      shift-left: w734 -> [w738]
                      tunnel: string[] ["Z STEPPER CAM HEIGHT", "READ STEPPER VALUES"] ("element") -> [w736] mode=indexing
                      n281 = Enqueue Element(queue=w738, element=w736) -> (queue out=w737:refnum<queue>)  [unwired: 2 in, 2 out]
                    }
                  }
                  frame True {
                    n282 = for {
                      shift-right: [w743] -> w741
                      shift-left: w740 -> [w744]
                      tunnel: string[] ["ARDUINO - ULTRASONIC", "READ ULTRASONIC", "FORWARD", "", "", ""] -> [w742] mode=indexing
                      n283 = Enqueue Element(queue=w744, element=w742) -> (queue out=w743:refnum<queue>)  [unwired: 2 in, 2 out]
                    }
                  }
                }
                n284 = Select(t=State_Type_Definitions."True Stop" ("Enum"), s=w723, f=State_Type_Definitions."Task 4_B" ("Enum")) -> (s? t:f=w726:T10)
                n285 = Select(t=w726, s=w724, f=State_Type_Definitions."Task 4_A" ("Enum")) -> (s? t:f=w732:T10)
              }
              frame "Exit" {
                n286 = for {
                  shift-right: [w751] -> w748
                  shift-left: w745 -> [w752]
                  tunnel: string[] ["STOP", "RESET ENCODERS", "RESET YAW", ""] -> [w750] mode=indexing
                  n287 = Enqueue Element(queue=w752, element=w750) -> (queue out=w751:refnum<queue>)  [unwired: 2 in, 2 out]
                }
              }
            }
          }
          frame 13 {
            w758 = u8 20
            # ">> Path blocked >>"
            # ">>> yStepper command>>>"
            # ">> Manual override >>"
            n288 = Dequeue Element(queue=w767, timeout in ms (-1)=w766, error in (no error)=w765) -> (element=w764:T1)  [unwired: 3 out]
            n289 = Less?(x=w760, y=w758) -> (x < y?=w755:bool)
            n290 = Less?(x=w759, y=w758) -> (x < y?=w756:bool)
            n291 = And(x=w756, y=w755) -> (x .and. y?=w757:bool)
            n292 = case shown="\"Start Task 1\", Default" w764 {
              tunnel: [w781 State_Type_Definitions."True Stop" ("Enum")] -> w769
              tunnel: [w779 w796] -> w770
              tunnel: w763 -> [w778 _]
              tunnel: w768 -> [w772 _]
              tunnel: [State_Type_Definitions."Idle" ("Enum") State_Type_Definitions."Shutdown" ("Enum")] -> w762
              tunnel: w757 -> [w771 _]
              frame "Start Task 1", Default {
                # ">> Manual override forces program to true stop >>"
                # ">>If ENABLE or Trigger is set to true>>"
                n293 = Or(x=w771, y=w772) -> (x .or. y?=w777:bool)
                n294 = case shown="True" w771 {
                  tunnel: [w784 w789] -> w779
                  tunnel: w778 -> [w783 w788]
                  frame False {
                    n295 = for {
                      shift-right: [w786] -> w784
                      shift-left: w783 -> [w787]
                      tunnel: string[] ["FORWARD", "READ ULTRASONIC", "READ NAVX"] ("element") -> [w785] mode=indexing
                      n296 = Enqueue Element(queue=w787, element=w785) -> (queue out=w786:refnum<queue>)  [unwired: 2 in, 2 out]
                    }
                  }
                  frame True {
                    n297 = for {
                      shift-right: [w792] -> w789
                      shift-left: w788 -> [w793]
                      tunnel: string[] ["STOP", "RESET YAW", "RESET ENCODERS", "RESET FLAGS"] -> [w791] mode=indexing
                      n298 = Enqueue Element(queue=w793, element=w791) -> (queue out=w792:refnum<queue>)  [unwired: 2 in, 2 out]
                    }
                  }
                }
                n299 = Select(t=State_Type_Definitions."True Stop" ("Enum"), s=w772, f=State_Type_Definitions."Task 4_C" ("Enum")) -> (s? t:f=w774:T10)
                n300 = Select(t=w774, s=w777, f=State_Type_Definitions."Task 4_B" ("Enum")) -> (s? t:f=w781:T10)
              }
              frame "Exit" {
                n301 = for {
                  shift-right: [w799] -> w796
                  shift-left: _ -> [w800]
                  tunnel: string[] ["STOP", "RESET ENCODERS", "RESET YAW", ""] -> [w798] mode=indexing
                  n302 = Enqueue Element(queue=w800, element=w798) -> (queue out=w799:refnum<queue>)  [unwired: 2 in, 2 out]
                }
              }
            }
          }
          frame 14 {
            w812 = u8 20
            # ">> xDistance travelled>>"
            # ">> Path NOT blocked >>"
            # ">>> yStepper command>>>"
            # ">> Manual override >>"
            n303 = Dequeue Element(queue=w822, timeout in ms (-1)=w815, error in (no error)=w814) -> (element=w816:T1)  [unwired: 3 out]
            n304 = Greater?(x=w804, y=w812) -> (0:w810:bool)
            n305 = Greater?(x=w809, y=80.0) -> (0:w807:bool)
            n306 = Greater?(x=w803, y=w812) -> (0:w811:bool)
            n307 = And(x=w811, y=w810) -> (x .and. y?=w806:bool)
            n308 = And(x=w807, y=w806) -> (x .and. y?=w805:bool)
            n309 = case shown="\"Exit\"" w816 {
              tunnel: [w833 State_Type_Definitions."True Stop" ("Enum")] -> w819
              tunnel: [w831 w849] -> w818
              tunnel: w821 -> [w830 w846]
              tunnel: w820 -> [w824 _]
              tunnel: [State_Type_Definitions."Idle" ("t") State_Type_Definitions."Shutdown" ("Enum")] -> w817
              tunnel: w805 -> [w823 _]
              frame "Start Task 1", Default {
                # ">> Manual override forces program to true stop >>"
                # ">>If ENABLE or Trigger is set to true>>"
                n310 = Or(x=w823, y=w824) -> (x .or. y?=w829:bool)
                n311 = case shown="False" w823 {
                  tunnel: [w836 w841] -> w831
                  tunnel: w830 -> [w834 w840]
                  frame False {
                    n312 = for {
                      shift-right: [w838] -> w836
                      shift-left: w834 -> [w839]
                      tunnel: string[] ["RIGHT", "READ NAVX", "READ ENCODERS", "READ ULTRASONIC"] ("element") -> [w837] mode=indexing
                      n313 = Enqueue Element(queue=w839, element=w837) -> (queue out=w838:refnum<queue>)  [unwired: 2 in, 2 out]
                    }
                  }
                  frame True {
                    n314 = for {
                      shift-right: [w844] -> w841
                      shift-left: w840 -> [w845]
                      tunnel: string[] ["STOP", "RESET YAW", "RESET ENCODERS", "ARDUINO - ULTRASONIC"] -> [w843] mode=indexing
                      n315 = Enqueue Element(queue=w845, element=w843) -> (queue out=w844:refnum<queue>)  [unwired: 2 in, 2 out]
                    }
                  }
                }
                n316 = Select(t=State_Type_Definitions."True Stop" ("Enum"), s=w824, f=State_Type_Definitions."Task 4_D" ("Enum")) -> (s? t:f=w825:T10)
                n317 = Select(t=w825, s=w829, f=State_Type_Definitions."Task 4_C" ("Enum")) -> (s? t:f=w833:T10)
              }
              frame "Exit" {
                n318 = for {
                  shift-right: [w852] -> w849
                  shift-left: w846 -> [w853]
                  tunnel: string[] ["STOP", "RESET ENCODERS", "RESET YAW", ""] -> [w851] mode=indexing
                  n319 = Enqueue Element(queue=w853, element=w851) -> (queue out=w852:refnum<queue>)  [unwired: 2 in, 2 out]
                }
              }
            }
          }
          frame 15 {
            w874 = u8 20
            # ">> yDistance travelled>>"
            # ">> Path blocked >>"
            # ">>> yStepper command>>>"
            # ">> Manual override >>"
            n320 = Dequeue Element(queue=w865, timeout in ms (-1)=w864, error in (no error)=w863) -> (element=w875:T1)  [unwired: 3 out]
            n321 = Less?(x=w858, y=w874) -> (x < y?=w872:bool)
            n322 = Greater?(x=w862, y=200.0) -> (0:w870:bool)
            n323 = Less?(x=w857, y=w874) -> (x < y?=w873:bool)
            n324 = And(x=w873, y=w872) -> (x .and. y?=w869:bool)
            n325 = Or(x=w870, y=w869) -> (x .or. y?=w868:bool)
            n326 = case shown="\"Start Task 1\", Default" w875 {
              tunnel: [w886 State_Type_Definitions."True Stop" ("Enum")] -> w861
              tunnel: [w884 w902] -> w859
              tunnel: w866 -> [w883 w899]
              tunnel: w867 -> [w877 _]
              tunnel: [State_Type_Definitions."Idle" ("t") State_Type_Definitions."Shutdown" ("Enum")] -> w860
              tunnel: w868 -> [w876 _]
              frame "Start Task 1", Default {
                # ">> Manual override forces program to true stop >>"
                # ">>If ENABLE or Trigger is set to true>>"
                n327 = Or(x=w876, y=w877) -> (x .or. y?=w882:bool)
                n328 = case shown="True" w876 {
                  tunnel: [w889 w894] -> w884
                  tunnel: w883 -> [w887 w893]
                  frame False {
                    n329 = for {
                      shift-right: [w891] -> w889
                      shift-left: w887 -> [w892]
                      tunnel: string[] ["FORWARD", "READ NAVX", "READ ENCODERS", "READ ULTRASONIC"] ("element") -> [w890] mode=indexing
                      n330 = Enqueue Element(queue=w892, element=w890) -> (queue out=w891:refnum<queue>)  [unwired: 2 in, 2 out]
                    }
                  }
                  frame True {
                    n331 = for {
                      shift-right: [w897] -> w894
                      shift-left: w893 -> [w898]
                      tunnel: string[] ["STOP", "RESET YAW", "RESET ENCODERS", "RESET FLAGS"] -> [w896] mode=indexing
                      n332 = Enqueue Element(queue=w898, element=w896) -> (queue out=w897:refnum<queue>)  [unwired: 2 in, 2 out]
                    }
                  }
                }
                n333 = Select(t=State_Type_Definitions."True Stop" ("Enum"), s=w877, f=State_Type_Definitions."True Stop" ("Enum")) -> (s? t:f=w878:T10)
                n334 = Select(t=w878, s=w882, f=State_Type_Definitions."Task 4_D" ("Enum")) -> (s? t:f=w886:T10)
              }
              frame "Exit" {
                n335 = for {
                  shift-right: [w905] -> w902
                  shift-left: w899 -> [w906]
                  tunnel: string[] ["STOP", "RESET ENCODERS", "RESET YAW", ""] -> [w904] mode=indexing
                  n336 = Enqueue Element(queue=w906, element=w904) -> (queue out=w905:refnum<queue>)  [unwired: 2 in, 2 out]
                }
              }
            }
          }
          frame 15 {
            # ">>> yStepper command>>>"
            # ">> Manual override >>"
            n337 = Dequeue Element(queue=w917, timeout in ms (-1)=w916, error in (no error)=w918) -> (element=w915:T1)  [unwired: 3 out]
            n338 = Equal?(x=w914, y=u8 60) -> (x = y?=w912:bool)
            n339 = case shown="\"Start Task 1\", Default" w915 {
              tunnel: [w928 State_Type_Definitions."True Stop" ("Enum")] -> w919
              tunnel: [w931 w948] -> w920
              tunnel: [State_Type_Definitions."Idle" ("Enum") State_Type_Definitions."Shutdown" ("Enum")] -> w921
              tunnel: w912 -> [w927 _]
              tunnel: w911 -> [w926 _]
              tunnel: w910 -> [w922 w945]
              frame "Start Task 1", Default {
                # "Stays in Task 5_A until stepper reaches desired \nheight"
                # "T: Go back to idle, F: Continue with task\""
                # ">> Manual override >>"
                n340 = case shown="True" w927 {
                  tunnel: [w935 w941] -> w931
                  tunnel: w922 -> [w933 w939]
                  frame False {
                    n341 = for {
                      tunnel: string[] ["Z STEPPER CAM HEIGHT", "READ STEPPER VALUES"] ("element") -> [w936] mode=indexing
                      shift-right: [w938] -> w935
                      shift-left: w933 -> [w937]
                      n342 = Enqueue Element(queue=w937, element=w936) -> (queue out=w938:refnum<queue>)  [unwired: 2 in, 2 out]
                    }
                  }
                  frame True {
                    n343 = for {
                      shift-right: [w943] -> w941
                      shift-left: w939 -> [w944]
                      tunnel: string[] ["ARDUINO - ULTRASONIC", "READ ULTRASONIC", ""] -> [w942] mode=indexing
                      n344 = Enqueue Element(queue=w944, element=w942) -> (queue out=w943:refnum<queue>)  [unwired: 2 in, 2 out]
                    }
                  }
                }
                n345 = Or(x=w927, y=w926) -> (x .or. y?=w929:bool)
                n346 = Select(t=State_Type_Definitions."True Stop" ("Enum"), s=w926, f=State_Type_Definitions."Task 5B: MOVE TO BOX" ("Enum")) -> (s? t:f=w923:u16)
                n347 = Select(t=w923, s=w929, f=State_Type_Definitions."Task 5A: ARM CAM HEIGHT" ("Enum")) -> (s? t:f=w928:u16)
              }
              frame "Exit" {
                n348 = for {
                  shift-right: [w951] -> w948
                  shift-left: w945 -> [w952]
                  tunnel: string[] ["STOP", "RESET ENCODERS", "RESET YAW", "ARDUINO MODE 0"] -> [w950] mode=indexing
                  n349 = Enqueue Element(queue=w952, element=w950) -> (queue out=w951:refnum<queue>)  [unwired: 2 in, 2 out]
                }
              }
            }
          }
          frame 16 {
            w960 = u8 20 ("y")
            # ">>> yStepper command>>>"
            n350 = Less?(x=w957, y=w960) -> (x < y?=w958:bool)
            n351 = Dequeue Element(queue=w964, timeout in ms (-1)=w963, error in (no error)=w965) -> (element=w962:T1)  [unwired: 3 out]
            n352 = Less?(x=w956, y=w960) -> (x < y?=w959:bool)
            n353 = And(x=w959, y=w958) -> (x .and. y?=w955:bool)
            n354 = case shown="\"Start Task 1\", Default" w962 {
              tunnel: [w977 State_Type_Definitions."True Stop" ("Enum")] -> w967
              tunnel: [w980 w997] -> w966
              tunnel: [State_Type_Definitions."Idle" ("Enum") State_Type_Definitions."Shutdown" ("Enum")] -> w968
              tunnel: w970 -> [w976 _]
              tunnel: w969 -> [w972 w994]
              tunnel: w955 -> [w971 _]
              frame "Start Task 1", Default {
                # "Stays in Task 5_B to capture image over 5 seconds"
                # "T: Go back to idle, F: Continue with task\""
                # ">> Manual override >>"
                n355 = case shown="True" w971 {
                  tunnel: [w984 w990] -> w980
                  tunnel: w972 -> [w982 w988]
                  frame False {
                    n356 = for {
                      tunnel: string[] ["FORWARD", "READ ULTRASONIC", "READ NAVX"] ("element") -> [w985] mode=indexing
                      shift-right: [w987] -> w984
                      shift-left: w982 -> [w986]
                      n357 = Enqueue Element(queue=w986, element=w985) -> (queue out=w987:refnum<queue>)  [unwired: 2 in, 2 out]
                    }
                  }
                  frame True {
                    n358 = for {
                      shift-right: [w992] -> w990
                      shift-left: w988 -> [w993]
                      tunnel: string[] ["STOP", "RESET ENCODERS", "OPEN LOG CAM", "SET TIMER 5"] -> [w991] mode=indexing
                      n359 = Enqueue Element(queue=w993, element=w991) -> (queue out=w992:refnum<queue>)  [unwired: 2 in, 2 out]
                    }
                  }
                }
                n360 = Or(x=w971, y=w976) -> (x .or. y?=w978:bool)
                n361 = Select(t=State_Type_Definitions."True Stop" ("Enum"), s=w976, f=State_Type_Definitions."Task 5C: CAM BURST" ("Enum")) -> (s? t:f=w973:u16)
                n362 = Select(t=w973, s=w978, f=State_Type_Definitions."Task 5B: MOVE TO BOX" ("Enum")) -> (s? t:f=w977:u16)
              }
              frame "Exit" {
                n363 = for {
                  shift-right: [w1000] -> w997
                  shift-left: w994 -> [w1001]
                  tunnel: string[] ["STOP", "RESET ENCODERS", "RESET YAW", "ARDUINO MODE 0"] -> [w999] mode=indexing
                  n364 = Enqueue Element(queue=w1001, element=w999) -> (queue out=w1000:refnum<queue>)  [unwired: 2 in, 2 out]
                }
              }
            }
          }
          frame 17 {
            # ">>> Motor control cluster >>>"
            # ">>> yStepper command>>>"
            # ">> Manual override >>"
            n365 = Dequeue Element(queue=w1012, timeout in ms (-1)=w1011, error in (no error)=w1010) -> (element=w1009:T1)  [unwired: 3 out]
            n366 = case shown="\"Start Task 1\", Default" w1009 {
              tunnel: [w1021 State_Type_Definitions."True Stop" ("Enum")] -> w1014
              tunnel: [w1024 w1041] -> w1007
              tunnel: [State_Type_Definitions."Idle" ("Enum") State_Type_Definitions."Shutdown" ("Enum")] -> w1006
              tunnel: w1008 -> [w1015 _]
              tunnel: w1013 -> [w1020 w1038]
              tunnel: w1004 -> [w1019 _]
              frame "Start Task 1", Default {
                # ">> Is time up? >>"
                # "Determines if object is in range to pick up"
                # ">> Manual override >>"
                n367 = case shown="False" w1019 {
                  tunnel: [w1028 w1034] -> w1024
                  tunnel: w1020 -> [w1026 w1032]
                  frame False {
                    n368 = for {
                      tunnel: string[] ["CAM ACQ", "START TIMER"] ("element") -> [w1029] mode=indexing
                      shift-right: [w1031] -> w1028
                      shift-left: w1026 -> [w1030]
                      n369 = Enqueue Element(queue=w1030, element=w1029) -> (queue out=w1031:refnum<queue>)  [unwired: 2 in, 2 out]
                    }
                  }
                  frame True {
                    n370 = for {
                      shift-right: [w1036] -> w1034
                      shift-left: w1032 -> [w1037]
                      tunnel: string[] ["CAM CLOSE", "PROCESS IMAGE", "SET TIMER 5"] -> [w1035] mode=indexing
                      n371 = Enqueue Element(queue=w1037, element=w1035) -> (queue out=w1036:refnum<queue>)  [unwired: 2 in, 2 out]
                    }
                  }
                }
                n372 = Or(x=w1019, y=w1015) -> (x .or. y?=w1022:bool)
                n373 = Select(t=State_Type_Definitions."True Stop" ("Enum"), s=w1015, f=State_Type_Definitions."Task 5D: PROCESS IMAGE" ("Enum")) -> (s? t:f=w1017:u16)
                n374 = Select(t=w1017, s=w1022, f=State_Type_Definitions."Task 5C: CAM BURST" ("Enum")) -> (s? t:f=w1021:u16)
              }
              frame "Exit" {
                n375 = for {
                  shift-right: [w1044] -> w1041
                  shift-left: w1038 -> [w1045]
                  tunnel: string[] ["STOP", "RESET ENCODERS", "RESET YAW", "ARDUINO MODE 0"] -> [w1043] mode=indexing
                  n376 = Enqueue Element(queue=w1045, element=w1043) -> (queue out=w1044:refnum<queue>)  [unwired: 2 in, 2 out]
                }
              }
            }
          }
          frame 18 {
            # ">>> yStepper command>>>"
            n377 = Dequeue Element(queue=w1053, timeout in ms (-1)=w1052, error in (no error)=w1051) -> (element=w1050:T1)  [unwired: 3 out]
            n378 = case shown="\"Start Task 1\", Default" w1050 {
              tunnel: [w1065 State_Type_Definitions."True Stop" ("Enum")] -> w1057
              tunnel: [w1068 w1085] -> w1056
              tunnel: [State_Type_Definitions."Idle" ("Enum") State_Type_Definitions."Shutdown" ("Enum")] -> w1058
              tunnel: w1054 -> [w1064 _]
              tunnel: w1055 -> [w1060 w1082]
              tunnel: w1048 -> [w1059 _]
              frame "Start Task 1", Default {
                # ">> T: Breaks out of state loop; F: Stays in loop>>"
                # ">> Manual override >>"
                # ">> Checks if time is up>>"
                # "Stays in Task 5D until the object is detected"
                # "T: Go back to idle, F: Continue with task\""
                # ">> Manual override >>"
                n379 = case shown="True" w1059 {
                  tunnel: [w1072 w1078] -> w1068
                  tunnel: w1060 -> [w1070 w1076]
                  frame False {
                    n380 = for {
                      tunnel: string[] ["START TIMER", "PROCESS IMAGE", ""] ("element") -> [w1073] mode=indexing
                      shift-right: [w1075] -> w1072
                      shift-left: w1070 -> [w1074]
                      n381 = Enqueue Element(queue=w1074, element=w1073) -> (queue out=w1075:refnum<queue>)  [unwired: 2 in, 2 out]
                    }
                  }
                  frame True {
                    n382 = for {
                      shift-right: [w1080] -> w1078
                      shift-left: w1076 -> [w1081]
                      tunnel: string[] ["CAM CLOSE", "", ""] -> [w1079] mode=indexing
                      n383 = Enqueue Element(queue=w1081, element=w1079) -> (queue out=w1080:refnum<queue>)  [unwired: 2 in, 2 out]
                    }
                  }
                }
                n384 = Or(x=w1059, y=w1064) -> (x .or. y?=w1066:bool)
                n385 = Select(t=State_Type_Definitions."True Stop" ("Enum"), s=w1064, f=State_Type_Definitions."Task 5E: POSITION ARM" ("Enum")) -> (s? t:f=w1061:T10)
                n386 = Select(t=w1061, s=w1066, f=State_Type_Definitions."Task 5D: PROCESS IMAGE" ("Enum")) -> (s? t:f=w1065:u16)
              }
              frame "Exit" {
                n387 = for {
                  shift-right: [w1088] -> w1085
                  shift-left: w1082 -> [w1089]
                  tunnel: string[] ["STOP", "RESET ENCODERS", "RESET YAW", "ARDUINO MODE 0"] -> [w1087] mode=indexing
                  n388 = Enqueue Element(queue=w1089, element=w1087) -> (queue out=w1088:refnum<queue>)  [unwired: 2 in, 2 out]
                }
              }
            }
          }
          frame 20 {
            # ">>> yStepper command>>>"
            n389 = Dequeue Element(queue=w1103, timeout in ms (-1)=w1104, error in (no error)=w1105) -> (element=w1107:T1)  [unwired: 3 out]
            n390 = formula code="if (pos < 100)\ny = 41;\n\nelse if (pos >= 100 && pos <= 140)\ny = 30;\n\nelse if (pos >= 141 && pos <= 170)\ny = 25;\n\nelse if (pos >= 171 &&pos <= 180) \ny = 20;\n\nelse if (pos >= 181&& pos <= 200)\ny = 15;\n\nelse if (pos >= 201 && pos <= 230)\ny = 10;\n\nelse if (pos >= 231 && pos <= 320)\ny = 8;\n\nelse if (pos > 320)\ny = 0;"("pos"=w1095) -> ("y"=w1098:dbl)
            n391 = To Unsigned Byte Integer(number=w1098) -> (unsigned 8bit integer=w1093:u8)
            n392 = Equal?(x=w1094, y=w1093) -> (x = y?=w1092:bool)
            n393 = case shown="\"Start Task 1\", Default" w1107 {
              tunnel: [w1114 State_Type_Definitions."True Stop" ("Enum")] -> w1101
              tunnel: [w1117 w1134] -> w1099
              tunnel: [State_Type_Definitions."Idle" ("Enum") State_Type_Definitions."Shutdown" ("Enum")] -> w1100
              tunnel: w1106 -> [w1113 _]
              tunnel: w1102 -> [w1109 w1131]
              tunnel: w1092 -> [w1108 _]
              frame "Start Task 1", Default {
                # ">> T: Breaks out of state loop; F: Stays in loop>>"
                # ">> Manual override >>"
                # ">> Checks if time is up>>"
                # "Stays in Task 5D until the object is detected"
                # "T: Go back to idle, F: Continue with task\""
                # ">> Manual override >>"
                n394 = case shown="False" w1108 {
                  tunnel: [w1121 w1127] -> w1117
                  tunnel: w1109 -> [w1119 w1125]
                  frame False {
                    n395 = for {
                      tunnel: string[] ["READ STEPPER VALUES", "Y STEPPER CONTROL", ""] ("element") -> [w1122] mode=indexing
                      shift-right: [w1124] -> w1121
                      shift-left: w1119 -> [w1123]
                      n396 = Enqueue Element(queue=w1123, element=w1122) -> (queue out=w1124:refnum<queue>)  [unwired: 2 in, 2 out]
                    }
                  }
                  frame True {
                    n397 = for {
                      shift-right: [w1129] -> w1127
                      shift-left: w1125 -> [w1130]
                      tunnel: string[] ["CAM CLOSE", "DISPOSE BUFFERS", ""] -> [w1128] mode=indexing
                      n398 = Enqueue Element(queue=w1130, element=w1128) -> (queue out=w1129:refnum<queue>)  [unwired: 2 in, 2 out]
                    }
                  }
                }
                n399 = Or(x=w1108, y=w1113) -> (x .or. y?=w1115:bool)
                n400 = Select(t=State_Type_Definitions."True Stop" ("Enum"), s=w1113, f=State_Type_Definitions."Task 5F: ARM GRAB HEIGHT" ("Enum")) -> (s? t:f=w1110:T10)
                n401 = Select(t=w1110, s=w1115, f=State_Type_Definitions."Task 5E: POSITION ARM" ("Enum")) -> (s? t:f=w1114:T10)
              }
              frame "Exit" {
                n402 = for {
                  shift-right: [w1137] -> w1134
                  shift-left: w1131 -> [w1138]
                  tunnel: string[] ["STOP", "RESET ENCODERS", "RESET YAW", "ARDUINO MODE 0"] -> [w1136] mode=indexing
                  n403 = Enqueue Element(queue=w1138, element=w1136) -> (queue out=w1137:refnum<queue>)  [unwired: 2 in, 2 out]
                }
              }
            }
            n404 = Bundle By Name(cluster=w1097, "yStepper desired"=w1093) -> (w1096:T14)
          }
          frame 21 {
            # ">>> Motor control cluster >>>"
            # ">>> yStepper command>>>"
            # ">> Manual override >>"
            n405 = Dequeue Element(queue=w1149, timeout in ms (-1)=w1148, error in (no error)=w1150) -> (element=w1147:T1)  [unwired: 3 out]
            n406 = Equal?(x=w1146, y=u8 1) -> (x = y?=w1144:bool)
            n407 = case shown="\"Start Task 1\", Default" w1147 {
              tunnel: [w1160 State_Type_Definitions."True Stop" ("Enum")] -> w1151
              tunnel: [w1163 w1180] -> w1152
              tunnel: [State_Type_Definitions."Idle" ("Enum") State_Type_Definitions."Shutdown" ("Enum")] -> w1153
              tunnel: w1144 -> [w1159 _]
              tunnel: w1143 -> [w1158 _]
              tunnel: w1142 -> [w1154 w1177]
              frame "Start Task 1", Default {
                # "Stays in Task 5F until stepper reaches desired \nheight"
                # "T: Go back to idle, F: Continue with task\""
                # ">> Manual override >>"
                n408 = case shown="True" w1159 {
                  tunnel: [w1167 w1173] -> w1163
                  tunnel: w1154 -> [w1165 w1171]
                  frame False {
                    n409 = for {
                      tunnel: string[] ["Z STEPPER GRAB HEIGHT", "READ STEPPER VALUES"] ("element") -> [w1168] mode=indexing
                      shift-right: [w1170] -> w1167
                      shift-left: w1165 -> [w1169]
                      n410 = Enqueue Element(queue=w1169, element=w1168) -> (queue out=w1170:refnum<queue>)  [unwired: 2 in, 2 out]
                    }
                  }
                  frame True {
                    n411 = for {
                      shift-right: [w1175] -> w1173
                      shift-left: w1171 -> [w1176]
                      tunnel: string[] ["SET TIMER 5", "CLOSE CLAW", ""] -> [w1174] mode=indexing
                      n412 = Enqueue Element(queue=w1176, element=w1174) -> (queue out=w1175:refnum<queue>)  [unwired: 2 in, 2 out]
                    }
                  }
                }
                n413 = Or(x=w1159, y=w1158) -> (x .or. y?=w1161:bool)
                n414 = Select(t=State_Type_Definitions."True Stop" ("Enum"), s=w1158, f=State_Type_Definitions."Task 5G: CLOSE CLAW" ("Enum")) -> (s? t:f=w1155:T10)
                n415 = Select(t=w1155, s=w1161, f=State_Type_Definitions."Task 5F: ARM GRAB HEIGHT" ("Enum")) -> (s? t:f=w1160:T10)
              }
              frame "Exit" {
                n416 = for {
                  shift-right: [w1183] -> w1180
                  shift-left: w1177 -> [w1184]
                  tunnel: string[] ["STOP", "RESET ENCODERS", "RESET YAW", "ARDUINO MODE 0"] -> [w1182] mode=indexing
                  n417 = Enqueue Element(queue=w1184, element=w1182) -> (queue out=w1183:refnum<queue>)  [unwired: 2 in, 2 out]
                }
              }
            }
          }
          frame 22 {
            # ">>> yStepper command>>>"
            # ">> Manual override >>"
            n418 = Dequeue Element(queue=w1195, timeout in ms (-1)=w1194, error in (no error)=w1193) -> (element=w1192:T1)  [unwired: 3 out]
            n419 = case shown="\"Start Task 1\", Default" w1192 {
              tunnel: [w1204 State_Type_Definitions."True Stop" ("Enum")] -> w1197
              tunnel: [w1207 w1224] -> w1190
              tunnel: [State_Type_Definitions."Idle" ("Enum") State_Type_Definitions."Shutdown" ("Enum")] -> w1189
              tunnel: w1191 -> [w1198 _]
              tunnel: w1196 -> [w1203 w1221]
              tunnel: w1187 -> [w1202 _]
              frame "Start Task 1", Default {
                # ">> Is time up? >>"
                # "Determines if object is in range to pick up"
                # ">> Manual override >>"
                n420 = case shown="True" w1202 {
                  tunnel: [w1211 w1217] -> w1207
                  tunnel: w1203 -> [w1209 w1215]
                  frame False {
                    n421 = for {
                      tunnel: string[] ["CLOSE CLAW", "START TIMER"] ("element") -> [w1212] mode=indexing
                      shift-right: [w1214] -> w1211
                      shift-left: w1209 -> [w1213]
                      n422 = Enqueue Element(queue=w1213, element=w1212) -> (queue out=w1214:refnum<queue>)  [unwired: 2 in, 2 out]
                    }
                  }
                  frame True {
                    n423 = for {
                      shift-right: [w1219] -> w1217
                      shift-left: w1215 -> [w1220]
                      tunnel: string[] ["READ STEPPER VALUES", "", ""] -> [w1218] mode=indexing
                      n424 = Enqueue Element(queue=w1220, element=w1218) -> (queue out=w1219:refnum<queue>)  [unwired: 2 in, 2 out]
                    }
                  }
                }
                n425 = Or(x=w1202, y=w1198) -> (x .or. y?=w1205:bool)
                n426 = Select(t=State_Type_Definitions."True Stop" ("Enum"), s=w1198, f=State_Type_Definitions."Task 5H: RAISE ARM" ("Enum")) -> (s? t:f=w1200:T10)
                n427 = Select(t=w1200, s=w1205, f=State_Type_Definitions."Task 5G: CLOSE CLAW" ("Enum")) -> (s? t:f=w1204:T10)
              }
              frame "Exit" {
                n428 = for {
                  shift-right: [w1227] -> w1224
                  shift-left: w1221 -> [w1228]
                  tunnel: string[] ["STOP", "RESET ENCODERS", "RESET YAW", "ARDUINO MODE 0"] -> [w1226] mode=indexing
                  n429 = Enqueue Element(queue=w1228, element=w1226) -> (queue out=w1227:refnum<queue>)  [unwired: 2 in, 2 out]
                }
              }
            }
          }
          frame 23 {
            # ">>> yStepper command>>>"
            # ">> Manual override >>"
            n430 = Dequeue Element(queue=w1239, timeout in ms (-1)=w1238, error in (no error)=w1240) -> (element=w1237:T1)  [unwired: 3 out]
            n431 = Equal?(x=w1236, y=u8 60) -> (x = y?=w1234:bool)
            n432 = case shown="\"Start Task 1\", Default" w1237 {
              tunnel: [w1250 State_Type_Definitions."True Stop" ("Enum")] -> w1241
              tunnel: [w1253 w1270] -> w1242
              tunnel: [State_Type_Definitions."Idle" ("Enum") State_Type_Definitions."Shutdown" ("Enum")] -> w1243
              tunnel: w1234 -> [w1249 _]
              tunnel: w1233 -> [w1248 _]
              tunnel: w1232 -> [w1244 w1267]
              frame "Start Task 1", Default {
                # "Stays in Task 5_A until stepper reaches desired \nheight"
                # "T: Go back to idle, F: Continue with task\""
                # ">> Manual override >>"
                n433 = case shown="False" w1249 {
                  tunnel: [w1257 w1263] -> w1253
                  tunnel: w1244 -> [w1255 w1261]
                  frame False {
                    n434 = for {
                      tunnel: string[] ["Z STEPPER CAM HEIGHT", "READ STEPPER VALUES"] ("element") -> [w1258] mode=indexing
                      shift-right: [w1260] -> w1257
                      shift-left: w1255 -> [w1259]
                      n435 = Enqueue Element(queue=w1259, element=w1258) -> (queue out=w1260:refnum<queue>)  [unwired: 2 in, 2 out]
                    }
                  }
                  frame True {
                    n436 = for {
                      shift-right: [w1265] -> w1263
                      shift-left: w1261 -> [w1266]
                      tunnel: string[] ["ARDUINO - ULTRASONIC", "READ ULTRASONIC", ""] -> [w1264] mode=indexing
                      n437 = Enqueue Element(queue=w1266, element=w1264) -> (queue out=w1265:refnum<queue>)  [unwired: 2 in, 2 out]
                    }
                  }
                }
                n438 = Or(x=w1249, y=w1248) -> (x .or. y?=w1251:bool)
                n439 = Select(t=State_Type_Definitions."True Stop" ("Enum"), s=w1248, f=State_Type_Definitions."True Stop" ("Enum")) -> (s? t:f=w1245:T10)
                n440 = Select(t=w1245, s=w1251, f=State_Type_Definitions."Task 5H: RAISE ARM" ("Enum")) -> (s? t:f=w1250:T10)
              }
              frame "Exit" {
                n441 = for {
                  shift-right: [w1273] -> w1270
                  shift-left: w1267 -> [w1274]
                  tunnel: string[] ["STOP", "RESET ENCODERS", "RESET YAW", "ARDUINO MODE 0"] -> [w1272] mode=indexing
                  n442 = Enqueue Element(queue=w1274, element=w1272) -> (queue out=w1273:refnum<queue>)  [unwired: 2 in, 2 out]
                }
              }
            }
          }
          frame 24 {
            # ">>> yStepper command>>>"
            n443 = Dequeue Element(queue=w1284, timeout in ms (-1)=w1283, error in (no error)=w1282) -> (element=w1289:T1)  [unwired: 3 out]
            n444 = Equal?(x=w1280, y=u8 60) -> (x = y?=w1279:bool)
            n445 = case shown="\"Start Task 1\", Default" w1289 {
              tunnel: [w1296 State_Type_Definitions."True Stop" ("Enum")] -> w1287
              tunnel: [w1295 w1313] -> w1286
              tunnel: [State_Type_Definitions."Idle" ("Enum") State_Type_Definitions."Shutdown" ("Enum")] -> w1288
              tunnel: w1285 -> [w1291 _]
              tunnel: w1281 -> [w1293 _]
              tunnel: w1279 -> [w1290 _]
              frame "Start Task 1", Default {
                n446 = case shown="False" w1290 {
                  tunnel: [w1301 w1307] -> w1295
                  tunnel: w1293 -> [w1299 w1305]
                  frame False {
                    n447 = for {
                      tunnel: string[] ["Z STEPPER CAM HEIGHT", "READ STEPPER VALUES"] ("element") -> [w1302] mode=indexing
                      shift-right: [w1304] -> w1301
                      shift-left: w1299 -> [w1303]
                      n448 = Enqueue Element(queue=w1303, element=w1302) -> (queue out=w1304:refnum<queue>)  [unwired: 2 in, 2 out]
                    }
                  }
                  frame True {
                    n449 = for {
                      shift-right: [w1309] -> w1307
                      shift-left: w1305 -> [w1310]
                      tunnel: string[] ["CAM ACQ", "OPEN LOG CAM"] -> [w1308] mode=indexing
                      n450 = Enqueue Element(queue=w1310, element=w1308) -> (queue out=w1309:refnum<queue>)  [unwired: 2 in, 2 out]
                    }
                  }
                }
                n451 = Or(x=w1290, y=w1291) -> (x .or. y?=w1292:bool)
                n452 = Select(t=State_Type_Definitions."Task 6_B" ("Enum"), s=w1292, f=State_Type_Definitions."Task 6_A" ("Enum")) -> (s? t:f=w1296:T10)
              }
              frame "Exit" {
                n453 = for {
                  shift-right: [w1316] -> w1313
                  shift-left: _ -> [w1317]
                  tunnel: string[] ["STOP", "RESET ENCODERS", "RESET YAW", "ARDUINO MODE 0"] -> [w1315] mode=indexing
                  n454 = Enqueue Element(queue=w1317, element=w1315) -> (queue out=w1316:refnum<queue>)  [unwired: 2 in, 2 out]
                }
              }
            }
          }
          frame 25 {
            # ">>> yStepper command>>>"
            n455 = Dequeue Element(queue=w1329, timeout in ms (-1)=w1327, error in (no error)=w1328) -> (element=w1326:T1)  [unwired: 3 out]
            n456 = case shown="\"Start Task 1\", Default" w1326 {
              tunnel: [w1336 State_Type_Definitions."True Stop" ("Enum")] -> w1322
              tunnel: [w1335 w1354] -> w1330
              tunnel: [State_Type_Definitions."Idle" ("Enum") State_Type_Definitions."Shutdown" ("Enum")] -> w1323
              tunnel: w1325 -> [w1331 _]
              tunnel: w1324 -> [w1333 _]
              tunnel: w1321 -> [w1332 w1351]
              frame "Start Task 1", Default {
                # ">> Manual override >>"
                n457 = case shown="True" w1333 {
                  tunnel: [w1341 w1347] -> w1335
                  tunnel: w1332 -> [w1340 w1345]
                  frame False {
                    n458 = for {
                      shift-right: [w1344] -> w1341
                      shift-left: w1340 -> [w1343]
                      tunnel: string[] ["CAM ACQ", "PROCESS IMAGE", "OPEN CLAW"] -> [w1342] mode=indexing
                      n459 = Enqueue Element(queue=w1343, element=w1342) -> (queue out=w1344:refnum<queue>)  [unwired: 2 in, 2 out]
                    }
                  }
                  frame True {
                    n460 = for {
                      shift-right: [w1349] -> w1347
                      shift-left: w1345 -> [w1350]
                      tunnel: string[] ["CAM ACQ", "PROCESS IMAGE", "CLOSE CLAW"] -> [w1348] mode=indexing
                      n461 = Enqueue Element(queue=w1350, element=w1348) -> (queue out=w1349:refnum<queue>)  [unwired: 2 in, 2 out]
                    }
                  }
                }
                n462 = Select(t=State_Type_Definitions."True Stop" ("Enum"), s=w1331, f=State_Type_Definitions."Task 6_B" ("Enum")) -> (s? t:f=w1336:T10)
              }
              frame "Exit" {
                # ">> State after true stop >>"
                # ">> Goes to true stop >>"
                n463 = for {
                  shift-right: [w1357] -> w1354
                  shift-left: w1351 -> [w1358]
                  tunnel: string[] ["STOP", "RESET ENCODERS", "RESET YAW", ""] -> [w1356] mode=indexing
                  n464 = Enqueue Element(queue=w1358, element=w1356) -> (queue out=w1357:refnum<queue>)  [unwired: 2 in, 2 out]
                }
              }
            }
          }
          frame 26 {
          }
          frame 27 {
            # ">>> Motor control cluster >>>"
            # ">>> yStepper command>>>"
            # ">> Manual override >>"
            n465 = Dequeue Element(queue=w1375, timeout in ms (-1)=w1374, error in (no error)=w1376) -> (element=w1373:T1)  [unwired: 3 out]
            n466 = Equal?(x=w1372, y=u8 60) -> (x = y?=w1370:bool)
            n467 = case shown="\"Start Task 1\", Default" w1373 {
              tunnel: [w1386 State_Type_Definitions."True Stop" ("Enum")] -> w1377
              tunnel: [w1389 w1406] -> w1378
              tunnel: [State_Type_Definitions."Idle" ("Enum") State_Type_Definitions."Shutdown" ("Enum")] -> w1379
              tunnel: w1370 -> [w1385 _]
              tunnel: w1369 -> [w1384 _]
              tunnel: w1368 -> [w1380 w1403]
              frame "Start Task 1", Default {
                # "Stays in Task 5_A until stepper reaches desired \nheight"
                # "T: Go back to idle, F: Continue with task\""
                # ">> Manual override >>"
                n468 = case shown="False" w1385 {
                  tunnel: [w1393 w1399] -> w1389
                  tunnel: w1380 -> [w1391 w1397]
                  frame False {
                    n469 = for {
                      tunnel: string[] ["Z STEPPER CAM HEIGHT", "READ STEPPER VALUES"] ("element") -> [w1394] mode=indexing
                      shift-right: [w1396] -> w1393
                      shift-left: w1391 -> [w1395]
                      n470 = Enqueue Element(queue=w1395, element=w1394) -> (queue out=w1396:refnum<queue>)  [unwired: 2 in, 2 out]
                    }
                  }
                  frame True {
                    n471 = for {
                      shift-right: [w1401] -> w1399
                      shift-left: w1397 -> [w1402]
                      tunnel: string[] ["ARDUINO - ULTRASONIC", "READ ULTRASONIC", ""] -> [w1400] mode=indexing
                      n472 = Enqueue Element(queue=w1402, element=w1400) -> (queue out=w1401:refnum<queue>)  [unwired: 2 in, 2 out]
                    }
                  }
                }
                n473 = Or(x=w1385, y=w1384) -> (x .or. y?=w1387:bool)
                n474 = Select(t=State_Type_Definitions."True Stop" ("Enum"), s=w1384, f=State_Type_Definitions."Task 8B: MOVE TO BOX" ("Enum")) -> (s? t:f=w1381:T10)
                n475 = Select(t=w1381, s=w1387, f=State_Type_Definitions."Task 8A: RAISE ARM" ("Enum")) -> (s? t:f=w1386:T10)
              }
              frame "Exit" {
                n476 = for {
                  shift-right: [w1409] -> w1406
                  shift-left: w1403 -> [w1410]
                  tunnel: string[] ["STOP", "RESET ENCODERS", "RESET YAW", "ARDUINO MODE 0"] -> [w1408] mode=indexing
                  n477 = Enqueue Element(queue=w1410, element=w1408) -> (queue out=w1409:refnum<queue>)  [unwired: 2 in, 2 out]
                }
              }
            }
          }
          frame 28 {
            w1418 = u8 15 ("y")
            # ">>> yStepper command>>>"
            n478 = Less?(x=w1415, y=w1418) -> (x < y?=w1416:bool)
            n479 = Dequeue Element(queue=w1422, timeout in ms (-1)=w1421, error in (no error)=w1423) -> (element=w1420:T1)  [unwired: 3 out]
            n480 = Less?(x=w1414, y=w1418) -> (x < y?=w1417:bool)
            n481 = And(x=w1417, y=w1416) -> (x .and. y?=w1413:bool)
            n482 = case shown="\"Start Task 1\", Default" w1420 {
              tunnel: [w1435 State_Type_Definitions."True Stop" ("Enum")] -> w1425
              tunnel: [w1438 w1455] -> w1424
              tunnel: [State_Type_Definitions."Idle" ("Enum") State_Type_Definitions."Shutdown" ("Enum")] -> w1426
              tunnel: w1428 -> [w1434 _]
              tunnel: w1427 -> [w1430 w1452]
              tunnel: w1413 -> [w1429 _]
              frame "Start Task 1", Default {
                # "Stays in Task 5_B to capture image over 5 seconds"
                # "T: Go back to idle, F: Continue with task\""
                # ">> Manual override >>"
                n483 = case shown="True" w1429 {
                  tunnel: [w1442 w1448] -> w1438
                  tunnel: w1430 -> [w1440 w1446]
                  frame False {
                    n484 = for {
                      tunnel: string[] ["FORWARD", "READ ULTRASONIC", "READ NAVX"] ("element") -> [w1443] mode=indexing
                      shift-right: [w1445] -> w1442
                      shift-left: w1440 -> [w1444]
                      n485 = Enqueue Element(queue=w1444, element=w1443) -> (queue out=w1445:refnum<queue>)  [unwired: 2 in, 2 out]
                    }
                  }
                  frame True {
                    n486 = for {
                      shift-right: [w1450] -> w1448
                      shift-left: w1446 -> [w1451]
                      tunnel: string[] ["STOP", "RESET ENCODERS", "OPEN LOG CAM", "SET TIMER 2", "OPEN IMAQ REF"] -> [w1449] mode=indexing
                      n487 = Enqueue Element(queue=w1451, element=w1449) -> (queue out=w1450:refnum<queue>)  [unwired: 2 in, 2 out]
                    }
                  }
                }
                n488 = Or(x=w1429, y=w1434) -> (x .or. y?=w1436:bool)
                n489 = Select(t=State_Type_Definitions."True Stop" ("Enum"), s=w1434, f=State_Type_Definitions."Task 8C: CAM BURST" ("Enum")) -> (s? t:f=w1431:T10)
                n490 = Select(t=w1431, s=w1436, f=State_Type_Definitions."Task 8B: MOVE TO BOX" ("Enum")) -> (s? t:f=w1435:T10)
              }
              frame "Exit" {
                n491 = for {
                  shift-right: [w1458] -> w1455
                  shift-left: w1452 -> [w1459]
                  tunnel: string[] ["STOP", "RESET ENCODERS", "RESET YAW", "ARDUINO MODE 0"] -> [w1457] mode=indexing
                  n492 = Enqueue Element(queue=w1459, element=w1457) -> (queue out=w1458:refnum<queue>)  [unwired: 2 in, 2 out]
                }
              }
            }
          }
          frame 29 {
            # ">>> Motor control cluster >>>"
            # ">>> yStepper command>>>"
            # ">> Manual override >>"
            n493 = Dequeue Element(queue=w1470, timeout in ms (-1)=w1469, error in (no error)=w1468) -> (element=w1467:T1)  [unwired: 3 out]
            n494 = case shown="\"Start Task 1\", Default" w1467 {
              tunnel: [w1479 State_Type_Definitions."True Stop" ("Enum")] -> w1472
              tunnel: [w1482 w1499] -> w1465
              tunnel: [State_Type_Definitions."Idle" ("Enum") State_Type_Definitions."Shutdown" ("Enum")] -> w1464
              tunnel: w1466 -> [w1473 _]
              tunnel: w1471 -> [w1478 w1496]
              tunnel: w1462 -> [w1477 _]
              frame "Start Task 1", Default {
                # ">> Is time up? >>"
                # "Determines if object is in range to pick up"
                # ">> Manual override >>"
                n495 = case shown="True" w1477 {
                  tunnel: [w1486 w1492] -> w1482
                  tunnel: w1478 -> [w1484 w1490]
                  frame False {
                    n496 = for {
                      tunnel: string[] ["CAM ACQ", "START TIMER"] ("element") -> [w1487] mode=indexing
                      shift-right: [w1489] -> w1486
                      shift-left: w1484 -> [w1488]
                      n497 = Enqueue Element(queue=w1488, element=w1487) -> (queue out=w1489:refnum<queue>)  [unwired: 2 in, 2 out]
                    }
                  }
                  frame True {
                    n498 = for {
                      shift-right: [w1494] -> w1492
                      shift-left: w1490 -> [w1495]
                      tunnel: string[] ["CAM CLOSE", "PROCESS IMAGE", "SET TIMER 5"] -> [w1493] mode=indexing
                      n499 = Enqueue Element(queue=w1495, element=w1493) -> (queue out=w1494:refnum<queue>)  [unwired: 2 in, 2 out]
                    }
                  }
                }
                n500 = Or(x=w1477, y=w1473) -> (x .or. y?=w1480:bool)
                n501 = Select(t=State_Type_Definitions."True Stop" ("Enum"), s=w1473, f=State_Type_Definitions."Task 8D: PROCESS IMAGE" ("Enum")) -> (s? t:f=w1475:T10)
                n502 = Select(t=w1475, s=w1480, f=State_Type_Definitions."Task 8C: CAM BURST" ("Enum")) -> (s? t:f=w1479:T10)
              }
              frame "Exit" {
                n503 = for {
                  shift-right: [w1502] -> w1499
                  shift-left: w1496 -> [w1503]
                  tunnel: string[] ["STOP", "RESET ENCODERS", "RESET YAW", "ARDUINO MODE 0"] -> [w1501] mode=indexing
                  n504 = Enqueue Element(queue=w1503, element=w1501) -> (queue out=w1502:refnum<queue>)  [unwired: 2 in, 2 out]
                }
              }
            }
          }
          frame 30 {
            # ">>> yStepper command>>>"
            n505 = Dequeue Element(queue=w1511, timeout in ms (-1)=w1510, error in (no error)=w1509) -> (element=w1508:T1)  [unwired: 3 out]
            n506 = case shown="\"Start Task 1\", Default" w1508 {
              tunnel: [w1523 State_Type_Definitions."True Stop" ("Enum")] -> w1515
              tunnel: [w1526 w1543] -> w1514
              tunnel: [State_Type_Definitions."Idle" ("Enum") State_Type_Definitions."Shutdown" ("Enum")] -> w1516
              tunnel: w1512 -> [w1522 _]
              tunnel: w1513 -> [w1518 w1540]
              tunnel: w1506 -> [w1517 _]
              frame "Start Task 1", Default {
                # ">> T: Breaks out of state loop; F: Stays in loop>>"
                # ">> Manual override >>"
                # ">> Checks if time is up>>"
                # "Stays in Task 5D until the object is detected"
                # "T: Go back to idle, F: Continue with task\""
                # ">> Manual override >>"
                n507 = case shown="True" w1517 {
                  tunnel: [w1530 w1536] -> w1526
                  tunnel: w1518 -> [w1528 w1534]
                  frame False {
                    n508 = for {
                      tunnel: string[] ["START TIMER", "PROCESS IMAGE", ""] ("element") -> [w1531] mode=indexing
                      shift-right: [w1533] -> w1530
                      shift-left: w1528 -> [w1532]
                      n509 = Enqueue Element(queue=w1532, element=w1531) -> (queue out=w1533:refnum<queue>)  [unwired: 2 in, 2 out]
                    }
                  }
                  frame True {
                    n510 = for {
                      shift-right: [w1538] -> w1536
                      shift-left: w1534 -> [w1539]
                      tunnel: string[] ["RESET ENCODERS", "", ""] -> [w1537] mode=indexing
                      n511 = Enqueue Element(queue=w1539, element=w1537) -> (queue out=w1538:refnum<queue>)  [unwired: 2 in, 2 out]
                    }
                  }
                }
                n512 = Or(x=w1517, y=w1522) -> (x .or. y?=w1524:bool)
                n513 = Select(t=State_Type_Definitions."True Stop" ("Enum"), s=w1522, f=State_Type_Definitions."Task 8E: ROBOT ADJUST" ("Enum")) -> (s? t:f=w1519:T10)
                n514 = Select(t=w1519, s=w1524, f=State_Type_Definitions."Task 8D: PROCESS IMAGE" ("Enum")) -> (s? t:f=w1523:T10)
              }
              frame "Exit" {
                n515 = for {
                  shift-right: [w1546] -> w1543
                  shift-left: w1540 -> [w1547]
                  tunnel: string[] ["STOP", "RESET ENCODERS", "RESET YAW", "ARDUINO MODE 0"] -> [w1545] mode=indexing
                  n516 = Enqueue Element(queue=w1547, element=w1545) -> (queue out=w1546:refnum<queue>)  [unwired: 2 in, 2 out]
                }
              }
            }
          }
          frame 31 {
            # ">>> Motor control cluster >>>"
            # ">>> yStepper command>>>"
            n517 = Dequeue Element(queue=w1564, timeout in ms (-1)=w1563, error in (no error)=w1562) -> (element=w1561:T1)  [unwired: 3 out]
            n518 = Subtract(x=w1559, y=300.0) -> (x-y=w1557:dbl)
            "x-y" <- w1557
            n519 = formula code="if (error <= -61&&error > -300){\ndistance = -15;\nxSpeed = -30;\n}\n\nelse if (error <= -51 && error >= -60){\ndistance = -10;\nxSpeed = -30;\n}\n\nelse if (error >= -50 && error <= 50){\ndistance = 0;\nxSpeed = 0;\n}\n\nelse if (error >= 51 && error <= 80){\ndistance = 10;\nxSpeed = 30;\n}\n\nelse if (error >= 81 && error <= 100){\ndistance = 15;\nxSpeed = 30;\n}\n\nelse if (error >= 101 && error <= 120){\ndistance = 20;\nxSpeed = 30;\n}\n\nelse if (error >= 121 && error < 300){\ndistance = 25;\nxSpeed = 30;\n}\n\nelse{\ndistance = 0;\nxSpeed = 0;\n}"("error"=w1557) -> ("distance"=w1552:dbl, "xSpeed"=w1554:dbl)
            n520 = formula code="if (target > 0){\nif (current  >= target)\noutput = 1;\n\nelse if (current != target)\noutput = 0;\n}\n\nelse if (target == 0){\nif (current == target)\noutput = 1;\n\nelse if (current != target)\noutput = 0;\n}\n\nelse if (target < 0){\nif (current <= target)\noutput = 1;\n\nelse if (current != target)\noutput = 0;\n}\n\nelse if (current != target)\noutput = 0;"("target"=w1552, "current"=w1553) -> ("output"=w1551:dbl)
            n521 = Bundle By Name(cluster=w1556, "xSpeed"=w1554) -> (w1555:T12)
            n522 = Equal?(x=w1551, y=1.0) -> (x = y?=w1549:bool)
            n523 = case shown="\"Start Task 1\", Default" w1561 {
              tunnel: [w1576 State_Type_Definitions."True Stop" ("Enum")] -> w1568
              tunnel: [w1579 w1596] -> w1567
              tunnel: [State_Type_Definitions."Idle" ("Enum") State_Type_Definitions."Shutdown" ("Enum")] -> w1569
              tunnel: w1565 -> [w1575 _]
              tunnel: w1566 -> [w1571 w1593]
              tunnel: w1549 -> [w1570 _]
              frame "Start Task 1", Default {
                # ">> T: Breaks out of state loop; F: Stays in loop>>"
                # ">> Manual override >>"
                # ">> Checks if time is up>>"
                # "Stays in Task 5D until the object is detected"
                # "T: Go back to idle, F: Continue with task\""
                # ">> Manual override >>"
                n524 = case shown="True" w1570 {
                  tunnel: [w1583 w1589] -> w1579
                  tunnel: w1571 -> [w1581 w1587]
                  frame False {
                    n525 = for {
                      tunnel: string[] ["X AXIS - SLOW", "READ ENCODERS", "READ NAVX"] ("element") -> [w1584] mode=indexing
                      shift-right: [w1586] -> w1583
                      shift-left: w1581 -> [w1585]
                      n526 = Enqueue Element(queue=w1585, element=w1584) -> (queue out=w1586:refnum<queue>)  [unwired: 2 in, 2 out]
                    }
                  }
                  frame True {
                    n527 = for {
                      shift-right: [w1591] -> w1589
                      shift-left: w1587 -> [w1592]
                      tunnel: string[] ["SET TIMER 2", "STOP", "READ STEPPER VALUES", ""] -> [w1590] mode=indexing
                      n528 = Enqueue Element(queue=w1592, element=w1590) -> (queue out=w1591:refnum<queue>)  [unwired: 2 in, 2 out]
                    }
                  }
                }
                n529 = Or(x=w1570, y=w1575) -> (x .or. y?=w1577:bool)
                n530 = Select(t=State_Type_Definitions."True Stop" ("Enum"), s=w1575, f=State_Type_Definitions."Task 8H: ARM ADJUST" ("Enum")) -> (s? t:f=w1572:T10)
                n531 = Select(t=w1572, s=w1577, f=State_Type_Definitions."Task 8E: ROBOT ADJUST" ("Enum")) -> (s? t:f=w1576:T10)
              }
              frame "Exit" {
                n532 = for {
                  shift-right: [w1599] -> w1596
                  shift-left: w1593 -> [w1600]
                  tunnel: string[] ["STOP", "RESET ENCODERS", "RESET YAW", "ARDUINO MODE 0"] -> [w1598] mode=indexing
                  n533 = Enqueue Element(queue=w1600, element=w1598) -> (queue out=w1599:refnum<queue>)  [unwired: 2 in, 2 out]
                }
              }
            }
          }
          frame 32 {
            # ">>> Motor control cluster >>>"
            # ">>> yStepper command>>>"
            # ">> Manual override >>"
            n534 = Dequeue Element(queue=w1611, timeout in ms (-1)=w1610, error in (no error)=w1609) -> (element=w1608:T1)  [unwired: 3 out]
            n535 = case shown="\"Start Task 1\", Default" w1608 {
              tunnel: [w1620 State_Type_Definitions."True Stop" ("Enum")] -> w1613
              tunnel: [w1623 w1640] -> w1606
              tunnel: [State_Type_Definitions."Idle" ("Enum") State_Type_Definitions."Shutdown" ("Enum")] -> w1605
              tunnel: w1607 -> [w1614 _]
              tunnel: w1612 -> [w1619 w1637]
              tunnel: w1603 -> [w1618 _]
              frame "Start Task 1", Default {
                # ">> Is time up? >>"
                # "Determines if object is in range to pick up"
                # ">> Manual override >>"
                n536 = case shown="True" w1618 {
                  tunnel: [w1627 w1633] -> w1623
                  tunnel: w1619 -> [w1625 w1631]
                  frame False {
                    n537 = for {
                      tunnel: string[] ["CAM ACQ", "START TIMER"] ("element") -> [w1628] mode=indexing
                      shift-right: [w1630] -> w1627
                      shift-left: w1625 -> [w1629]
                      n538 = Enqueue Element(queue=w1629, element=w1628) -> (queue out=w1630:refnum<queue>)  [unwired: 2 in, 2 out]
                    }
                  }
                  frame True {
                    n539 = for {
                      shift-right: [w1635] -> w1633
                      shift-left: w1631 -> [w1636]
                      tunnel: string[] ["CAM CLOSE", "PROCESS IMAGE", "SET TIMER 3"] -> [w1634] mode=indexing
                      n540 = Enqueue Element(queue=w1636, element=w1634) -> (queue out=w1635:refnum<queue>)  [unwired: 2 in, 2 out]
                    }
                  }
                }
                n541 = Or(x=w1618, y=w1614) -> (x .or. y?=w1621:bool)
                n542 = Select(t=State_Type_Definitions."True Stop" ("Enum"), s=w1614, f=State_Type_Definitions."Task 8G: PROCESS IMAGE 2" ("Enum")) -> (s? t:f=w1616:T10)
                n543 = Select(t=w1616, s=w1621, f=State_Type_Definitions."Task 8F: CAM BURST 2" ("Enum")) -> (s? t:f=w1620:T10)
              }
              frame "Exit" {
                n544 = for {
                  shift-right: [w1643] -> w1640
                  shift-left: w1637 -> [w1644]
                  tunnel: string[] ["STOP", "RESET ENCODERS", "RESET YAW", "ARDUINO MODE 0"] -> [w1642] mode=indexing
                  n545 = Enqueue Element(queue=w1644, element=w1642) -> (queue out=w1643:refnum<queue>)  [unwired: 2 in, 2 out]
                }
              }
            }
          }
          frame 33 {
            # ">>> yStepper command>>>"
            n546 = Dequeue Element(queue=w1652, timeout in ms (-1)=w1651, error in (no error)=w1650) -> (element=w1649:T1)  [unwired: 3 out]
            n547 = case shown="\"Start Task 1\", Default" w1649 {
              tunnel: [w1664 State_Type_Definitions."True Stop" ("Enum")] -> w1656
              tunnel: [w1667 w1684] -> w1655
              tunnel: [State_Type_Definitions."Idle" ("Enum") State_Type_Definitions."Shutdown" ("Enum")] -> w1657
              tunnel: w1653 -> [w1663 _]
              tunnel: w1654 -> [w1659 w1681]
              tunnel: w1647 -> [w1658 _]
              frame "Start Task 1", Default {
                # ">> T: Breaks out of state loop; F: Stays in loop>>"
                # ">> Manual override >>"
                # ">> Checks if time is up>>"
                # "Stays in Task 5D until the object is detected"
                # "T: Go back to idle, F: Continue with task\""
                # ">> Manual override >>"
                n548 = case shown="False" w1658 {
                  tunnel: [w1671 w1677] -> w1667
                  tunnel: w1659 -> [w1669 w1675]
                  frame False {
                    n549 = for {
                      tunnel: string[] ["START TIMER", "PROCESS IMAGE", ""] ("element") -> [w1672] mode=indexing
                      shift-right: [w1674] -> w1671
                      shift-left: w1669 -> [w1673]
                      n550 = Enqueue Element(queue=w1673, element=w1672) -> (queue out=w1674:refnum<queue>)  [unwired: 2 in, 2 out]
                    }
                  }
                  frame True {
                    n551 = for {
                      shift-right: [w1679] -> w1677
                      shift-left: w1675 -> [w1680]
                      tunnel: string[] ["READ STEPPER VALUES", "Y STEPPER CONTROL", ""] -> [w1678] mode=indexing
                      n552 = Enqueue Element(queue=w1680, element=w1678) -> (queue out=w1679:refnum<queue>)  [unwired: 2 in, 2 out]
                    }
                  }
                }
                n553 = Or(x=w1658, y=w1663) -> (x .or. y?=w1665:bool)
                n554 = Select(t=State_Type_Definitions."True Stop" ("Enum"), s=w1663, f=State_Type_Definitions."Task 8H: ARM ADJUST" ("Enum")) -> (s? t:f=w1660:T10)
                n555 = Select(t=w1660, s=w1665, f=State_Type_Definitions."Task 8G: PROCESS IMAGE 2" ("Enum")) -> (s? t:f=w1664:T10)
              }
              frame "Exit" {
                n556 = for {
                  shift-right: [w1687] -> w1684
                  shift-left: w1681 -> [w1688]
                  tunnel: string[] ["STOP", "RESET ENCODERS", "RESET YAW", "ARDUINO MODE 0"] -> [w1686] mode=indexing
                  n557 = Enqueue Element(queue=w1688, element=w1686) -> (queue out=w1687:refnum<queue>)  [unwired: 2 in, 2 out]
                }
              }
            }
          }
          frame 34 {
            # ">>> yStepper command>>>"
            n558 = Dequeue Element(queue=w1702, timeout in ms (-1)=w1703, error in (no error)=w1704) -> (element=w1706:T1)  [unwired: 3 out]
            n559 = formula code="if (pos < 70)\ny = 43;\n\nelse if (pos >= 71 &&pos <= 80)\ny = 40;\n\nelse if (pos >= 81 && pos <= 90)\ny = 38;\n\nelse if (pos >= 91 &&pos <= 120)\ny = 35;\n\nelse if (pos >= 121 && pos <= 140)\ny = 30;\n\nelse if (pos >= 141 && pos <= 170)\ny = 26;\n\nelse if (pos >= 171 &&pos <= 220) \ny = 20;\n\nelse if (pos >= 221&& pos <= 240)\ny = 15;\n\nelse if (pos >= 241 && pos <= 250)\ny = 10;\n\nelse if (pos >= 251)\ny = 0;"("pos"=w1694) -> ("y"=w1697:dbl)
            n560 = To Unsigned Byte Integer(number=w1697) -> (unsigned 8bit integer=w1692:u8)
            "Correcte stepper" <- w1692
            n561 = Equal?(x=w1693, y=w1692) -> (x = y?=w1691:bool)
            n562 = case shown="\"Start Task 1\", Default" w1706 {
              tunnel: [w1713 State_Type_Definitions."True Stop" ("Enum")] -> w1700
              tunnel: [w1716 w1733] -> w1698
              tunnel: [State_Type_Definitions."Idle" ("Enum") State_Type_Definitions."Shutdown" ("Enum")] -> w1699
              tunnel: w1705 -> [w1712 _]
              tunnel: w1701 -> [w1708 w1730]
              tunnel: w1691 -> [w1707 _]
              frame "Start Task 1", Default {
                # ">> T: Breaks out of state loop; F: Stays in loop>>"
                # ">> Manual override >>"
                # ">> Checks if time is up>>"
                # "Stays in Task 5D until the object is detected"
                # "T: Go back to idle, F: Continue with task\""
                # ">> Manual override >>"
                n563 = case shown="False" w1707 {
                  tunnel: [w1720 w1726] -> w1716
                  tunnel: w1708 -> [w1718 w1724]
                  frame False {
                    n564 = for {
                      tunnel: string[] ["READ STEPPER VALUES", "Y STEPPER CONTROL", ""] ("element") -> [w1721] mode=indexing
                      shift-right: [w1723] -> w1720
                      shift-left: w1718 -> [w1722]
                      n565 = Enqueue Element(queue=w1722, element=w1721) -> (queue out=w1723:refnum<queue>)  [unwired: 2 in, 2 out]
                    }
                  }
                  frame True {
                    n566 = for {
                      shift-right: [w1728] -> w1726
                      shift-left: w1724 -> [w1729]
                      tunnel: string[] ["DISPOSE BUFFERS", "READ STEPPER VALUES", ""] -> [w1727] mode=indexing
                      n567 = Enqueue Element(queue=w1729, element=w1727) -> (queue out=w1728:refnum<queue>)  [unwired: 2 in, 2 out]
                    }
                  }
                }
                n568 = Or(x=w1707, y=w1712) -> (x .or. y?=w1714:bool)
                n569 = Select(t=State_Type_Definitions."True Stop" ("Enum"), s=w1712, f=State_Type_Definitions."Task 8I: ARM GRAB HEIGHT" ("Enum")) -> (s? t:f=w1709:T10)
                n570 = Select(t=w1709, s=w1714, f=State_Type_Definitions."Task 8H: ARM ADJUST" ("Enum")) -> (s? t:f=w1713:T10)
              }
              frame "Exit" {
                n571 = for {
                  shift-right: [w1736] -> w1733
                  shift-left: w1730 -> [w1737]
                  tunnel: string[] ["STOP", "RESET ENCODERS", "RESET YAW", "ARDUINO MODE 0"] -> [w1735] mode=indexing
                  n572 = Enqueue Element(queue=w1737, element=w1735) -> (queue out=w1736:refnum<queue>)  [unwired: 2 in, 2 out]
                }
              }
            }
            n573 = Bundle By Name(cluster=w1696, "yStepper desired"=w1692) -> (w1695:T14)
          }
          frame 35 {
            # ">>> Motor control cluster >>>"
            # ">>> yStepper command>>>"
            # ">> Manual override >>"
            n574 = Dequeue Element(queue=w1748, timeout in ms (-1)=w1747, error in (no error)=w1749) -> (element=w1746:T1)  [unwired: 3 out]
            n575 = Equal?(x=w1745, y=u8 1) -> (x = y?=w1743:bool)
            n576 = case shown="\"Start Task 1\", Default" w1746 {
              tunnel: [w1759 State_Type_Definitions."True Stop" ("Enum")] -> w1750
              tunnel: [w1762 w1779] -> w1751
              tunnel: [State_Type_Definitions."Idle" ("Enum") State_Type_Definitions."Shutdown" ("Enum")] -> w1752
              tunnel: w1743 -> [w1758 _]
              tunnel: w1742 -> [w1757 _]
              tunnel: w1741 -> [w1753 w1776]
              frame "Start Task 1", Default {
                # "Stays in Task 5F until stepper reaches desired \nheight"
                # "T: Go back to idle, F: Continue with task\""
                # ">> Manual override >>"
                n577 = case shown="True" w1758 {
                  tunnel: [w1766 w1772] -> w1762
                  tunnel: w1753 -> [w1764 w1770]
                  frame False {
                    n578 = for {
                      tunnel: string[] ["Z STEPPER GRAB HEIGHT", "READ STEPPER VALUES"] ("element") -> [w1767] mode=indexing
                      shift-right: [w1769] -> w1766
                      shift-left: w1764 -> [w1768]
                      n579 = Enqueue Element(queue=w1768, element=w1767) -> (queue out=w1769:refnum<queue>)  [unwired: 2 in, 2 out]
                    }
                  }
                  frame True {
                    n580 = for {
                      shift-right: [w1774] -> w1772
                      shift-left: w1770 -> [w1775]
                      tunnel: string[] ["SET TIMER 2", "CLOSE CLAW", ""] -> [w1773] mode=indexing
                      n581 = Enqueue Element(queue=w1775, element=w1773) -> (queue out=w1774:refnum<queue>)  [unwired: 2 in, 2 out]
                    }
                  }
                }
                n582 = Or(x=w1758, y=w1757) -> (x .or. y?=w1760:bool)
                n583 = Select(t=State_Type_Definitions."True Stop" ("Enum"), s=w1757, f=State_Type_Definitions."Task 8J: CLOSE CLAW" ("Enum")) -> (s? t:f=w1754:T10)
                n584 = Select(t=w1754, s=w1760, f=State_Type_Definitions."Task 8I: ARM GRAB HEIGHT" ("Enum")) -> (s? t:f=w1759:T10)
              }
              frame "Exit" {
                n585 = for {
                  shift-right: [w1782] -> w1779
                  shift-left: w1776 -> [w1783]
                  tunnel: string[] ["STOP", "RESET ENCODERS", "RESET YAW", "ARDUINO MODE 0"] -> [w1781] mode=indexing
                  n586 = Enqueue Element(queue=w1783, element=w1781) -> (queue out=w1782:refnum<queue>)  [unwired: 2 in, 2 out]
                }
              }
            }
          }
          frame 36 {
            # ">>> yStepper command>>>"
            # ">> Manual override >>"
            n587 = Dequeue Element(queue=w1794, timeout in ms (-1)=w1793, error in (no error)=w1792) -> (element=w1791:T1)  [unwired: 3 out]
            n588 = case shown="\"Start Task 1\", Default" w1791 {
              tunnel: [w1803 State_Type_Definitions."True Stop" ("Enum")] -> w1796
              tunnel: [w1806 w1823] -> w1789
              tunnel: [State_Type_Definitions."Idle" ("Enum") State_Type_Definitions."Shutdown" ("Enum")] -> w1788
              tunnel: w1790 -> [w1797 _]
              tunnel: w1795 -> [w1802 w1820]
              tunnel: w1786 -> [w1801 _]
              frame "Start Task 1", Default {
                # ">> Is time up? >>"
                # "Determines if object is in range to pick up"
                # ">> Manual override >>"
                n589 = case shown="True" w1801 {
                  tunnel: [w1810 w1816] -> w1806
                  tunnel: w1802 -> [w1808 w1814]
                  frame False {
                    n590 = for {
                      tunnel: string[] ["CLOSE CLAW", "START TIMER"] ("element") -> [w1811] mode=indexing
                      shift-right: [w1813] -> w1810
                      shift-left: w1808 -> [w1812]
                      n591 = Enqueue Element(queue=w1812, element=w1811) -> (queue out=w1813:refnum<queue>)  [unwired: 2 in, 2 out]
                    }
                  }
                  frame True {
                    n592 = for {
                      shift-right: [w1818] -> w1816
                      shift-left: w1814 -> [w1819]
                      tunnel: string[] ["READ STEPPER VALUES", "", ""] -> [w1817] mode=indexing
                      n593 = Enqueue Element(queue=w1819, element=w1817) -> (queue out=w1818:refnum<queue>)  [unwired: 2 in, 2 out]
                    }
                  }
                }
                n594 = Or(x=w1801, y=w1797) -> (x .or. y?=w1804:bool)
                n595 = Select(t=State_Type_Definitions."True Stop" ("Enum"), s=w1797, f=State_Type_Definitions."Task 8K: RAISE MY SWORD" ("Enum")) -> (s? t:f=w1799:T10)
                n596 = Select(t=w1799, s=w1804, f=State_Type_Definitions."Task 8J: CLOSE CLAW" ("Enum")) -> (s? t:f=w1803:T10)
              }
              frame "Exit" {
                n597 = for {
                  shift-right: [w1826] -> w1823
                  shift-left: w1820 -> [w1827]
                  tunnel: string[] ["STOP", "RESET ENCODERS", "RESET YAW", "ARDUINO MODE 0"] -> [w1825] mode=indexing
                  n598 = Enqueue Element(queue=w1827, element=w1825) -> (queue out=w1826:refnum<queue>)  [unwired: 2 in, 2 out]
                }
              }
            }
          }
          frame 37 {
            # ">>> yStepper command>>>"
            # ">> Manual override >>"
            n599 = Dequeue Element(queue=w1838, timeout in ms (-1)=w1837, error in (no error)=w1839) -> (element=w1836:T1)  [unwired: 3 out]
            n600 = Equal?(x=w1835, y=u8 60) -> (x = y?=w1833:bool)
            n601 = case shown="\"Start Task 1\", Default" w1836 {
              tunnel: [w1849 State_Type_Definitions."True Stop" ("Enum")] -> w1840
              tunnel: [w1852 w1869] -> w1841
              tunnel: [State_Type_Definitions."Idle" ("Enum") State_Type_Definitions."Shutdown" ("Enum")] -> w1842
              tunnel: w1833 -> [w1848 _]
              tunnel: w1832 -> [w1847 _]
              tunnel: w1831 -> [w1843 w1866]
              frame "Start Task 1", Default {
                # "Stays in Task 5_A until stepper reaches desired \nheight"
                # "T: Go back to idle, F: Continue with task\""
                # ">> Manual override >>"
                n602 = case shown="True" w1848 {
                  tunnel: [w1856 w1862] -> w1852
                  tunnel: w1843 -> [w1854 w1860]
                  frame False {
                    n603 = for {
                      tunnel: string[] ["Z STEPPER CAM HEIGHT", "READ STEPPER VALUES"] ("element") -> [w1857] mode=indexing
                      shift-right: [w1859] -> w1856
                      shift-left: w1854 -> [w1858]
                      n604 = Enqueue Element(queue=w1858, element=w1857) -> (queue out=w1859:refnum<queue>)  [unwired: 2 in, 2 out]
                    }
                  }
                  frame True {
                    n605 = for {
                      shift-right: [w1864] -> w1862
                      shift-left: w1860 -> [w1865]
                      tunnel: string[] ["CAM CLOSE", "DISPOSE CAM BUFFERS", "DISPOSE PROC BUFFERS", "RESET ENCODERS"] -> [w1863] mode=indexing
                      n606 = Enqueue Element(queue=w1865, element=w1863) -> (queue out=w1864:refnum<queue>)  [unwired: 2 in, 2 out]
                    }
                  }
                }
                n607 = Or(x=w1848, y=w1847) -> (x .or. y?=w1850:bool)
                n608 = Select(t=State_Type_Definitions."True Stop" ("Enum"), s=w1847, f=State_Type_Definitions."True Stop" ("Enum")) -> (s? t:f=w1844:T10)
                n609 = Select(t=w1844, s=w1850, f=State_Type_Definitions."Task 8K: RAISE MY SWORD" ("Enum")) -> (s? t:f=w1849:T10)
              }
              frame "Exit" {
                n610 = for {
                  shift-right: [w1872] -> w1869
                  shift-left: w1866 -> [w1873]
                  tunnel: string[] ["STOP", "RESET ENCODERS", "RESET YAW", "ARDUINO MODE 0"] -> [w1871] mode=indexing
                  n611 = Enqueue Element(queue=w1873, element=w1871) -> (queue out=w1872:refnum<queue>)  [unwired: 2 in, 2 out]
                }
              }
            }
          }
          frame 38 {
            # ">> Stepper height reeached >>"
            # ">>> yStepper command>>>"
            # ">> Manual override >>"
            n612 = Dequeue Element(queue=w1885, timeout in ms (-1)=w1880, error in (no error)=w1884) -> (element=w1888:T1)  [unwired: 3 out]
            n613 = Equal?(x=w1882, y=u8 40) -> (x = y?=w1886:bool)
            n614 = case shown="\"Start Task 1\", Default" w1888 {
              tunnel: [w1899 State_Type_Definitions."True Stop" ("Enum")] -> w1878
              tunnel: [w1897 w1914] -> w1877
              tunnel: w1881 -> [w1896 _]
              tunnel: w1883 -> [w1890 _]
              tunnel: [State_Type_Definitions."Idle" ("Enum") State_Type_Definitions."Shutdown" ("Enum")] -> w1879
              tunnel: w1886 -> [w1889 _]
              frame "Start Task 1", Default {
                # ">> WIill proceed to part ii if not manual override >>"
                # ">>If ENABLE or Trigger is set to true>>"
                n615 = Or(x=w1889, y=w1890) -> (x .or. y?=w1891:bool)
                n616 = case shown="False" w1889 {
                  tunnel: [w1902 w1908] -> w1897
                  tunnel: w1896 -> [w1901 w1907]
                  frame False {
                    n617 = for {
                      shift-right: [w1904] -> w1902
                      shift-left: w1901 -> [w1905]
                      tunnel: string[] ["Z STEPPER BOX HEIGHT", "READ STEPPER VALUES"] ("element") -> [w1903] mode=indexing
                      n618 = Enqueue Element(queue=w1905, element=w1903) -> (queue out=w1904:refnum<queue>)  [unwired: 2 in, 2 out]
                    }
                  }
                  frame True {
                    n619 = for {
                      shift-right: [w1910] -> w1908
                      shift-left: w1907 -> [w1911]
                      tunnel: string[] ["ARDUINO - ULTRASONIC", "READ ULTRASONIC", "", "", "", ""] -> [w1909] mode=indexing
                      n620 = Enqueue Element(queue=w1911, element=w1909) -> (queue out=w1910:refnum<queue>)  [unwired: 2 in, 2 out]
                    }
                  }
                }
                n621 = Select(t=State_Type_Definitions."True Stop" ("Enum"), s=w1890, f=State_Type_Definitions."Task 9B: Rotate to Angle" ("Enum")) -> (s? t:f=w1893:T10)
                n622 = Select(t=w1893, s=w1891, f=State_Type_Definitions."Task 9A: Raise Arm" ("Enum")) -> (s? t:f=w1899:T10)
              }
              frame "Exit" {
                n623 = for {
                  shift-right: [w1917] -> w1914
                  shift-left: _ -> [w1918]
                  tunnel: string[] ["STOP", "RESET ENCODERS", "RESET YAW", ""] -> [w1916] mode=indexing
                  n624 = Enqueue Element(queue=w1918, element=w1916) -> (queue out=w1917:refnum<queue>)  [unwired: 2 in, 2 out]
                }
              }
            }
          }
          frame 39 {
            # ">>> yStepper command>>>"
            n625 = Dequeue Element(queue=w1932, timeout in ms (-1)=w1931, error in (no error)=w1930) -> (element=w1934:T1)  [unwired: 3 out]
            n626 = In Range and Coerce(upper limit=65.0, x=w1924, lower limit=55.0) -> (In Range?=w1921:bool)  [unwired: 1 out]
            n627 = case shown="\"Start Task 1\", Default" w1934 {
              tunnel: w1925 -> [w1937 _]
              tunnel: [w1945 State_Type_Definitions."True Stop" ("Enum")] -> w1927
              tunnel: w1933 -> [w1943 w1961]
              tunnel: [w1942 w1960] -> w1926
              tunnel: [State_Type_Definitions."Idle" ("Enum") State_Type_Definitions."Shutdown" ("Enum")] -> w1928
              tunnel: w1921 -> [w1935 _]
              frame "Start Task 1", Default {
                n628 = Or(x=w1935, y=w1937) -> (x .or. y?=w1936:bool)
                n629 = case shown="True" w1935 {
                  tunnel: w1943 -> [w1948 w1954]
                  tunnel: [w1947 w1952] -> w1942
                  frame False {
                    n630 = for {
                      shift-right: [w1950] -> w1947
                      shift-left: w1948 -> [w1951]
                      tunnel: string[] ["READ NAVX", "R-ACW"] ("element") -> [w1949] mode=indexing
                      n631 = Enqueue Element(queue=w1951, element=w1949) -> (queue out=w1950:refnum<queue>)  [unwired: 2 in, 2 out]
                    }
                  }
                  frame True {
                    n632 = for {
                      shift-right: [w1956] -> w1952
                      shift-left: w1954 -> [w1957]
                      tunnel: string[] ["STOP", "RESET ENCODERS", "RESET YAW", ""] -> [w1955] mode=indexing
                      n633 = Enqueue Element(queue=w1957, element=w1955) -> (queue out=w1956:refnum<queue>)  [unwired: 2 in, 2 out]
                    }
                  }
                }
                n634 = Select(t=State_Type_Definitions."True Stop" ("Enum"), s=w1937, f=State_Type_Definitions."Task 9C: Rotation alignmnet") -> (s? t:f=w1939:u16)
                n635 = Select(t=w1939, s=w1936, f=State_Type_Definitions."Task 9B: Rotate to Angle" ("Enum")) -> (s? t:f=w1945:u16)
              }
              frame "Exit" {
                n636 = for {
                  shift-right: [w1964] -> w1960
                  shift-left: w1961 -> [w1965]
                  tunnel: string[] ["STOP", "RESET ENCODERS", "RESET YAW", ""] -> [w1963] mode=indexing
                  n637 = Enqueue Element(queue=w1965, element=w1963) -> (queue out=w1964:refnum<queue>)  [unwired: 2 in, 2 out]
                }
              }
            }
          }
          frame 39 {
            # ">>> Motor control cluster >>>"
            # ">>Line Detected>>"
            # ">>Action Queue>>"
            # ">>> yStepper command>>>"
            n638 = Dequeue Element(queue=w1977, timeout in ms (-1)=w1976, error in (no error)=w1975) -> (element=w1978:T1)  [unwired: 3 out]
            n639 = case shown="\"Start Task 1\", Default" w1978 {
              tunnel: w1973 -> [w1979 _]
              tunnel: [w1989 State_Type_Definitions."True Stop" ("Enum")] -> w1970
              tunnel: w1974 -> [w1987 w2005]
              tunnel: [w1986 w2004] -> w1969
              tunnel: [State_Type_Definitions."Idle" ("Enum") State_Type_Definitions."Shutdown" ("Enum")] -> w1972
              tunnel: w1967 -> [w1980 _]
              frame "Start Task 1", Default {
                n640 = Or(x=w1979, y=w1980) -> (x .or. y?=w1981:bool)
                n641 = case shown="True" w1980 {
                  tunnel: w1987 -> [w1992 w1998]
                  tunnel: [w1991 w1996] -> w1986
                  frame False {
                    n642 = for {
                      shift-right: [w1994] -> w1991
                      shift-left: w1992 -> [w1995]
                      tunnel: string[] ["READ IR", "READ LINE SENSOR", "FORWARD - IR ASSIST"] ("element") -> [w1993] mode=indexing
                      n643 = Enqueue Element(queue=w1995, element=w1993) -> (queue out=w1994:refnum<queue>)  [unwired: 2 in, 2 out]
                    }
                  }
                  frame True {
                    n644 = for {
                      shift-right: [w2000] -> w1996
                      shift-left: w1998 -> [w2001]
                      tunnel: string[] ["STOP", "RESET ENCODERS", "RESET YAW", ""] -> [w1999] mode=indexing
                      n645 = Enqueue Element(queue=w2001, element=w1999) -> (queue out=w2000:refnum<queue>)  [unwired: 2 in, 2 out]
                    }
                  }
                }
                n646 = Select(t=State_Type_Definitions."True Stop" ("Enum"), s=w1979, f=State_Type_Definitions."Task 9D: Move Forward") -> (s? t:f=w1983:u16)
                n647 = Select(t=w1983, s=w1981, f=State_Type_Definitions."Task 9C: Rotation alignmnet" ("Enum")) -> (s? t:f=w1989:u16)
              }
              frame "Exit" {
                n648 = for {
                  shift-right: [w2008] -> w2004
                  shift-left: w2005 -> [w2009]
                  tunnel: string[] ["STOP", "RESET ENCODERS", "RESET YAW", ""] -> [w2007] mode=indexing
                  n649 = Enqueue Element(queue=w2009, element=w2007) -> (queue out=w2008:refnum<queue>)  [unwired: 2 in, 2 out]
                }
              }
            }
          }
          frame 40 {
            # ">> Manual override >>"
            # ">>Table Detected>>"
            # ">>> Motor control cluster >>>"
            # ">>Line Detected>>"
            # ">>Action Queue>>"
            # ">>> yStepper command>>>"
            n650 = Less Or Equal?(x=w2012, y=15.0) -> (x <= y?=w2011:bool)
            n651 = Dequeue Element(queue=w2023, timeout in ms (-1)=w2022, error in (no error)=w2021) -> (element=w2024:T1)  [unwired: 3 out]
            n652 = case shown="\"Start Task 1\", Default" w2024 {
              tunnel: w2019 -> [w2025 _]
              tunnel: [w2035 State_Type_Definitions."True Stop" ("Enum")] -> w2016
              tunnel: w2020 -> [w2033 w2051]
              tunnel: [w2032 w2050] -> w2015
              tunnel: [State_Type_Definitions."Idle" ("Enum") State_Type_Definitions."Shutdown" ("Enum")] -> w2018
              tunnel: w2011 -> [w2026 _]
              frame "Start Task 1", Default {
                n653 = Or(x=w2025, y=w2026) -> (x .or. y?=w2027:bool)
                n654 = case shown="True" w2026 {
                  tunnel: w2033 -> [w2038 w2044]
                  tunnel: [w2037 w2042] -> w2032
                  frame False {
                    n655 = for {
                      shift-right: [w2040] -> w2037
                      shift-left: w2038 -> [w2041]
                      tunnel: string[] ["READ IR", "FORWARD - IR ASSIST", ""] ("element") -> [w2039] mode=indexing
                      n656 = Enqueue Element(queue=w2041, element=w2039) -> (queue out=w2040:refnum<queue>)  [unwired: 2 in, 2 out]
                    }
                  }
                  frame True {
                    n657 = for {
                      shift-right: [w2046] -> w2042
                      shift-left: w2044 -> [w2047]
                      tunnel: string[] ["STOP", "RESET ENCODERS", "RESET YAW", ""] -> [w2045] mode=indexing
                      n658 = Enqueue Element(queue=w2047, element=w2045) -> (queue out=w2046:refnum<queue>)  [unwired: 2 in, 2 out]
                    }
                  }
                }
                n659 = Select(t=State_Type_Definitions."True Stop" ("Enum"), s=w2025, f=State_Type_Definitions."Task 9E: MOVE LEFT") -> (s? t:f=w2029:T10)
                n660 = Select(t=w2029, s=w2027, f=State_Type_Definitions."Task 9D: Move Forward" ("Enum")) -> (s? t:f=w2035:u16)
              }
              frame "Exit" {
                n661 = for {
                  shift-right: [w2054] -> w2050
                  shift-left: w2051 -> [w2055]
                  tunnel: string[] ["STOP", "RESET ENCODERS", "RESET YAW", ""] -> [w2053] mode=indexing
                  n662 = Enqueue Element(queue=w2055, element=w2053) -> (queue out=w2054:refnum<queue>)  [unwired: 2 in, 2 out]
                }
              }
            }
          }
          frame 42 {
            # ">> Reached distance?>>"
            # ">> Manual override >>"
            # ">>> Motor control cluster >>>"
            # ">>Action Queue>>"
            # ">>> yStepper command>>>"
            n663 = Dequeue Element(queue=w2069, timeout in ms (-1)=w2068, error in (no error)=w2067) -> (element=w2070:T1)  [unwired: 3 out]
            n664 = Less Or Equal?(x=w2059, y=-25.0) -> (x <= y?=w2057:bool)
            "Distance reached?" <- w2057
            n665 = case shown="\"Start Task 1\", Default" w2070 {
              tunnel: w2065 -> [w2071 _]
              tunnel: [w2081 State_Type_Definitions."True Stop" ("Enum")] -> w2062
              tunnel: w2066 -> [w2079 w2097]
              tunnel: [w2078 w2096] -> w2061
              tunnel: [State_Type_Definitions."Idle" ("Enum") State_Type_Definitions."Shutdown" ("Enum")] -> w2064
              tunnel: w2057 -> [w2072 _]
              frame "Start Task 1", Default {
                n666 = Or(x=w2071, y=w2072) -> (x .or. y?=w2073:bool)
                n667 = case shown="False" w2072 {
                  tunnel: w2079 -> [w2084 w2090]
                  tunnel: [w2083 w2088] -> w2078
                  frame False {
                    n668 = for {
                      shift-right: [w2086] -> w2083
                      shift-left: w2084 -> [w2087]
                      tunnel: string[] ["LEFT", "READ NAVX", "READ ENCODERS"] ("element") -> [w2085] mode=indexing
                      n669 = Enqueue Element(queue=w2087, element=w2085) -> (queue out=w2086:refnum<queue>)  [unwired: 2 in, 2 out]
                    }
                  }
                  frame True {
                    n670 = for {
                      shift-right: [w2092] -> w2088
                      shift-left: w2090 -> [w2093]
                      tunnel: string[] ["STOP", "RESET ENCODERS", "RESET YAW", ""] -> [w2091] mode=indexing
                      n671 = Enqueue Element(queue=w2093, element=w2091) -> (queue out=w2092:refnum<queue>)  [unwired: 2 in, 2 out]
                    }
                  }
                }
                n672 = Select(t=State_Type_Definitions."True Stop" ("Enum"), s=w2071, f=State_Type_Definitions."True Stop") -> (s? t:f=w2075:T10)
                n673 = Select(t=w2075, s=w2073, f=State_Type_Definitions."Task 9E: MOVE LEFT" ("Enum")) -> (s? t:f=w2081:T10)
              }
              frame "Exit" {
                n674 = for {
                  shift-right: [w2100] -> w2096
                  shift-left: w2097 -> [w2101]
                  tunnel: string[] ["STOP", "RESET ENCODERS", "RESET YAW", ""] -> [w2099] mode=indexing
                  n675 = Enqueue Element(queue=w2101, element=w2099) -> (queue out=w2100:refnum<queue>)  [unwired: 2 in, 2 out]
                }
              }
            }
          }
          frame 42 {
            # ">> Stepper height reeached >>"
            # ">>> yStepper command>>>"
            # ">> Manual override >>"
            n676 = Dequeue Element(queue=w2113, timeout in ms (-1)=w2108, error in (no error)=w2112) -> (element=w2116:T1)  [unwired: 3 out]
            n677 = Equal?(x=w2110, y=u8 40) -> (x = y?=w2114:bool)
            n678 = case shown="\"Start Task 1\", Default" w2116 {
              tunnel: [w2127 State_Type_Definitions."True Stop" ("Enum")] -> w2106
              tunnel: [w2125 w2143] -> w2105
              tunnel: w2109 -> [w2124 w2140]
              tunnel: w2111 -> [w2118 _]
              tunnel: [State_Type_Definitions."Idle" ("Enum") State_Type_Definitions."Shutdown" ("Enum")] -> w2107
              tunnel: w2114 -> [w2117 _]
              frame "Start Task 1", Default {
                # ">> WIill proceed to part ii if not manual override >>"
                # ">>If ENABLE or Trigger is set to true>>"
                n679 = Or(x=w2117, y=w2118) -> (x .or. y?=w2119:bool)
                n680 = case shown="False" w2117 {
                  tunnel: [w2130 w2136] -> w2125
                  tunnel: w2124 -> [w2129 w2135]
                  frame False {
                    n681 = for {
                      shift-right: [w2132] -> w2130
                      shift-left: w2129 -> [w2133]
                      tunnel: string[] ["Z STEPPER BOX HEIGHT", "READ STEPPER VALUES"] ("element") -> [w2131] mode=indexing
                      n682 = Enqueue Element(queue=w2133, element=w2131) -> (queue out=w2132:refnum<queue>)  [unwired: 2 in, 2 out]
                    }
                  }
                  frame True {
                    n683 = for {
                      shift-right: [w2138] -> w2136
                      shift-left: w2135 -> [w2139]
                      tunnel: string[] ["READ IR", "", "", "", "", ""] -> [w2137] mode=indexing
                      n684 = Enqueue Element(queue=w2139, element=w2137) -> (queue out=w2138:refnum<queue>)  [unwired: 2 in, 2 out]
                    }
                  }
                }
                n685 = Select(t=State_Type_Definitions."True Stop" ("Enum"), s=w2118, f=State_Type_Definitions."Task A: MOVE FORWARD" ("Enum")) -> (s? t:f=w2121:u16)
                n686 = Select(t=w2121, s=w2119, f=State_Type_Definitions."Task A: RAISE ARM TO HEIGHT" ("Enum")) -> (s? t:f=w2127:u16)
              }
              frame "Exit" {
                n687 = for {
                  shift-right: [w2146] -> w2143
                  shift-left: w2140 -> [w2147]
                  tunnel: string[] ["STOP", "RESET ENCODERS", "RESET YAW", ""] -> [w2145] mode=indexing
                  n688 = Enqueue Element(queue=w2147, element=w2145) -> (queue out=w2146:refnum<queue>)  [unwired: 2 in, 2 out]
                }
              }
            }
          }
          frame 43 {
            # ">>> Motor control cluster >>>"
            # ">>> yStepper command>>>"
            # ">>Object detected>>"
            n689 = Dequeue Element(queue=w2157, timeout in ms (-1)=w2156, error in (no error)=w2155) -> (element=w2162:T1)  [unwired: 3 out]
            n690 = Less Or Equal?(x=w2151, y=30.0) -> (x <= y?=w2149:bool)
            "Table obstruct" <- w2149
            n691 = case shown="\"Start Task 1\", Default" w2162 {
              tunnel: w2149 -> [w2165 _]
              tunnel: [w2172 State_Type_Definitions."True Stop" ("Enum")] -> w2161
              tunnel: w2154 -> [w2164 _]
              tunnel: w2158 -> [w2171 w2188]
              tunnel: [w2170 w2189] -> w2160
              tunnel: [State_Type_Definitions."Idle" ("Enum") State_Type_Definitions."Shutdown" ("Enum")] -> w2159
              frame "Start Task 1", Default {
                n692 = case shown="False" w2165 {
                  tunnel: w2171 -> [w2175 w2182]
                  tunnel: [w2176 w2181] -> w2170
                  frame False {
                    n693 = for {
                      tunnel: string[] ["READ IR", "FORWARD", "READ NAVX"] ("element") -> [w2177] mode=indexing
                      shift-right: [w2179] -> w2176
                      shift-left: w2175 -> [w2178]
                      n694 = Enqueue Element(queue=w2178, element=w2177) -> (queue out=w2179:refnum<queue>)  [unwired: 2 in, 2 out]
                    }
                  }
                  frame True {
                    n695 = for {
                      shift-right: [w2184] -> w2181
                      shift-left: w2182 -> [w2185]
                      tunnel: string[] ["RESET ENCODERS", "READ NAVX", "READ ENCODERS"] -> [w2183] mode=indexing
                      n696 = Enqueue Element(queue=w2185, element=w2183) -> (queue out=w2184:refnum<queue>)  [unwired: 2 in, 2 out]
                    }
                  }
                }
                n697 = Or(x=w2165, y=w2164) -> (x .or. y?=w2163:bool)
                n698 = Select(t=State_Type_Definitions."True Stop" ("Enum"), s=w2164, f=State_Type_Definitions."True Stop" ("Enum")) -> (s? t:f=w2166:T10)
                n699 = Select(t=w2166, s=w2163, f=State_Type_Definitions."Task A: MOVE FORWARD" ("Enum")) -> (s? t:f=w2172:u16)
              }
              frame "Exit" {
                n700 = for {
                  shift-right: [w2192] -> w2189
                  shift-left: w2188 -> [w2193]
                  tunnel: string[] ["STOP", "RESET ENCODERS", "RESET YAW", "ARDUINO MODE 0"] -> [w2191] mode=indexing
                  n701 = Enqueue Element(queue=w2193, element=w2191) -> (queue out=w2192:refnum<queue>)  [unwired: 2 in, 2 out]
                }
              }
            }
          }
        }
        "Object Detection" <- w291
      }
    }
    "Object recognition mode" <- w203
    n702 = local write "Green LED"(w213) -> ()
  }
  n703 = while {
    stop <- w2901 stop-if-true
    n704 = call "MOTOR CONTROL WITH PID AE.vi"("AE Mode"=MOTOR_CONTROL_WITH_PID_AE_DATA_MODE_TYPE_DEF."Read from AE") -> ("Speed & distance"=→"Speed & distance":T6)  [unwired: 3 in]
    n705 = call "FGV Bool.vi"("Init/Read/Write State"=States_for_Action_Engine."Read") -> ("Output node"=w2901:bool)  [unwired: 2 in, 1 out]
    n706 = Wait (ms)(milliseconds to wait=u32 5) -> ()  [unwired: 1 out]
  }
  n707 = while {
    stop <- w2906 stop-if-true
    n708 = call <vilib>:"RT Get CPU Loads.vi"() -> ("CPU loads"=→"CPU loads":T9[])  [unwired: 10 in, 1 out]
    n709 = Wait (ms)(milliseconds to wait=u32 100) -> ()  [unwired: 1 out]
    n710 = call "FGV Bool.vi"("Init/Read/Write State"=States_for_Action_Engine."Read") -> ("Output node"=w2906:bool)  [unwired: 2 in, 1 out]
  }
  n711 = call <vilib>:"DIO Close.vi"("error in (no error)"=w22, "DIO Info In"=w25) -> ()  [unwired: 9 in, 1 out]
  n712 = call <vilib>:"DIO Close.vi"("error in (no error)"=w32, "DIO Info In"=w34) -> ()  [unwired: 9 in, 1 out]
  n713 = call <vilib>:"NavX Close.vi"("error in (no error)"=w9, "NavX Info In"=w8) -> ()  [unwired: 9 in, 1 out]
  n714 = call <vilib>:"DIO Close.vi"("error in (no error)"=w27, "DIO Info In"=w29) -> ()  [unwired: 9 in, 1 out]
  n715 = call <vilib>:"DIO Close.vi"("error in (no error)"=w16, "DIO Info In"=w17) -> ()  [unwired: 9 in, 1 out]
  n716 = call <vilib>:"DIO Close.vi"("error in (no error)"=w11, "DIO Info In"=w12) -> ()  [unwired: 9 in, 1 out]
  n717 = Merge Errors "Merge Errors"(w62, w61) -> (w44:errorcluster)
  n718 = Merge Errors(w48, w44) -> (w43:errorcluster)
  n719 = Destroy User Event(user event=w66, error in=w43) -> ()  [unwired: 1 out]
  n720 = Release Queue(queue=w39, error in (no error)=w43) -> (error out=→"Queue Errors":errorcluster)  [unwired: 1 in, 2 out]
  n721 = Release Queue(queue=w56, error in (no error)=w43) -> ()  [unwired: 1 in, 3 out]
  n722 = Destroy User Event(user event=w65, error in=w43) -> ()  [unwired: 1 out]
  n723 = Unregister For Events(event registration refnum=w57, error in=w43) -> ()  [unwired: 1 out]
